vi "QUIZ#2.vi"() -> ()   [LabVIEW 2020]
uses:
  <vilib>/Utility/miscctls.llb/LVBoundsTypeDef.ctl
  <vilib>/Utility/miscctls.llb/LVPositionTypeDef.ctl
  Control 2.ctl
panel:
  out "String":string
  out "DISCO 6":bool
  out "Numeric 2":dbl
  out "x-y":ext
  in  "Array":dbl[](array[numeric])
  out "Bounds 4":T1
  out "x*y 2":u32
  in  "NUMERO DISCOS":T2
  out "Position 5":T3
  out "Position 4":T3
  out "Position 3":T3
  out "Position 2":T3
  out "Position":T3
  out "DISCO 1":bool
  out "DISCO 2":bool
  in  "Boolean 2":bool
  in  "Boolean":bool
  in  "s 2":bool
  out "Bounds 3":T1
  out "DISCO 3":bool
  out "DISCO 4":bool
  out "Bounds":T1
  in  "s":bool
  out "DISCO 5":bool
  out "DESTINO 3":bool
  out "DESTINO":bool
  out "DESTINO 2":bool
  # "NUMERO DE DISCOS ="
  # "NUMERO DE MOVIMIENTOS MINIMOS="
  # "TU NUMERO DE MOVIMIENTOS="
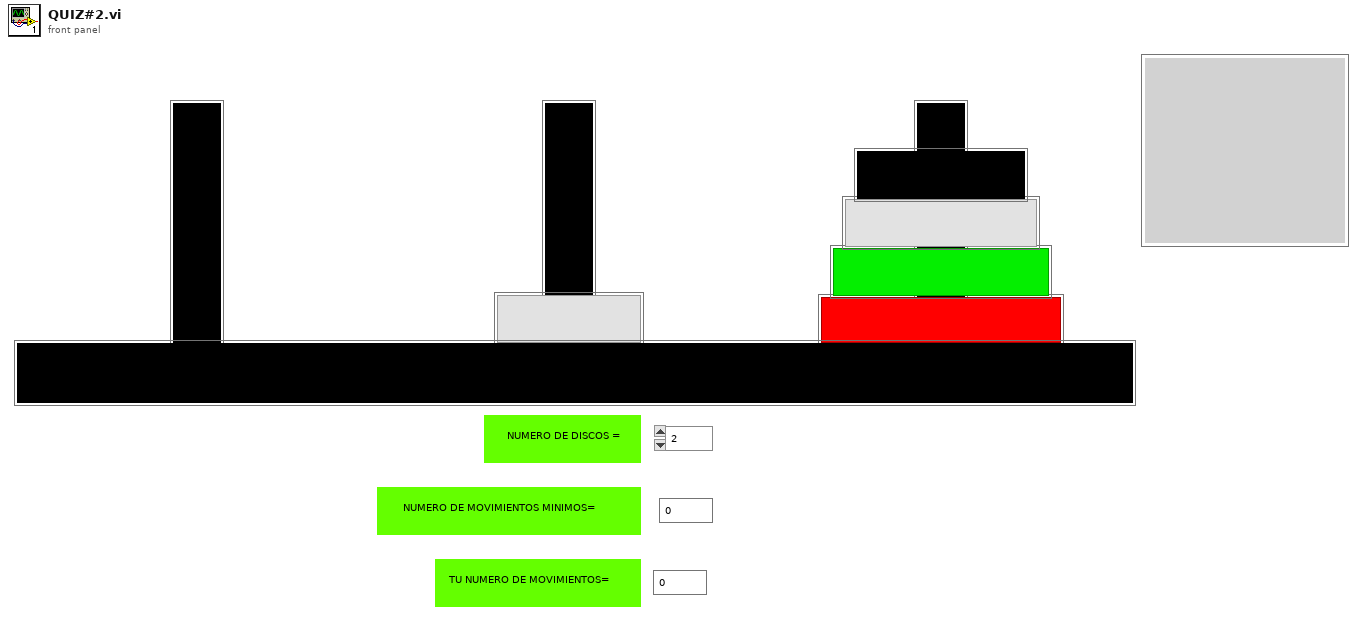
[diagram p1: front panel]
types:
  T1 = typedef "LVBoundsTypeDef.ctl" = cluster{"Width":u32, "Height":u32}
  T2 = typedef "Control 2.ctl" = enum16{"2", "3", "4", "5"}
  T3 = typedef "LVPositionTypeDef.ctl" = cluster{"Left":i32, "Top":i32}
  T4 = typedef "LVPoint32TypeDef.ctl" = cluster{"Horizontal":i32, "Vertical":i32}
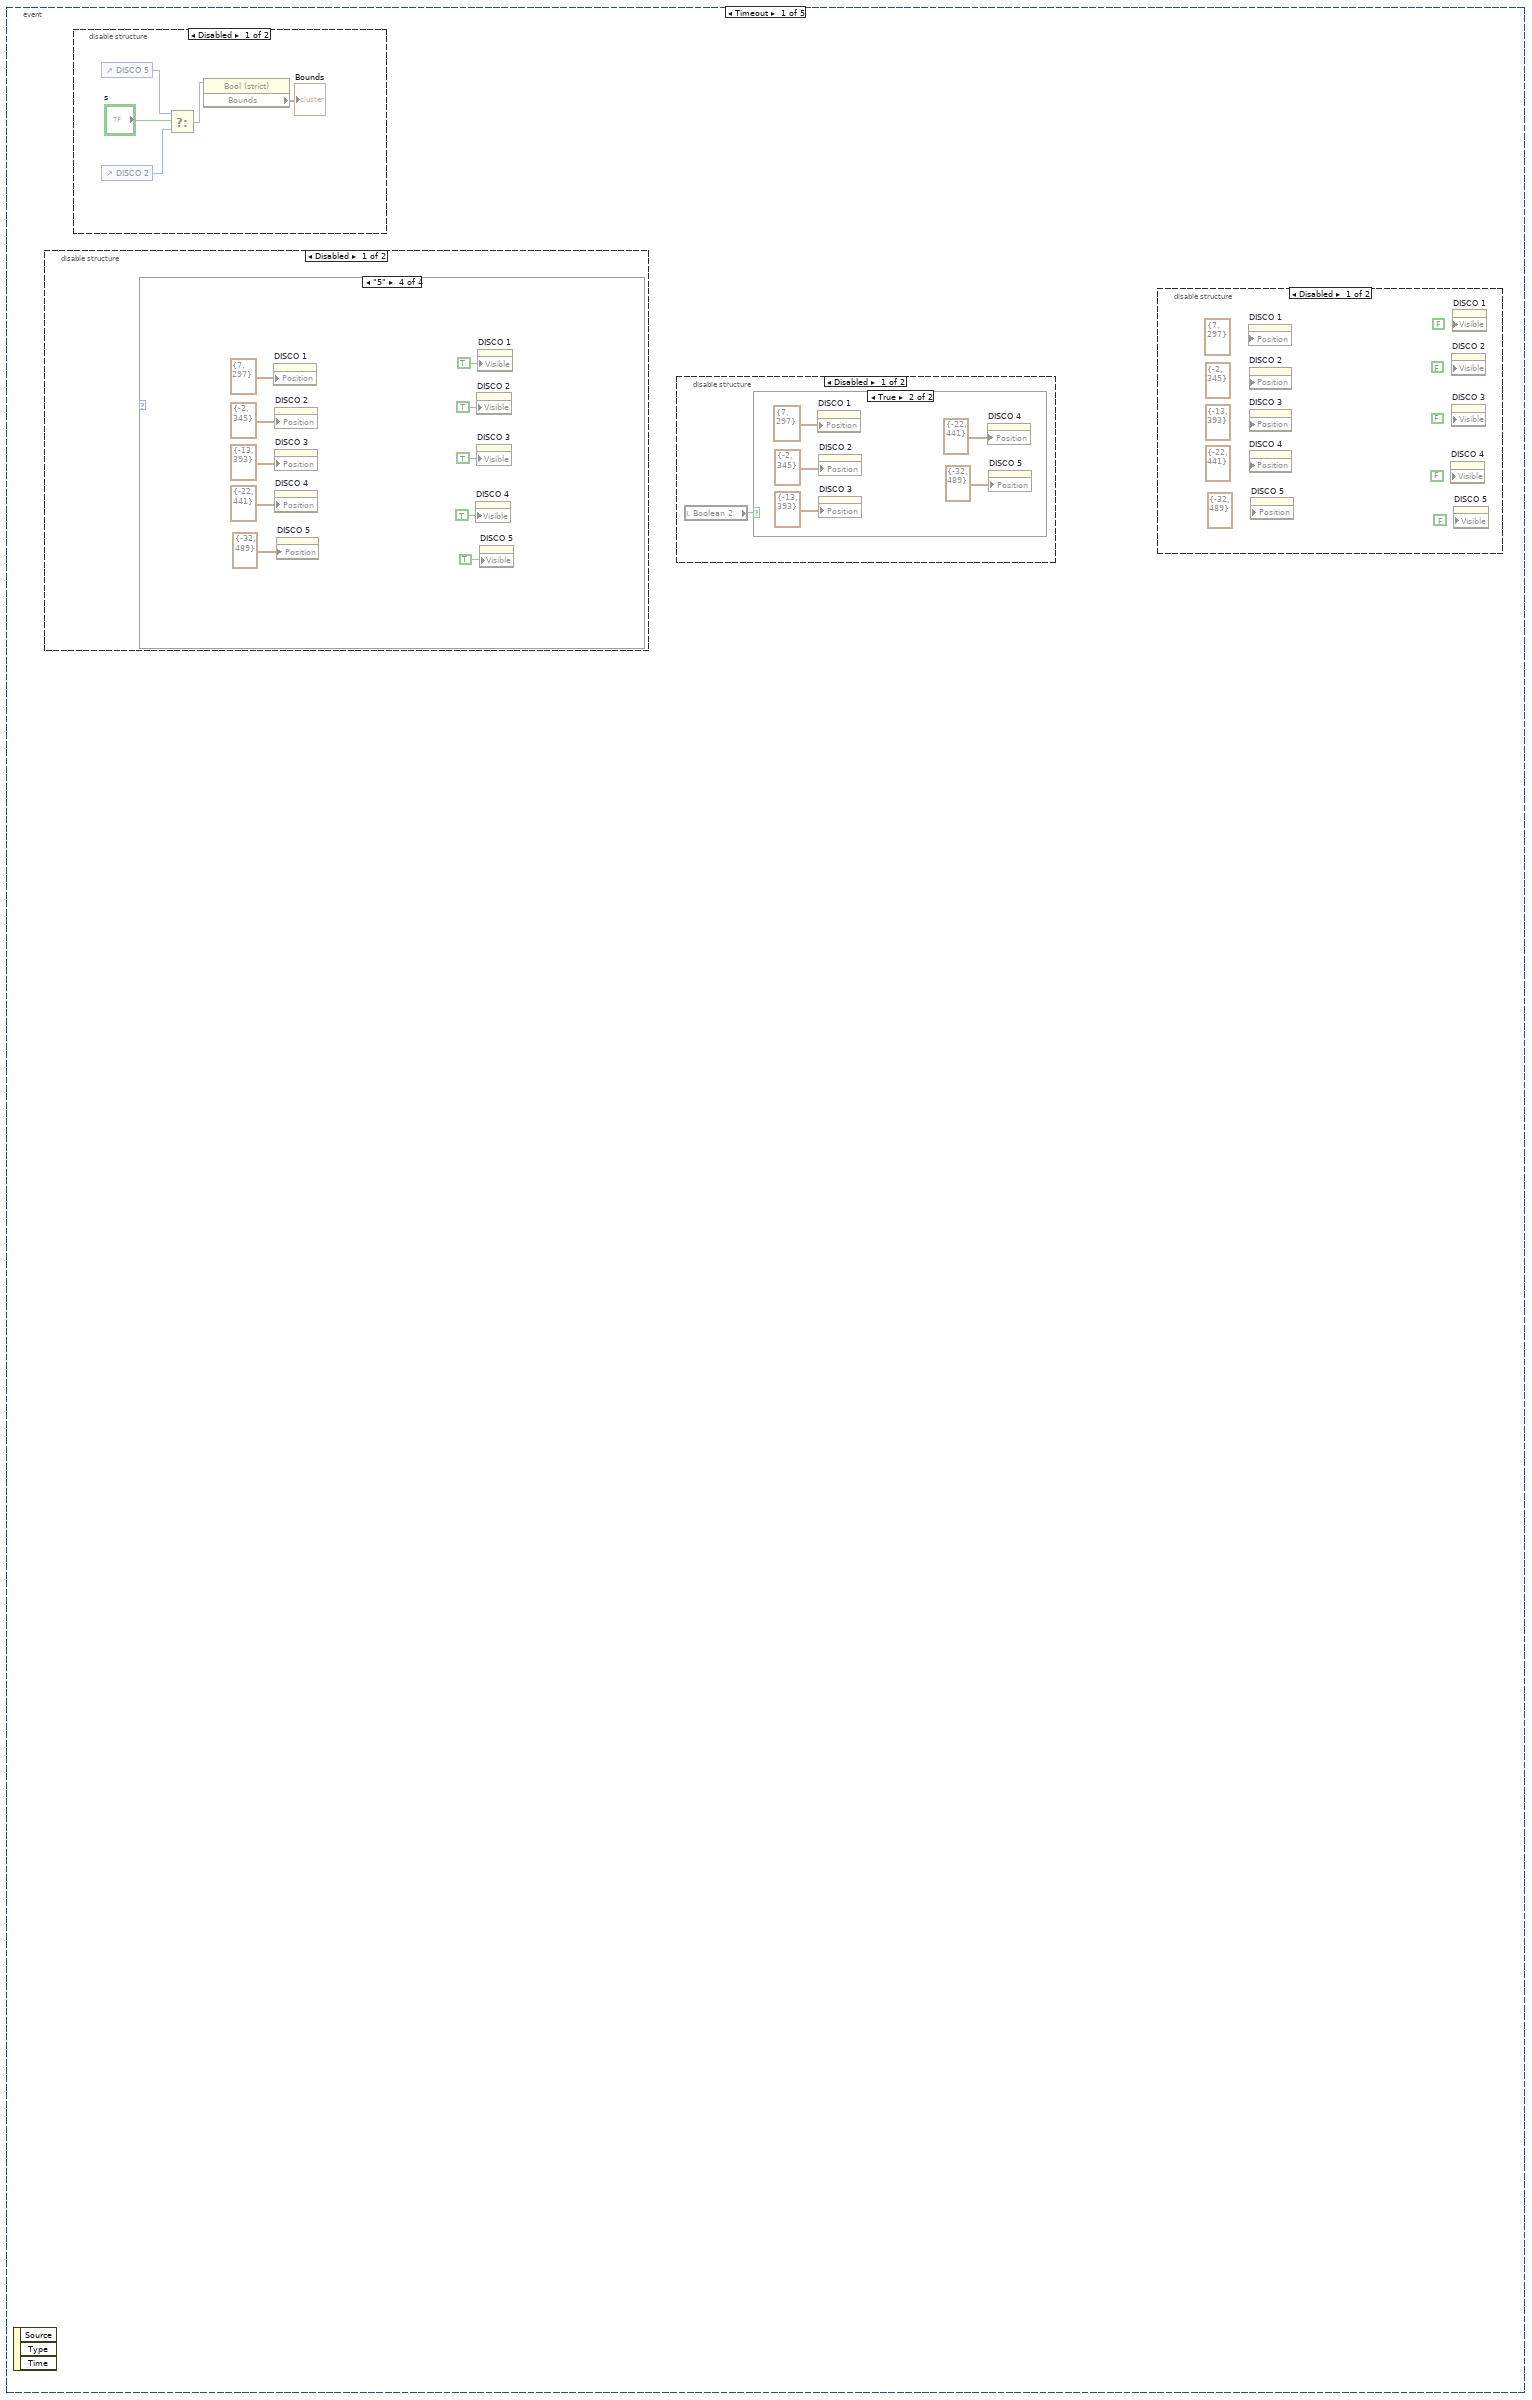
[diagram p7: hidden frame]
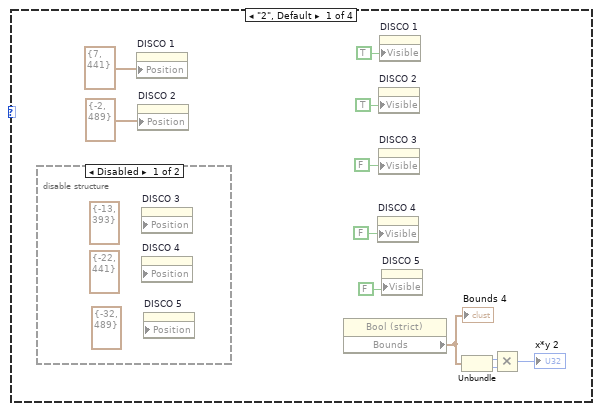
[diagram p9: hidden frame]
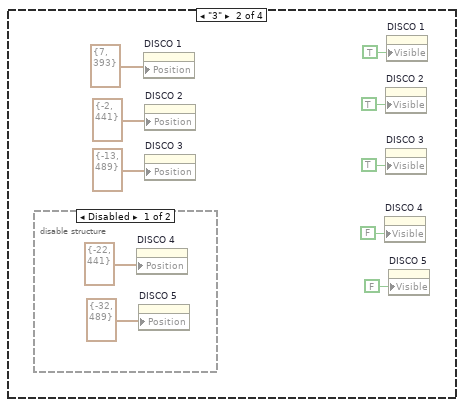
[diagram p11: hidden frame]
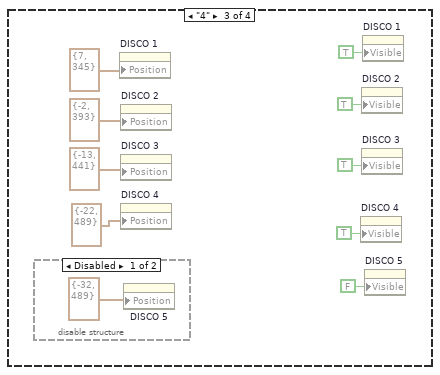
[diagram p13: hidden frame]
diagram:
  (unwired) Control_2."2"
  n1 = disable-structure shown="Disabled" {
    frame Disabled {
      n2 = property on="DISCO 1" class="Bool (strict)"() -> ("Position"=→"Position":T3)  [unwired: 2 in, 2 out]
      n3 = property on="DISCO 2" class="Bool (strict)"() -> ("Position"=→"Position 2":T3)  [unwired: 2 in, 2 out]
      n4 = property on="DISCO 3" class="Bool (strict)"() -> ("Position"=→"Position 3":T3)  [unwired: 2 in, 2 out]
      n5 = property on="DISCO 4" class="Bool (strict)"() -> ("Position"=→"Position 4":T3)  [unwired: 2 in, 2 out]
      n6 = property on="DISCO 5" class="Bool (strict)"() -> ("Position"=→"Position 5":T3)  [unwired: 2 in, 2 out]
      n7 = property on="DISCO 1" class="Bool (strict)"("Position"=T3 {"Left"=381, "Top"=297}) -> ()  [unwired: 2 in, 2 out]
      n8 = property on="DISCO 2" class="Bool (strict)"("Position"=T3 {"Left"=369, "Top"=345}) -> ()  [unwired: 2 in, 2 out]
      n9 = property on="DISCO 3" class="Bool (strict)"("Position"=T3 {"Left"=357, "Top"=393}) -> ()  [unwired: 2 in, 2 out]
      n10 = property on="DISCO 4" class="Bool (strict)"("Position"=T3 {"Left"=345, "Top"=441}) -> ()  [unwired: 2 in, 2 out]
      n11 = property on="DISCO 5" class="Bool (strict)"("Position"=T3 {"Left"=333, "Top"=489}) -> ()  [unwired: 2 in, 2 out]
    }
    frame Enabled {
    }
  }
  n12 = while {
    stop <- FALSE stop-if-true
    n13 = event shown="[1] \"DISCO 1\", \"DISCO 2\", \"DISCO 5\", \"DISCO 4\", \"DISCO 3\", \"DESTINO 3\", \"DESTINO 2\", \"DESTINO\": Mouse Up" {
      selector: _ -> [_ _ _ _ _]
      dyn-events: _ -> [_ _ _ _ _]
      timeout: 100 -> [_ _ _ _ _]
      event Timeout {
        n14 = event-data() -> ()  [unwired: 1 in, 3 out]
        n15 = disable-structure shown="Disabled" {
          frame Disabled {
            n16 = case shown="\"5\"" w14 {
              frame "2", Default {
                n17 = disable-structure shown="Disabled" {
                  frame Disabled {
                    (unwired) T3 {"Left"=-32, "Top"=489} ("Position")
                    (unwired) T3 {"Left"=-22, "Top"=441} ("Position")
                    (unwired) T3 {"Left"=-13, "Top"=393} ("Position")
                    n18 = property on="DISCO 3" class="Bool (strict)" props=["Position"]() -> ()  [unwired: 3 in, 2 out]
                    n19 = property on="DISCO 4" class="Bool (strict)" props=["Position"]() -> ()  [unwired: 3 in, 2 out]
                    n20 = property on="DISCO 5" class="Bool (strict)" props=["Position"]() -> ()  [unwired: 3 in, 2 out]
                  }
                  frame Enabled {
                  }
                }
                n21 = property on="DISCO 1" class="Bool (strict)"("Position"=T3 {"Left"=7, "Top"=441}) -> ()  [unwired: 2 in, 2 out]
                n22 = property on="DISCO 2" class="Bool (strict)"("Position"=T3 {"Left"=-2, "Top"=489}) -> ()  [unwired: 2 in, 2 out]
                n23 = property class="Bool (strict)"() -> ("Bounds"=w18:T1)  [unwired: 2 in, 2 out]
                "Bounds 4" <- w18
                n24 = property on="DISCO 4" class="Bool (strict)"("Visible"=FALSE) -> ()  [unwired: 2 in, 2 out]
                n25 = property on="DISCO 2" class="Bool (strict)"("Visible"=TRUE) -> ()  [unwired: 2 in, 2 out]
                n26 = property on="DISCO 3" class="Bool (strict)"("Visible"=FALSE) -> ()  [unwired: 2 in, 2 out]
                n27 = property on="DISCO 1" class="Bool (strict)"("Visible"=TRUE) -> ()  [unwired: 2 in, 2 out]
                n28 = property on="DISCO 5" class="Bool (strict)"("Visible"=FALSE) -> ()  [unwired: 2 in, 2 out]
                n29 = Unbundle(w18) -> ("Width"=w16:u32, "Height"=w15:u32)
                n30 = Multiply(x=w16, y=w15) -> (x*y=→"x*y 2":u32)
              }
              frame "3" {
                n31 = disable-structure shown="Disabled" {
                  frame Disabled {
                    n32 = property on="DISCO 4" class="Bool (strict)"("Position"=T3 {"Left"=-22, "Top"=441}) -> ()  [unwired: 2 in, 2 out]
                    n33 = property on="DISCO 5" class="Bool (strict)"("Position"=T3 {"Left"=-32, "Top"=489}) -> ()  [unwired: 2 in, 2 out]
                  }
                  frame Enabled {
                  }
                }
                n34 = property on="DISCO 1" class="Bool (strict)"("Position"=T3 {"Left"=7, "Top"=393}) -> ()  [unwired: 2 in, 2 out]
                n35 = property on="DISCO 2" class="Bool (strict)"("Position"=T3 {"Left"=-2, "Top"=441}) -> ()  [unwired: 2 in, 2 out]
                n36 = property on="DISCO 3" class="Bool (strict)"("Position"=T3 {"Left"=-13, "Top"=489}) -> ()  [unwired: 2 in, 2 out]
                n37 = property on="DISCO 4" class="Bool (strict)"("Visible"=FALSE) -> ()  [unwired: 2 in, 2 out]
                n38 = property on="DISCO 2" class="Bool (strict)"("Visible"=TRUE) -> ()  [unwired: 2 in, 2 out]
                n39 = property on="DISCO 3" class="Bool (strict)"("Visible"=TRUE) -> ()  [unwired: 2 in, 2 out]
                n40 = property on="DISCO 1" class="Bool (strict)"("Visible"=TRUE) -> ()  [unwired: 2 in, 2 out]
                n41 = property on="DISCO 5" class="Bool (strict)"("Visible"=FALSE) -> ()  [unwired: 2 in, 2 out]
              }
              frame "4" {
                n42 = disable-structure shown="Disabled" {
                  frame Disabled {
                    n43 = property on="DISCO 5" class="Bool (strict)"("Position"=T3 {"Left"=-32, "Top"=489}) -> ()  [unwired: 2 in, 2 out]
                  }
                  frame Enabled {
                  }
                }
                n44 = property on="DISCO 1" class="Bool (strict)"("Position"=T3 {"Left"=7, "Top"=345}) -> ()  [unwired: 2 in, 2 out]
                n45 = property on="DISCO 2" class="Bool (strict)"("Position"=T3 {"Left"=-2, "Top"=393}) -> ()  [unwired: 2 in, 2 out]
                n46 = property on="DISCO 3" class="Bool (strict)"("Position"=T3 {"Left"=-13, "Top"=441}) -> ()  [unwired: 2 in, 2 out]
                n47 = property on="DISCO 4" class="Bool (strict)"("Position"=T3 {"Left"=-22, "Top"=489}) -> ()  [unwired: 2 in, 2 out]
                n48 = property on="DISCO 4" class="Bool (strict)"("Visible"=TRUE) -> ()  [unwired: 2 in, 2 out]
                n49 = property on="DISCO 2" class="Bool (strict)"("Visible"=TRUE) -> ()  [unwired: 2 in, 2 out]
                n50 = property on="DISCO 3" class="Bool (strict)"("Visible"=TRUE) -> ()  [unwired: 2 in, 2 out]
                n51 = property on="DISCO 1" class="Bool (strict)"("Visible"=TRUE) -> ()  [unwired: 2 in, 2 out]
                n52 = property on="DISCO 5" class="Bool (strict)"("Visible"=FALSE) -> ()  [unwired: 2 in, 2 out]
              }
              frame "5" {
                n53 = property on="DISCO 1" class="Bool (strict)"("Position"=T3 {"Left"=7, "Top"=297}) -> ()  [unwired: 2 in, 2 out]
                n54 = property on="DISCO 2" class="Bool (strict)"("Position"=T3 {"Left"=-2, "Top"=345}) -> ()  [unwired: 2 in, 2 out]
                n55 = property on="DISCO 3" class="Bool (strict)"("Position"=T3 {"Left"=-13, "Top"=393}) -> ()  [unwired: 2 in, 2 out]
                n56 = property on="DISCO 4" class="Bool (strict)"("Position"=T3 {"Left"=-22, "Top"=441}) -> ()  [unwired: 2 in, 2 out]
                n57 = property on="DISCO 5" class="Bool (strict)"("Position"=T3 {"Left"=-32, "Top"=489}) -> ()  [unwired: 2 in, 2 out]
                n58 = property on="DISCO 4" class="Bool (strict)"("Visible"=TRUE) -> ()  [unwired: 2 in, 2 out]
                n59 = property on="DISCO 2" class="Bool (strict)"("Visible"=TRUE) -> ()  [unwired: 2 in, 2 out]
                n60 = property on="DISCO 3" class="Bool (strict)"("Visible"=TRUE) -> ()  [unwired: 2 in, 2 out]
                n61 = property on="DISCO 1" class="Bool (strict)"("Visible"=TRUE) -> ()  [unwired: 2 in, 2 out]
                n62 = property on="DISCO 5" class="Bool (strict)"("Visible"=TRUE) -> ()  [unwired: 2 in, 2 out]
              }
            }
          }
          frame Enabled {
          }
        }
        n63 = disable-structure shown="Disabled" {
          frame Disabled {
            n64 = control-ref of="DISCO 5"() -> (w66:refnum<vi>)
            n65 = control-ref of="DISCO 2"() -> (w65:refnum<vi>)
            n66 = Select(t=w66, s="s", f=w65) -> (s? t:f=w64:refnum<vi>)
            n67 = property on="Property Node" class="Bool (strict)"(reference=w64) -> ("Bounds"=→"Bounds":T1)  [unwired: 1 in, 2 out]
          }
          frame Enabled {
          }
        }
        n68 = disable-structure shown="Disabled" {
          frame Disabled {
            n69 = local read "Boolean 2"() -> (w56:bool)
            n70 = case shown="True" w56 {
              frame False {
              }
              frame True {
                n71 = property on="DISCO 1" class="Bool (strict)"("Position"=T3 {"Left"=7, "Top"=297}) -> ()  [unwired: 2 in, 2 out]
                n72 = property on="DISCO 2" class="Bool (strict)"("Position"=T3 {"Left"=-2, "Top"=345}) -> ()  [unwired: 2 in, 2 out]
                n73 = property on="DISCO 3" class="Bool (strict)"("Position"=T3 {"Left"=-13, "Top"=393}) -> ()  [unwired: 2 in, 2 out]
                n74 = property on="DISCO 4" class="Bool (strict)"("Position"=T3 {"Left"=-22, "Top"=441}) -> ()  [unwired: 2 in, 2 out]
                n75 = property on="DISCO 5" class="Bool (strict)"("Position"=T3 {"Left"=-32, "Top"=489}) -> ()  [unwired: 2 in, 2 out]
              }
            }
          }
          frame Enabled {
          }
        }
        n76 = disable-structure shown="Disabled" {
          frame Disabled {
            (unwired) FALSE ("Visible")
            (unwired) FALSE ("Visible")
            (unwired) FALSE ("Visible")
            (unwired) FALSE ("Visible")
            (unwired) FALSE ("Visible")
            (unwired) T3 {"Left"=-32, "Top"=489} ("Position")
            (unwired) T3 {"Left"=-22, "Top"=441} ("Position")
            (unwired) T3 {"Left"=-13, "Top"=393} ("Position")
            (unwired) T3 {"Left"=-2, "Top"=345} ("Position")
            (unwired) T3 {"Left"=7, "Top"=297} ("Position")
            n77 = property on="DISCO 1" class="Bool (strict)" props=["Position"]() -> ()  [unwired: 3 in, 2 out]
            n78 = property on="DISCO 2" class="Bool (strict)" props=["Position"]() -> ()  [unwired: 3 in, 2 out]
            n79 = property on="DISCO 3" class="Bool (strict)" props=["Position"]() -> ()  [unwired: 3 in, 2 out]
            n80 = property on="DISCO 4" class="Bool (strict)" props=["Position"]() -> ()  [unwired: 3 in, 2 out]
            n81 = property on="DISCO 5" class="Bool (strict)" props=["Position"]() -> ()  [unwired: 3 in, 2 out]
            n82 = property on="DISCO 4" class="Bool (strict)" props=["Visible"]() -> ()  [unwired: 3 in, 2 out]
            n83 = property on="DISCO 2" class="Bool (strict)" props=["Visible"]() -> ()  [unwired: 3 in, 2 out]
            n84 = property on="DISCO 3" class="Bool (strict)" props=["Visible"]() -> ()  [unwired: 3 in, 2 out]
            n85 = property on="DISCO 1" class="Bool (strict)" props=["Visible"]() -> ()  [unwired: 3 in, 2 out]
            n86 = property on="DISCO 5" class="Bool (strict)" props=["Visible"]() -> ()  [unwired: 3 in, 2 out]
          }
          frame Enabled {
          }
        }
      }
      event "DISCO 1", "DISCO 2", "DISCO 5", "DISCO 4", "DISCO 3", "DESTINO 3", "DESTINO 2", "DESTINO": Mouse Up {
        (unwired) 0 ("x")
        (unwired) 345 ("y")
        n87 = event-data() -> ()  [unwired: 1 in, 6 out]
        n88 = property on="DISCO 3" class="Bool (strict)"() -> ("Left"=w2294:i32, "Top"=w2302:i32)  [unwired: 2 in, 2 out]
        n89 = property on="DISCO 3" class="Bool (strict)"() -> ("Left"=w2311:i32, "Top"=w2303:i32)  [unwired: 2 in, 2 out]
        n90 = property on="DISCO 3" class="Bool (strict)"() -> ("Left"=w2320:i32, "Top"=w2328:i32)  [unwired: 2 in, 2 out]
        n91 = property on="DISCO 3" class="Bool (strict)"() -> ("Left"=w2337:i32, "Top"=w2329:i32)  [unwired: 2 in, 2 out]
        n92 = property on="DISCO 3" class="Bool (strict)"() -> ("Left"=w2346:i32, "Top"=w2354:i32)  [unwired: 2 in, 2 out]
        n93 = property on="DISCO 5" class="Bool (strict)"() -> ("Left"=w2415:i32, "Top"=w2407:i32)  [unwired: 2 in, 2 out]
        n94 = property on="DISCO 5" class="Bool (strict)"() -> ("Left"=w2398:i32, "Top"=w2406:i32)  [unwired: 2 in, 2 out]
        n95 = property on="DISCO 5" class="Bool (strict)"() -> ("Left"=w2389:i32, "Top"=w2381:i32)  [unwired: 2 in, 2 out]
        n96 = property on="DISCO 5" class="Bool (strict)"() -> ("Left"=w2372:i32, "Top"=w2380:i32)  [unwired: 2 in, 2 out]
        n97 = property on="DISCO 5" class="Bool (strict)"() -> ("Left"=w2363:i32, "Top"=w2355:i32)  [unwired: 2 in, 2 out]
        n98 = property on="DISCO 5" class="Bool (strict)"() -> ("Left"=w2424:i32, "Top"=w2432:i32)  [unwired: 2 in, 2 out]
        n99 = local write "Boolean"(FALSE ("Boolean 2")) -> ()
        n100 = property on="DISCO 5" class="Bool (strict)"() -> ("Left"=w2441:i32, "Top"=w2433:i32)  [unwired: 2 in, 2 out]
        n101 = property on="DISCO 5" class="Bool (strict)"() -> ("Left"=w2467:i32, "Top"=w2459:i32)  [unwired: 2 in, 2 out]
        n102 = property on="DISCO 5" class="Bool (strict)"() -> ("Left"=w2476:i32, "Top"=w2484:i32)  [unwired: 2 in, 2 out]
        n103 = property on="DISCO 3" class="Bool (strict)"() -> ("Left"=w1765:i32, "Top"=w1757:i32)  [unwired: 2 in, 2 out]
        n104 = property on="DISCO 5" class="Bool (strict)"() -> ("Left"=w2450:i32, "Top"=w2458:i32)  [unwired: 2 in, 2 out]
        n105 = property on="DISCO 1" class="Bool (strict)"() -> ("Left"=w2208:i32, "Top"=w2200:i32)  [unwired: 2 in, 2 out]
        n106 = property on="DISCO 1" class="Bool (strict)"() -> ("Left"=w2217:i32, "Top"=w2225:i32)  [unwired: 2 in, 2 out]
        n107 = property on="DISCO 3" class="Bool (strict)"() -> ("Left"=w1748:i32, "Top"=w1756:i32)  [unwired: 2 in, 2 out]
        n108 = property on="DISCO 3" class="Bool (strict)"() -> ("Left"=w1739:i32, "Top"=w1731:i32)  [unwired: 2 in, 2 out]
        n109 = property on="DISCO 3" class="Bool (strict)"() -> ("Left"=w1722:i32, "Top"=w1730:i32)  [unwired: 2 in, 2 out]
        n110 = property on="DISCO 3" class="Bool (strict)"() -> ("Left"=w1713:i32, "Top"=w1705:i32)  [unwired: 2 in, 2 out]
        n111 = property on="DISCO 1" class="Bool (strict)"() -> ("Left"=w2165:i32, "Top"=w2173:i32)  [unwired: 2 in, 2 out]
        n112 = property on="DISCO 1" class="Bool (strict)"() -> ("Left"=w2182:i32, "Top"=w2174:i32)  [unwired: 2 in, 2 out]
        n113 = property on="DISCO 1" class="Bool (strict)"() -> ("Left"=w2191:i32, "Top"=w2199:i32)  [unwired: 2 in, 2 out]
        n114 = Greater Or Equal?(x=w2372, y=700) -> (x >= y?=w2370:bool)
        n115 = Less Or Equal?(x=w2372, y=900) -> (x <= y?=w2371:bool)
        n116 = Greater Or Equal?(x=w2380, y=297) -> (x >= y?=w2374:bool)
        n117 = Less Or Equal?(x=w2380, y=345) -> (x <= y?=w2373:bool)
        n118 = Greater Or Equal?(x=w2363, y=700) -> (x >= y?=w2365:bool)
        n119 = Less Or Equal?(x=w2363, y=900) -> (x <= y?=w2364:bool)
        n120 = Greater Or Equal?(x=w2355, y=240) -> (x >= y?=w2361:bool)
        n121 = Less Or Equal?(x=w2355, y=297) -> (x <= y?=w2362:bool)
        n122 = Greater Or Equal?(x=w2337, y=700) -> (x >= y?=w2339:bool)
        n123 = Less Or Equal?(x=w2337, y=900) -> (x <= y?=w2338:bool)
        n124 = Greater Or Equal?(x=w2329, y=297) -> (x >= y?=w2335:bool)
        n125 = Less Or Equal?(x=w2329, y=345) -> (x <= y?=w2336:bool)
        n126 = Greater Or Equal?(x=w2346, y=700) -> (x >= y?=w2344:bool)
        n127 = Less Or Equal?(x=w2346, y=900) -> (x <= y?=w2345:bool)
        n128 = Greater Or Equal?(x=w2354, y=240) -> (x >= y?=w2348:bool)
        n129 = Less Or Equal?(x=w2354, y=297) -> (x <= y?=w2347:bool)
        n130 = property on="DISCO 1" class="Bool (strict)"() -> ("Left"=w2519:i32, "Top"=w2511:i32)  [unwired: 2 in, 2 out]
        n131 = Less Or Equal?(x=w2415, y=900) -> (x <= y?=w2416:bool)
        n132 = Greater Or Equal?(x=w2407, y=441) -> (x >= y?=w2413:bool)
        n133 = Less Or Equal?(x=w2407, y=489) -> (x <= y?=w2414:bool)
        n134 = Greater Or Equal?(x=w2398, y=700) -> (x >= y?=w2396:bool)
        n135 = Less Or Equal?(x=w2398, y=900) -> (x <= y?=w2397:bool)
        n136 = Greater Or Equal?(x=w2406, y=393) -> (x >= y?=w2400:bool)
        n137 = Less Or Equal?(x=w2406, y=441) -> (x <= y?=w2399:bool)
        n138 = Greater Or Equal?(x=w2389, y=700) -> (x >= y?=w2391:bool)
        n139 = Less Or Equal?(x=w2389, y=900) -> (x <= y?=w2390:bool)
        n140 = Greater Or Equal?(x=w2381, y=345) -> (x >= y?=w2387:bool)
        n141 = Less Or Equal?(x=w2381, y=393) -> (x <= y?=w2388:bool)
        n142 = Less Or Equal?(x=w2294, y=900) -> (x <= y?=w2293:bool)
        n143 = Greater Or Equal?(x=w2302, y=441) -> (x >= y?=w2296:bool)
        n144 = Less Or Equal?(x=w2302, y=489) -> (x <= y?=w2295:bool)
        n145 = Greater Or Equal?(x=w2311, y=700) -> (x >= y?=w2313:bool)
        n146 = Less Or Equal?(x=w2311, y=900) -> (x <= y?=w2312:bool)
        n147 = Greater Or Equal?(x=w2303, y=393) -> (x >= y?=w2309:bool)
        n148 = Less Or Equal?(x=w2303, y=441) -> (x <= y?=w2310:bool)
        n149 = Greater Or Equal?(x=w2320, y=700) -> (x >= y?=w2318:bool)
        n150 = Less Or Equal?(x=w2320, y=900) -> (x <= y?=w2319:bool)
        n151 = Greater Or Equal?(x=w2328, y=345) -> (x >= y?=w2322:bool)
        n152 = Less Or Equal?(x=w2328, y=393) -> (x <= y?=w2321:bool)
        n153 = Greater Or Equal?(x=w2415, y=700) -> (x >= y?=w2417:bool)
        n154 = Greater Or Equal?(x=w2294, y=700) -> (x >= y?=w2292:bool)
        n155 = property on="DISCO 1" class="Bool (strict)"() -> ("Left"=w1696:i32, "Top"=w1704:i32)  [unwired: 2 in, 2 out]
        n156 = property on="DISCO 1" class="Bool (strict)"() -> ("Left"=w1687:i32, "Top"=w1679:i32)  [unwired: 2 in, 2 out]
        n157 = property on="DISCO 1" class="Bool (strict)"() -> ("Left"=w2503:i32, "Top"=w2510:i32)  [unwired: 2 in, 2 out]
        n158 = property on="DISCO 1" class="Bool (strict)"() -> ("Left"=w2493:i32, "Top"=w2485:i32)  [unwired: 2 in, 2 out]
        n159 = And(x=w2370, y=w2371) -> (x .and. y?=w2377:bool)
        n160 = And(x=w2374, y=w2373) -> (x .and. y?=w2378:bool)
        n161 = And(x=w2365, y=w2364) -> (x .and. y?=w2358:bool)
        n162 = And(x=w2361, y=w2362) -> (x .and. y?=w2357:bool)
        n163 = And(x=w2339, y=w2338) -> (x .and. y?=w2332:bool)
        n164 = And(x=w2335, y=w2336) -> (x .and. y?=w2331:bool)
        n165 = And(x=w2344, y=w2345) -> (x .and. y?=w2351:bool)
        n166 = And(x=w2348, y=w2347) -> (x .and. y?=w2352:bool)
        n167 = Less Or Equal?(x=w1730, y=345) -> (x <= y?=w1723:bool)
        n168 = Greater Or Equal?(x=w2467, y=350) -> (x >= y?=w2469:bool)
        n169 = Less Or Equal?(x=w2467, y=500) -> (x <= y?=w2468:bool)
        n170 = Greater Or Equal?(x=w2459, y=297) -> (x >= y?=w2465:bool)
        n171 = Less Or Equal?(x=w2459, y=345) -> (x <= y?=w2466:bool)
        n172 = And(x=w2417, y=w2416) -> (x .and. y?=w2410:bool)
        n173 = And(x=w2413, y=w2414) -> (x .and. y?=w2409:bool)
        n174 = And(x=w2396, y=w2397) -> (x .and. y?=w2403:bool)
        n175 = And(x=w2400, y=w2399) -> (x .and. y?=w2404:bool)
        n176 = And(x=w2391, y=w2390) -> (x .and. y?=w2384:bool)
        n177 = And(x=w2387, y=w2388) -> (x .and. y?=w2383:bool)
        n178 = Greater Or Equal?(x=w2476, y=350) -> (x >= y?=w2474:bool)
        n179 = Less Or Equal?(x=w2476, y=500) -> (x <= y?=w2475:bool)
        n180 = Greater Or Equal?(x=w2484, y=240) -> (x >= y?=w2478:bool)
        n181 = Greater Or Equal?(x=w1722, y=350) -> (x >= y?=w1720:bool)
        n182 = Less Or Equal?(x=w1722, y=500) -> (x <= y?=w1721:bool)
        n183 = Greater Or Equal?(x=w1730, y=297) -> (x >= y?=w1724:bool)
        n184 = And(x=w2292, y=w2293) -> (x .and. y?=w2299:bool)
        n185 = And(x=w2296, y=w2295) -> (x .and. y?=w2300:bool)
        n186 = And(x=w2313, y=w2312) -> (x .and. y?=w2306:bool)
        n187 = And(x=w2309, y=w2310) -> (x .and. y?=w2305:bool)
        n188 = And(x=w2318, y=w2319) -> (x .and. y?=w2325:bool)
        n189 = And(x=w2322, y=w2321) -> (x .and. y?=w2326:bool)
        n190 = Greater Or Equal?(x=w1713, y=350) -> (x >= y?=w1715:bool)
        n191 = Less Or Equal?(x=w1713, y=500) -> (x <= y?=w1714:bool)
        n192 = Greater Or Equal?(x=w1705, y=240) -> (x >= y?=w1711:bool)
        n193 = Less Or Equal?(x=w1705, y=297) -> (x <= y?=w1712:bool)
        n194 = Less Or Equal?(x=w2484, y=297) -> (x <= y?=w2477:bool)
        n195 = Less Or Equal?(x=w2424, y=500) -> (x <= y?=w2423:bool)
        n196 = Greater Or Equal?(x=w2432, y=441) -> (x >= y?=w2426:bool)
        n197 = Less Or Equal?(x=w2432, y=489) -> (x <= y?=w2425:bool)
        n198 = Greater Or Equal?(x=w2441, y=350) -> (x >= y?=w2443:bool)
        n199 = Less Or Equal?(x=w2441, y=500) -> (x <= y?=w2442:bool)
        n200 = Greater Or Equal?(x=w2433, y=393) -> (x >= y?=w2439:bool)
        n201 = Less Or Equal?(x=w2433, y=441) -> (x <= y?=w2440:bool)
        n202 = Greater Or Equal?(x=w2450, y=350) -> (x >= y?=w2448:bool)
        n203 = Less Or Equal?(x=w2450, y=500) -> (x <= y?=w2449:bool)
        n204 = Greater Or Equal?(x=w2458, y=345) -> (x >= y?=w2452:bool)
        n205 = Less Or Equal?(x=w2458, y=393) -> (x <= y?=w2451:bool)
        n206 = Less Or Equal?(x=w1756, y=441) -> (x <= y?=w1749:bool)
        n207 = Less Or Equal?(x=w1765, y=500) -> (x <= y?=w1766:bool)
        n208 = Greater Or Equal?(x=w1757, y=441) -> (x >= y?=w1763:bool)
        n209 = Less Or Equal?(x=w1757, y=489) -> (x <= y?=w1764:bool)
        n210 = Greater Or Equal?(x=w1748, y=350) -> (x >= y?=w1746:bool)
        n211 = Less Or Equal?(x=w1748, y=500) -> (x <= y?=w1747:bool)
        n212 = Greater Or Equal?(x=w1756, y=393) -> (x >= y?=w1750:bool)
        n213 = Greater Or Equal?(x=w1739, y=350) -> (x >= y?=w1741:bool)
        n214 = Less Or Equal?(x=w1739, y=500) -> (x <= y?=w1740:bool)
        n215 = Greater Or Equal?(x=w1731, y=345) -> (x >= y?=w1737:bool)
        n216 = Less Or Equal?(x=w1731, y=393) -> (x <= y?=w1738:bool)
        n217 = Greater Or Equal?(x=w2424, y=350) -> (x >= y?=w2422:bool)
        n218 = Greater Or Equal?(x=w1765, y=350) -> (x >= y?=w1767:bool)
        n219 = Greater Or Equal?(x=w2208, y=700) -> (x >= y?=w2210:bool)
        n220 = Less Or Equal?(x=w2208, y=900) -> (x <= y?=w2209:bool)
        n221 = Greater Or Equal?(x=w2200, y=297) -> (x >= y?=w2206:bool)
        n222 = Less Or Equal?(x=w2200, y=345) -> (x <= y?=w2207:bool)
        n223 = And(x=w2377, y=w2378) -> (x .and. y?=w2379:bool)
        n224 = Greater Or Equal?(x=w2217, y=700) -> (x >= y?=w2215:bool)
        n225 = Less Or Equal?(x=w2217, y=900) -> (x <= y?=w2216:bool)
        n226 = Greater Or Equal?(x=w2225, y=240) -> (x >= y?=w2219:bool)
        n227 = Less Or Equal?(x=w2225, y=297) -> (x <= y?=w2218:bool)
        n228 = And(x=w2358, y=w2357) -> (x .and. y?=w2356:bool)
        n229 = And(x=w2332, y=w2331) -> (x .and. y?=w2330:bool)
        n230 = And(x=w2351, y=w2352) -> (x .and. y?=w2353:bool)
        n231 = And(x=w2469, y=w2468) -> (x .and. y?=w2462:bool)
        n232 = And(x=w2465, y=w2466) -> (x .and. y?=w2461:bool)
        n233 = And(x=w2474, y=w2475) -> (x .and. y?=w2481:bool)
        n234 = And(x=w2478, y=w2477) -> (x .and. y?=w2482:bool)
        n235 = Greater Or Equal?(x=w2165, y=700) -> (x >= y?=w2163:bool)
        n236 = Less Or Equal?(x=w2165, y=900) -> (x <= y?=w2164:bool)
        n237 = Greater Or Equal?(x=w2173, y=441) -> (x >= y?=w2167:bool)
        n238 = Less Or Equal?(x=w2173, y=489) -> (x <= y?=w2166:bool)
        n239 = Greater Or Equal?(x=w2182, y=700) -> (x >= y?=w2184:bool)
        n240 = Less Or Equal?(x=w2182, y=900) -> (x <= y?=w2183:bool)
        n241 = Greater Or Equal?(x=w2174, y=393) -> (x >= y?=w2180:bool)
        n242 = Less Or Equal?(x=w2174, y=441) -> (x <= y?=w2181:bool)
        n243 = Greater Or Equal?(x=w2191, y=700) -> (x >= y?=w2189:bool)
        n244 = Less Or Equal?(x=w2191, y=900) -> (x <= y?=w2190:bool)
        n245 = Greater Or Equal?(x=w2199, y=345) -> (x >= y?=w2193:bool)
        n246 = Less Or Equal?(x=w2199, y=393) -> (x <= y?=w2192:bool)
        n247 = And(x=w2410, y=w2409) -> (x .and. y?=w2408:bool)
        n248 = And(x=w2403, y=w2404) -> (x .and. y?=w2405:bool)
        n249 = And(x=w2384, y=w2383) -> (x .and. y?=w2382:bool)
        n250 = And(x=w1720, y=w1721) -> (x .and. y?=w1727:bool)
        n251 = And(x=w1724, y=w1723) -> (x .and. y?=w1728:bool)
        n252 = And(x=w1715, y=w1714) -> (x .and. y?=w1708:bool)
        n253 = And(x=w1711, y=w1712) -> (x .and. y?=w1707:bool)
        n254 = And(x=w2299, y=w2300) -> (x .and. y?=w2301:bool)
        n255 = And(x=w2306, y=w2305) -> (x .and. y?=w2304:bool)
        n256 = And(x=w2325, y=w2326) -> (x .and. y?=w2327:bool)
        n257 = And(x=w2422, y=w2423) -> (x .and. y?=w2429:bool)
        n258 = And(x=w2426, y=w2425) -> (x .and. y?=w2430:bool)
        n259 = And(x=w2443, y=w2442) -> (x .and. y?=w2436:bool)
        n260 = And(x=w2439, y=w2440) -> (x .and. y?=w2435:bool)
        n261 = And(x=w2448, y=w2449) -> (x .and. y?=w2455:bool)
        n262 = And(x=w2452, y=w2451) -> (x .and. y?=w2456:bool)
        n263 = And(x=w1767, y=w1766) -> (x .and. y?=w1760:bool)
        n264 = And(x=w1763, y=w1764) -> (x .and. y?=w1759:bool)
        n265 = And(x=w1746, y=w1747) -> (x .and. y?=w1753:bool)
        n266 = And(x=w1750, y=w1749) -> (x .and. y?=w1754:bool)
        n267 = And(x=w1741, y=w1740) -> (x .and. y?=w1734:bool)
        n268 = And(x=w1737, y=w1738) -> (x .and. y?=w1733:bool)
        n269 = Greater Or Equal?(x=w2519, y=350) -> (x >= y?=w2521:bool)
        n270 = Less Or Equal?(x=w2519, y=500) -> (x <= y?=w2520:bool)
        n271 = Greater Or Equal?(x=w2511, y=441) -> (x >= y?=w2517:bool)
        n272 = Less Or Equal?(x=w1704, y=345) -> (x <= y?=w1697:bool)
        n273 = And(x=w2210, y=w2209) -> (x .and. y?=w2203:bool)
        n274 = And(x=w2206, y=w2207) -> (x .and. y?=w2202:bool)
        n275 = And(x=w2215, y=w2216) -> (x .and. y?=w2222:bool)
        n276 = And(x=w2219, y=w2218) -> (x .and. y?=w2223:bool)
        n277 = Less Or Equal?(x=w1679, y=297) -> (x <= y?=w1686:bool)
        n278 = case shown="True" w2356 {
          frame False {
          }
          frame True {
            n279 = property on="DISCO 5" class="Bool (strict)"("Position"=T3 {"Left"=705, "Top"=297}) -> ()  [unwired: 2 in, 2 out]
          }
        }
        n280 = Greater Or Equal?(x=w1696, y=350) -> (x >= y?=w1694:bool)
        n281 = Less Or Equal?(x=w1696, y=500) -> (x <= y?=w1695:bool)
        n282 = Greater Or Equal?(x=w1704, y=297) -> (x >= y?=w1698:bool)
        n283 = And(x=w2462, y=w2461) -> (x .and. y?=w2460:bool)
        n284 = And(x=w2163, y=w2164) -> (x .and. y?=w2170:bool)
        n285 = And(x=w2167, y=w2166) -> (x .and. y?=w2171:bool)
        n286 = And(x=w2184, y=w2183) -> (x .and. y?=w2177:bool)
        n287 = And(x=w2180, y=w2181) -> (x .and. y?=w2176:bool)
        n288 = And(x=w2189, y=w2190) -> (x .and. y?=w2196:bool)
        n289 = And(x=w2193, y=w2192) -> (x .and. y?=w2197:bool)
        n290 = Greater Or Equal?(x=w1687, y=350) -> (x >= y?=w1689:bool)
        n291 = Less Or Equal?(x=w1687, y=500) -> (x <= y?=w1688:bool)
        n292 = Greater Or Equal?(x=w1679, y=240) -> (x >= y?=w1685:bool)
        n293 = And(x=w2481, y=w2482) -> (x .and. y?=w2483:bool)
        n294 = case shown="True" w2353 {
          frame False {
          }
          frame True {
            n295 = property on="DISCO 3" class="Bool (strict)"("Position"=T3 {"Left"=729, "Top"=297}) -> ()  [unwired: 2 in, 2 out]
          }
        }
        n296 = case shown="True" w2379 {
          frame False {
          }
          frame True {
            n297 = property on="DISCO 5" class="Bool (strict)"("Position"=T3 {"Left"=705, "Top"=345}) -> ()  [unwired: 2 in, 2 out]
          }
        }
        n298 = Greater Or Equal?(x=w2510, y=393) -> (x >= y?=w2505:bool)
        n299 = case shown="True" w2382 {
          frame False {
          }
          frame True {
            n300 = property on="DISCO 5" class="Bool (strict)"("Position"=T3 {"Left"=705, "Top"=393}) -> ()  [unwired: 2 in, 2 out]
          }
        }
        n301 = And(x=w1727, y=w1728) -> (x .and. y?=w1729:bool)
        n302 = case shown="True" w2405 {
          frame False {
          }
          frame True {
            n303 = property on="DISCO 5" class="Bool (strict)"("Position"=T3 {"Left"=705, "Top"=441}) -> ()  [unwired: 2 in, 2 out]
          }
        }
        n304 = Less Or Equal?(x=w2510, y=441) -> (x <= y?=w2504:bool)
        n305 = And(x=w1708, y=w1707) -> (x .and. y?=w1706:bool)
        n306 = case shown="True" w2330 {
          frame False {
          }
          frame True {
            n307 = property on="DISCO 3" class="Bool (strict)"("Position"=T3 {"Left"=729, "Top"=345}) -> ()  [unwired: 2 in, 2 out]
          }
        }
        n308 = case shown="True" w2327 {
          frame False {
          }
          frame True {
            n309 = property on="DISCO 3" class="Bool (strict)"("Position"=T3 {"Left"=729, "Top"=393}) -> ()  [unwired: 2 in, 2 out]
          }
        }
        n310 = case shown="True" w2304 {
          frame False {
          }
          frame True {
            n311 = property on="DISCO 3" class="Bool (strict)"("Position"=T3 {"Left"=729, "Top"=441}) -> ()  [unwired: 2 in, 2 out]
          }
        }
        n312 = Less Or Equal?(x=w2511, y=489) -> (x <= y?=w2518:bool)
        n313 = Greater Or Equal?(x=w2503, y=350) -> (x >= y?=w2501:bool)
        n314 = Less Or Equal?(x=w2503, y=500) -> (x <= y?=w2502:bool)
        n315 = Greater Or Equal?(x=w2493, y=350) -> (x >= y?=w2495:bool)
        n316 = Less Or Equal?(x=w2493, y=500) -> (x <= y?=w2494:bool)
        n317 = Greater Or Equal?(x=w2485, y=345) -> (x >= y?=w2491:bool)
        n318 = And(x=w2429, y=w2430) -> (x .and. y?=w2431:bool)
        n319 = And(x=w2436, y=w2435) -> (x .and. y?=w2434:bool)
        n320 = And(x=w2455, y=w2456) -> (x .and. y?=w2457:bool)
        n321 = Less Or Equal?(x=w2485, y=393) -> (x <= y?=w2492:bool)
        n322 = And(x=w1760, y=w1759) -> (x .and. y?=w1758:bool)
        n323 = And(x=w1753, y=w1754) -> (x .and. y?=w1755:bool)
        n324 = And(x=w1734, y=w1733) -> (x .and. y?=w1732:bool)
        n325 = case shown="True" w2408 {
          frame False {
          }
          frame True {
            n326 = property on="DISCO 5" class="Bool (strict)"("Position"=T3 {"Left"=705, "Top"=489}) -> ()  [unwired: 2 in, 2 out]
          }
        }
        n327 = case shown="True" w2301 {
          frame False {
          }
          frame True {
            n328 = property on="DISCO 3" class="Bool (strict)"("Position"=T3 {"Left"=729, "Top"=489}) -> ()  [unwired: 2 in, 2 out]
          }
        }
        n329 = And(x=w2521, y=w2520) -> (x .and. y?=w2514:bool)
        n330 = And(x=w2517, y=w2518) -> (x .and. y?=w2513:bool)
        n331 = And(x=w2203, y=w2202) -> (x .and. y?=w2201:bool)
        n332 = And(x=w2222, y=w2223) -> (x .and. y?=w2224:bool)
        n333 = And(x=w1694, y=w1695) -> (x .and. y?=w1701:bool)
        n334 = And(x=w1698, y=w1697) -> (x .and. y?=w1702:bool)
        n335 = And(x=w1689, y=w1688) -> (x .and. y?=w1682:bool)
        n336 = And(x=w1685, y=w1686) -> (x .and. y?=w1681:bool)
        n337 = And(x=w2170, y=w2171) -> (x .and. y?=w2172:bool)
        n338 = And(x=w2177, y=w2176) -> (x .and. y?=w2175:bool)
        n339 = And(x=w2196, y=w2197) -> (x .and. y?=w2198:bool)
        n340 = And(x=w2505, y=w2504) -> (x .and. y?=w2508:bool)
        n341 = case shown="True" w2483 {
          frame False {
          }
          frame True {
            n342 = property on="DISCO 5" class="Bool (strict)"("Position"=T3 {"Left"=333, "Top"=297}) -> ()  [unwired: 2 in, 2 out]
          }
        }
        n343 = And(x=w2501, y=w2502) -> (x .and. y?=w2507:bool)
        n344 = And(x=w2495, y=w2494) -> (x .and. y?=w2488:bool)
        n345 = And(x=w2491, y=w2492) -> (x .and. y?=w2487:bool)
        n346 = case shown="True" w2460 {
          frame False {
          }
          frame True {
            n347 = property on="DISCO 5" class="Bool (strict)"("Position"=T3 {"Left"=333, "Top"=345}) -> ()  [unwired: 2 in, 2 out]
          }
        }
        n348 = case shown="True" w1729 {
          frame False {
          }
          frame True {
            n349 = property on="DISCO 3" class="Bool (strict)"("Position"=T3 {"Left"=357, "Top"=345}) -> ()  [unwired: 2 in, 2 out]
          }
        }
        n350 = case shown="True" w2457 {
          frame False {
          }
          frame True {
            n351 = property on="DISCO 5" class="Bool (strict)"("Position"=T3 {"Left"=333, "Top"=393}) -> ()  [unwired: 2 in, 2 out]
          }
        }
        n352 = case shown="True" w2434 {
          frame False {
          }
          frame True {
            n353 = property on="DISCO 5" class="Bool (strict)"("Position"=T3 {"Left"=333, "Top"=441}) -> ()  [unwired: 2 in, 2 out]
          }
        }
        n354 = case shown="True" w1706 {
          frame False {
          }
          frame True {
            n355 = property on="DISCO 3" class="Bool (strict)"("Position"=T3 {"Left"=357, "Top"=297}) -> ()  [unwired: 2 in, 2 out]
          }
        }
        n356 = case shown="True" w1755 {
          frame False {
          }
          frame True {
            n357 = property on="DISCO 3" class="Bool (strict)"("Position"=T3 {"Left"=357, "Top"=441}) -> ()  [unwired: 2 in, 2 out]
          }
        }
        n358 = And(x=w2514, y=w2513) -> (x .and. y?=w2512:bool)
        n359 = case shown="True" w2431 {
          frame False {
          }
          frame True {
            n360 = property on="DISCO 5" class="Bool (strict)"("Position"=T3 {"Left"=333, "Top"=489}) -> ()  [unwired: 2 in, 2 out]
          }
        }
        n361 = case shown="True" w1732 {
          frame False {
          }
          frame True {
            n362 = property on="DISCO 3" class="Bool (strict)"("Position"=T3 {"Left"=357, "Top"=393}) -> ()  [unwired: 2 in, 2 out]
          }
        }
        n363 = case shown="True" w1758 {
          frame False {
          }
          frame True {
            n364 = property on="DISCO 3" class="Bool (strict)"("Position"=T3 {"Left"=357, "Top"=489}) -> ()  [unwired: 2 in, 2 out]
          }
        }
        n365 = case shown="True" w2224 {
          frame False {
          }
          frame True {
            n366 = property on="DISCO 1" class="Bool (strict)"("Position"=T3 {"Left"=753, "Top"=297}) -> ()  [unwired: 2 in, 2 out]
          }
        }
        n367 = And(x=w1701, y=w1702) -> (x .and. y?=w1703:bool)
        n368 = And(x=w1682, y=w1681) -> (x .and. y?=w1680:bool)
        n369 = case shown="True" w2201 {
          frame False {
          }
          frame True {
            n370 = property on="DISCO 1" class="Bool (strict)"("Position"=T3 {"Left"=753, "Top"=345}) -> ()  [unwired: 2 in, 2 out]
          }
        }
        n371 = case shown="True" w2198 {
          frame False {
          }
          frame True {
            n372 = property on="DISCO 1" class="Bool (strict)"("Position"=T3 {"Left"=753, "Top"=393}) -> ()  [unwired: 2 in, 2 out]
          }
        }
        n373 = case shown="True" w2175 {
          frame False {
          }
          frame True {
            n374 = property on="DISCO 1" class="Bool (strict)"("Position"=T3 {"Left"=753, "Top"=441}) -> ()  [unwired: 2 in, 2 out]
          }
        }
        n375 = And(x=w2507, y=w2508) -> (x .and. y?=w2509:bool)
        n376 = And(x=w2488, y=w2487) -> (x .and. y?=w2486:bool)
        n377 = case shown="True" w2172 {
          frame False {
          }
          frame True {
            n378 = property on="DISCO 1" class="Bool (strict)"("Position"=T3 {"Left"=753, "Top"=489}) -> ()  [unwired: 2 in, 2 out]
          }
        }
        n379 = case shown="True" w2512 {
          frame False {
          }
          frame True {
            n380 = property on="DISCO 1" class="Bool (strict)"("Position"=T3 {"Left"=381, "Top"=489}) -> ()  [unwired: 2 in, 2 out]
          }
        }
        n381 = case shown="True" w2486 {
          frame False {
          }
          frame True {
            n382 = property on="DISCO 1" class="Bool (strict)"("Position"=T3 {"Left"=381, "Top"=393}) -> ()  [unwired: 2 in, 2 out]
          }
        }
        n383 = case shown="True" w2509 {
          frame False {
          }
          frame True {
            n384 = property on="DISCO 1" class="Bool (strict)"("Position"=T3 {"Left"=381, "Top"=441}) -> ()  [unwired: 2 in, 2 out]
          }
        }
        n385 = case shown="True" w1680 {
          frame False {
          }
          frame True {
            n386 = property on="DISCO 1" class="Bool (strict)"("Position"=T3 {"Left"=381, "Top"=297}) -> ()  [unwired: 2 in, 2 out]
          }
        }
        n387 = case shown="True" w1703 {
          frame False {
          }
          frame True {
            n388 = property on="DISCO 1" class="Bool (strict)"("Position"=T3 {"Left"=381, "Top"=345}) -> ()  [unwired: 2 in, 2 out]
          }
        }
        n389 = disable-structure shown="Disabled" {
          frame Disabled {
            n390 = property on="DISCO 4" class="Bool (strict)"() -> ("Left"=w2598:i32, "Top"=w2590:i32)  [unwired: 2 in, 2 out]
            n391 = Less Or Equal?(x=w2590, y=489) -> (x <= y?=w2597:bool)
            n392 = Less Or Equal?(x=w2598, y=900) -> (x <= y?=w2599:bool)
            n393 = Greater Or Equal?(x=w2590, y=441) -> (x >= y?=w2596:bool)
            n394 = Greater Or Equal?(x=w2598, y=700) -> (x >= y?=w2600:bool)
            n395 = And(x=w2600, y=w2599) -> (x .and. y?=w2593:bool)
            n396 = And(x=w2596, y=w2597) -> (x .and. y?=w2592:bool)
            n397 = And(x=w2593, y=w2592) -> (x .and. y?=w2591:bool)
            n398 = case shown="True" w2591 {
              frame False {
              }
              frame True {
                n399 = property on="DISCO 4" class="Bool (strict)"("Position"=T3 {"Left"=717, "Top"=489}) -> ()  [unwired: 2 in, 2 out]
              }
            }
          }
          frame Enabled {
          }
        }
        n400 = property on="DISCO 2" class="Bool (strict)"() -> ("Left"=w2243:i32, "Top"=w2251:i32)  [unwired: 2 in, 2 out]
        n401 = property on="DISCO 2" class="Bool (strict)"() -> ("Left"=w2234:i32, "Top"=w2226:i32)  [unwired: 2 in, 2 out]
        n402 = property on="DISCO 2" class="Bool (strict)"() -> ("Left"=w2285:i32, "Top"=w2278:i32)  [unwired: 2 in, 2 out]
        n403 = property on="DISCO 2" class="Bool (strict)"() -> ("Left"=w2269:i32, "Top"=w2277:i32)  [unwired: 2 in, 2 out]
        n404 = property on="DISCO 2" class="Bool (strict)"() -> ("Left"=w2260:i32, "Top"=w2252:i32)  [unwired: 2 in, 2 out]
        n405 = property on="DISCO 4" class="Bool (strict)"() -> ("Left"=w71:i32, "Top"=w79:i32)  [unwired: 2 in, 2 out]
        n406 = property on="DISCO 4" class="Bool (strict)"() -> ("Left"=w114:i32, "Top"=w106:i32)  [unwired: 2 in, 2 out]
        n407 = property on="DISCO 4" class="Bool (strict)"() -> ("Left"=w97:i32, "Top"=w105:i32)  [unwired: 2 in, 2 out]
        n408 = property on="DISCO 4" class="Bool (strict)"() -> ("Left"=w88:i32, "Top"=w80:i32)  [unwired: 2 in, 2 out]
        n409 = property on="DISCO 2" class="Bool (strict)"() -> ("Left"=w1813:i32, "Top"=w1821:i32)  [unwired: 2 in, 2 out]
        n410 = property on="DISCO 2" class="Bool (strict)"() -> ("Left"=w1791:i32, "Top"=w1783:i32)  [unwired: 2 in, 2 out]
        n411 = property on="DISCO 4" class="Bool (strict)"() -> ("Left"=w2529:i32, "Top"=w2537:i32)  [unwired: 2 in, 2 out]
        n412 = property on="DISCO 2" class="Bool (strict)"() -> ("Left"=w1774:i32, "Top"=w1782:i32)  [unwired: 2 in, 2 out]
        n413 = property on="DISCO 2" class="Bool (strict)"() -> ("Left"=w1830:i32, "Top"=w1822:i32)  [unwired: 2 in, 2 out]
        n414 = property on="DISCO 2" class="Bool (strict)"() -> ("Left"=w1800:i32, "Top"=w1808:i32)  [unwired: 2 in, 2 out]
        n415 = property on="DISCO 4" class="Bool (strict)"() -> ("Left"=w2546:i32, "Top"=w2538:i32)  [unwired: 2 in, 2 out]
        n416 = property on="DISCO 4" class="Bool (strict)"() -> ("Left"=w2555:i32, "Top"=w2563:i32)  [unwired: 2 in, 2 out]
        n417 = property on="DISCO 4" class="Bool (strict)"() -> ("Left"=w2572:i32, "Top"=w2564:i32)  [unwired: 2 in, 2 out]
        n418 = property on="DISCO 4" class="Bool (strict)"() -> ("Left"=w2581:i32, "Top"=w2589:i32)  [unwired: 2 in, 2 out]
        n419 = Greater Or Equal?(x=w97, y=700) -> (x >= y?=w95:bool)
        n420 = Less Or Equal?(x=w97, y=900) -> (x <= y?=w96:bool)
        n421 = Greater Or Equal?(x=w105, y=297) -> (x >= y?=w99:bool)
        n422 = Less Or Equal?(x=w105, y=345) -> (x <= y?=w98:bool)
        n423 = Greater Or Equal?(x=w88, y=700) -> (x >= y?=w90:bool)
        n424 = Less Or Equal?(x=w88, y=900) -> (x <= y?=w89:bool)
        n425 = Greater Or Equal?(x=w80, y=240) -> (x >= y?=w86:bool)
        n426 = Less Or Equal?(x=w80, y=297) -> (x <= y?=w87:bool)
        n427 = Greater Or Equal?(x=w71, y=700) -> (x >= y?=w69:bool)
        n428 = Less Or Equal?(x=w71, y=900) -> (x <= y?=w70:bool)
        n429 = Greater Or Equal?(x=w79, y=393) -> (x >= y?=w73:bool)
        n430 = Less Or Equal?(x=w79, y=441) -> (x <= y?=w72:bool)
        n431 = Greater Or Equal?(x=w114, y=700) -> (x >= y?=w116:bool)
        n432 = Less Or Equal?(x=w114, y=900) -> (x <= y?=w115:bool)
        n433 = Greater Or Equal?(x=w106, y=345) -> (x >= y?=w112:bool)
        n434 = Less Or Equal?(x=w106, y=393) -> (x <= y?=w113:bool)
        n435 = Less Or Equal?(x=w2226, y=297) -> (x <= y?=w2233:bool)
        n436 = Greater Or Equal?(x=w2243, y=700) -> (x >= y?=w2241:bool)
        n437 = Less Or Equal?(x=w2243, y=900) -> (x <= y?=w2242:bool)
        n438 = Greater Or Equal?(x=w2251, y=297) -> (x >= y?=w2245:bool)
        n439 = Less Or Equal?(x=w2251, y=345) -> (x <= y?=w2244:bool)
        n440 = Greater Or Equal?(x=w2234, y=700) -> (x >= y?=w2236:bool)
        n441 = Less Or Equal?(x=w2234, y=900) -> (x <= y?=w2235:bool)
        n442 = Greater Or Equal?(x=w2226, y=240) -> (x >= y?=w2232:bool)
        n443 = Greater Or Equal?(x=w2285, y=700) -> (x >= y?=w2287:bool)
        n444 = Less Or Equal?(x=w2285, y=900) -> (x <= y?=w2286:bool)
        n445 = Greater Or Equal?(x=w2278, y=441) -> (x >= y?=w2283:bool)
        n446 = Less Or Equal?(x=w2278, y=489) -> (x <= y?=w2284:bool)
        n447 = Greater Or Equal?(x=w2269, y=700) -> (x >= y?=w2267:bool)
        n448 = Less Or Equal?(x=w2269, y=900) -> (x <= y?=w2268:bool)
        n449 = Greater Or Equal?(x=w2277, y=393) -> (x >= y?=w2271:bool)
        n450 = Less Or Equal?(x=w2277, y=441) -> (x <= y?=w2270:bool)
        n451 = Greater Or Equal?(x=w2260, y=700) -> (x >= y?=w2262:bool)
        n452 = Less Or Equal?(x=w2260, y=900) -> (x <= y?=w2261:bool)
        n453 = Greater Or Equal?(x=w2252, y=345) -> (x >= y?=w2258:bool)
        n454 = Less Or Equal?(x=w2252, y=393) -> (x <= y?=w2259:bool)
        n455 = And(x=w95, y=w96) -> (x .and. y?=w102:bool)
        n456 = And(x=w99, y=w98) -> (x .and. y?=w103:bool)
        n457 = And(x=w90, y=w89) -> (x .and. y?=w83:bool)
        n458 = And(x=w86, y=w87) -> (x .and. y?=w82:bool)
        n459 = Greater Or Equal?(x=w1813, y=350) -> (x >= y?=w1811:bool)
        n460 = Less Or Equal?(x=w1813, y=500) -> (x <= y?=w1812:bool)
        n461 = Greater Or Equal?(x=w1821, y=441) -> (x >= y?=w1815:bool)
        n462 = Greater Or Equal?(x=w2572, y=350) -> (x >= y?=w2574:bool)
        n463 = Less Or Equal?(x=w2572, y=500) -> (x <= y?=w2573:bool)
        n464 = Greater Or Equal?(x=w2564, y=297) -> (x >= y?=w2570:bool)
        n465 = Less Or Equal?(x=w2564, y=345) -> (x <= y?=w2571:bool)
        n466 = And(x=w69, y=w70) -> (x .and. y?=w76:bool)
        n467 = And(x=w73, y=w72) -> (x .and. y?=w77:bool)
        n468 = And(x=w116, y=w115) -> (x .and. y?=w109:bool)
        n469 = And(x=w112, y=w113) -> (x .and. y?=w108:bool)
        n470 = Greater Or Equal?(x=w2581, y=350) -> (x >= y?=w2579:bool)
        n471 = Less Or Equal?(x=w2581, y=500) -> (x <= y?=w2580:bool)
        n472 = Greater Or Equal?(x=w2589, y=240) -> (x >= y?=w2583:bool)
        n473 = Less Or Equal?(x=w2589, y=297) -> (x <= y?=w2582:bool)
        n474 = And(x=w2241, y=w2242) -> (x .and. y?=w2248:bool)
        n475 = And(x=w2245, y=w2244) -> (x .and. y?=w2249:bool)
        n476 = And(x=w2236, y=w2235) -> (x .and. y?=w2229:bool)
        n477 = And(x=w2232, y=w2233) -> (x .and. y?=w2228:bool)
        n478 = Less Or Equal?(x=w2529, y=500) -> (x <= y?=w2528:bool)
        n479 = Greater Or Equal?(x=w2537, y=441) -> (x >= y?=w2531:bool)
        n480 = Less Or Equal?(x=w2537, y=489) -> (x <= y?=w2530:bool)
        n481 = Greater Or Equal?(x=w2546, y=350) -> (x >= y?=w2548:bool)
        n482 = Less Or Equal?(x=w2546, y=500) -> (x <= y?=w2547:bool)
        n483 = Greater Or Equal?(x=w2538, y=393) -> (x >= y?=w2544:bool)
        n484 = Less Or Equal?(x=w2538, y=441) -> (x <= y?=w2545:bool)
        n485 = Greater Or Equal?(x=w2555, y=350) -> (x >= y?=w2553:bool)
        n486 = Less Or Equal?(x=w2555, y=500) -> (x <= y?=w2554:bool)
        n487 = Greater Or Equal?(x=w2563, y=345) -> (x >= y?=w2557:bool)
        n488 = Less Or Equal?(x=w2563, y=393) -> (x <= y?=w2556:bool)
        n489 = Less Or Equal?(x=w1783, y=345) -> (x <= y?=w1790:bool)
        n490 = Greater Or Equal?(x=w2529, y=350) -> (x >= y?=w2527:bool)
        n491 = Greater Or Equal?(x=w1791, y=350) -> (x >= y?=w1793:bool)
        n492 = Less Or Equal?(x=w1791, y=500) -> (x <= y?=w1792:bool)
        n493 = Greater Or Equal?(x=w1783, y=297) -> (x >= y?=w1789:bool)
        n494 = And(x=w2287, y=w2286) -> (x .and. y?=w2280:bool)
        n495 = And(x=w2283, y=w2284) -> (x .and. y?=w2279:bool)
        n496 = And(x=w2267, y=w2268) -> (x .and. y?=w2274:bool)
        n497 = And(x=w2271, y=w2270) -> (x .and. y?=w2275:bool)
        n498 = And(x=w2262, y=w2261) -> (x .and. y?=w2255:bool)
        n499 = And(x=w2258, y=w2259) -> (x .and. y?=w2254:bool)
        n500 = Greater Or Equal?(x=w1774, y=350) -> (x >= y?=w1772:bool)
        n501 = Less Or Equal?(x=w1774, y=500) -> (x <= y?=w1773:bool)
        n502 = Greater Or Equal?(x=w1782, y=240) -> (x >= y?=w1776:bool)
        n503 = Less Or Equal?(x=w1782, y=297) -> (x <= y?=w1775:bool)
        n504 = Less Or Equal?(x=w1822, y=441) -> (x <= y?=w1829:bool)
        n505 = Less Or Equal?(x=w1808, y=393) -> (x <= y?=w1801:bool)
        n506 = Less Or Equal?(x=w1821, y=489) -> (x <= y?=w1814:bool)
        n507 = Greater Or Equal?(x=w1830, y=350) -> (x >= y?=w1832:bool)
        n508 = Less Or Equal?(x=w1830, y=500) -> (x <= y?=w1831:bool)
        n509 = Greater Or Equal?(x=w1822, y=393) -> (x >= y?=w1828:bool)
        n510 = Greater Or Equal?(x=w1800, y=350) -> (x >= y?=w1798:bool)
        n511 = Less Or Equal?(x=w1800, y=500) -> (x <= y?=w1799:bool)
        n512 = Greater Or Equal?(x=w1808, y=345) -> (x >= y?=w1802:bool)
        n513 = And(x=w102, y=w103) -> (x .and. y?=w104:bool)
        n514 = And(x=w1811, y=w1812) -> (x .and. y?=w1818:bool)
        n515 = And(x=w1815, y=w1814) -> (x .and. y?=w1819:bool)
        n516 = And(x=w83, y=w82) -> (x .and. y?=w81:bool)
        n517 = And(x=w2574, y=w2573) -> (x .and. y?=w2567:bool)
        n518 = And(x=w2570, y=w2571) -> (x .and. y?=w2566:bool)
        n519 = And(x=w2579, y=w2580) -> (x .and. y?=w2586:bool)
        n520 = And(x=w2583, y=w2582) -> (x .and. y?=w2587:bool)
        n521 = And(x=w76, y=w77) -> (x .and. y?=w78:bool)
        n522 = And(x=w109, y=w108) -> (x .and. y?=w107:bool)
        n523 = And(x=w2248, y=w2249) -> (x .and. y?=w2250:bool)
        n524 = And(x=w2527, y=w2528) -> (x .and. y?=w2534:bool)
        n525 = And(x=w2531, y=w2530) -> (x .and. y?=w2535:bool)
        n526 = And(x=w2548, y=w2547) -> (x .and. y?=w2541:bool)
        n527 = And(x=w2544, y=w2545) -> (x .and. y?=w2540:bool)
        n528 = And(x=w2553, y=w2554) -> (x .and. y?=w2560:bool)
        n529 = And(x=w2557, y=w2556) -> (x .and. y?=w2561:bool)
        n530 = And(x=w2229, y=w2228) -> (x .and. y?=w2227:bool)
        n531 = And(x=w1793, y=w1792) -> (x .and. y?=w1786:bool)
        n532 = And(x=w1789, y=w1790) -> (x .and. y?=w1785:bool)
        n533 = And(x=w1772, y=w1773) -> (x .and. y?=w1779:bool)
        n534 = And(x=w1776, y=w1775) -> (x .and. y?=w1780:bool)
        n535 = And(x=w2280, y=w2279) -> (x .and. y?=w2160:bool)
        n536 = And(x=w2274, y=w2275) -> (x .and. y?=w2276:bool)
        n537 = And(x=w2255, y=w2254) -> (x .and. y?=w2253:bool)
        n538 = And(x=w1832, y=w1831) -> (x .and. y?=w1825:bool)
        n539 = And(x=w1828, y=w1829) -> (x .and. y?=w1824:bool)
        n540 = And(x=w1798, y=w1799) -> (x .and. y?=w1805:bool)
        n541 = And(x=w1802, y=w1801) -> (x .and. y?=w1806:bool)
        n542 = And(x=w1818, y=w1819) -> (x .and. y?=w1820:bool)
        n543 = case shown="True" w81 {
          frame False {
          }
          frame True {
            n544 = property on="DISCO 4" class="Bool (strict)"("Position"=T3 {"Left"=717, "Top"=297}) -> ()  [unwired: 2 in, 2 out]
          }
        }
        n545 = And(x=w2567, y=w2566) -> (x .and. y?=w2565:bool)
        n546 = And(x=w2586, y=w2587) -> (x .and. y?=w2588:bool)
        n547 = case shown="True" w78 {
          frame False {
          }
          frame True {
            n548 = property on="DISCO 4" class="Bool (strict)"("Position"=T3 {"Left"=717, "Top"=441}) -> ()  [unwired: 2 in, 2 out]
          }
        }
        n549 = case shown="True" w104 {
          frame False {
          }
          frame True {
            n550 = property on="DISCO 4" class="Bool (strict)"("Position"=T3 {"Left"=717, "Top"=345}) -> ()  [unwired: 2 in, 2 out]
          }
        }
        n551 = And(x=w2534, y=w2535) -> (x .and. y?=w2536:bool)
        n552 = And(x=w2541, y=w2540) -> (x .and. y?=w2539:bool)
        n553 = And(x=w2560, y=w2561) -> (x .and. y?=w2562:bool)
        n554 = case shown="True" w2227 {
          frame False {
          }
          frame True {
            n555 = property on="DISCO 2" class="Bool (strict)"("Position"=T3 {"Left"=741, "Top"=297}) -> ()  [unwired: 2 in, 2 out]
          }
        }
        n556 = case shown="True" w107 {
          frame False {
          }
          frame True {
            n557 = property on="DISCO 4" class="Bool (strict)"("Position"=T3 {"Left"=717, "Top"=393}) -> ()  [unwired: 2 in, 2 out]
          }
        }
        n558 = And(x=w1786, y=w1785) -> (x .and. y?=w1784:bool)
        n559 = And(x=w1779, y=w1780) -> (x .and. y?=w1781:bool)
        n560 = case shown="True" w2250 {
          frame False {
          }
          frame True {
            n561 = property on="DISCO 2" class="Bool (strict)"("Position"=T3 {"Left"=741, "Top"=345}) -> ()  [unwired: 2 in, 2 out]
          }
        }
        n562 = case shown="True" w2253 {
          frame False {
          }
          frame True {
            n563 = property on="DISCO 2" class="Bool (strict)"("Position"=T3 {"Left"=741, "Top"=393}) -> ()  [unwired: 2 in, 2 out]
          }
        }
        n564 = case shown="True" w2276 {
          frame False {
          }
          frame True {
            n565 = property on="DISCO 2" class="Bool (strict)"("Position"=T3 {"Left"=741, "Top"=441}) -> ()  [unwired: 2 in, 2 out]
          }
        }
        n566 = And(x=w1825, y=w1824) -> (x .and. y?=w1823:bool)
        n567 = And(x=w1805, y=w1806) -> (x .and. y?=w1807:bool)
        n568 = case shown="True" w2588 {
          frame False {
          }
          frame True {
            n569 = property on="DISCO 4" class="Bool (strict)"("Position"=T3 {"Left"=345, "Top"=297}) -> ()  [unwired: 2 in, 2 out]
          }
        }
        n570 = case shown="True" w2565 {
          frame False {
          }
          frame True {
            n571 = property on="DISCO 4" class="Bool (strict)"("Position"=T3 {"Left"=345, "Top"=345}) -> ()  [unwired: 2 in, 2 out]
          }
        }
        n572 = case shown="True" w2562 {
          frame False {
          }
          frame True {
            n573 = property on="DISCO 4" class="Bool (strict)"("Position"=T3 {"Left"=345, "Top"=393}) -> ()  [unwired: 2 in, 2 out]
          }
        }
        n574 = case shown="True" w2539 {
          frame False {
          }
          frame True {
            n575 = property on="DISCO 4" class="Bool (strict)"("Position"=T3 {"Left"=345, "Top"=441}) -> ()  [unwired: 2 in, 2 out]
          }
        }
        n576 = case shown="True" w2160 {
          frame False {
          }
          frame True {
            n577 = property on="DISCO 2" class="Bool (strict)"("Position"=T3 {"Left"=741, "Top"=489}) -> ()  [unwired: 2 in, 2 out]
          }
        }
        n578 = case shown="True" w2536 {
          frame False {
          }
          frame True {
            n579 = property on="DISCO 4" class="Bool (strict)"("Position"=T3 {"Left"=345, "Top"=489}) -> ()  [unwired: 2 in, 2 out]
          }
        }
        n580 = case shown="True" w1784 {
          frame False {
          }
          frame True {
            n581 = property on="DISCO 2" class="Bool (strict)"("Position"=T3 {"Left"=369, "Top"=345}) -> ()  [unwired: 2 in, 2 out]
          }
        }
        n582 = case shown="True" w1807 {
          frame False {
          }
          frame True {
            n583 = property on="DISCO 2" class="Bool (strict)"("Position"=T3 {"Left"=369, "Top"=393}) -> ()  [unwired: 2 in, 2 out]
          }
        }
        n584 = case shown="True" w1823 {
          frame False {
          }
          frame True {
            n585 = property on="DISCO 2" class="Bool (strict)"("Position"=T3 {"Left"=369, "Top"=441}) -> ()  [unwired: 2 in, 2 out]
          }
        }
        n586 = case shown="True" w1820 {
          frame False {
          }
          frame True {
            n587 = property on="DISCO 2" class="Bool (strict)"("Position"=T3 {"Left"=369, "Top"=489}) -> ()  [unwired: 2 in, 2 out]
          }
        }
        n588 = case shown="True" w1781 {
          frame False {
          }
          frame True {
            n589 = property on="DISCO 2" class="Bool (strict)"("Position"=T3 {"Left"=369, "Top"=297}) -> ()  [unwired: 2 in, 2 out]
          }
        }
        n590 = property on="DISCO 3" class="Bool (strict)"() -> ("Left"=w1969:i32, "Top"=w1977:i32)  [unwired: 2 in, 2 out]
        n591 = property on="DISCO 3" class="Bool (strict)"() -> ("Left"=w1986:i32, "Top"=w1978:i32)  [unwired: 2 in, 2 out]
        n592 = property on="DISCO 3" class="Bool (strict)"() -> ("Left"=w1995:i32, "Top"=w2003:i32)  [unwired: 2 in, 2 out]
        n593 = property on="DISCO 3" class="Bool (strict)"() -> ("Left"=w2012:i32, "Top"=w2004:i32)  [unwired: 2 in, 2 out]
        n594 = property on="DISCO 3" class="Bool (strict)"() -> ("Left"=w2021:i32, "Top"=w2029:i32)  [unwired: 2 in, 2 out]
        n595 = property on="DISCO 5" class="Bool (strict)"() -> ("Left"=w2155:i32, "Top"=w2147:i32)  [unwired: 2 in, 2 out]
        n596 = property on="DISCO 5" class="Bool (strict)"() -> ("Left"=w2138:i32, "Top"=w2146:i32)  [unwired: 2 in, 2 out]
        n597 = property on="DISCO 5" class="Bool (strict)"() -> ("Left"=w2129:i32, "Top"=w2121:i32)  [unwired: 2 in, 2 out]
        n598 = property on="DISCO 5" class="Bool (strict)"() -> ("Left"=w2112:i32, "Top"=w2120:i32)  [unwired: 2 in, 2 out]
        n599 = property on="DISCO 5" class="Bool (strict)"() -> ("Left"=w2103:i32, "Top"=w2095:i32)  [unwired: 2 in, 2 out]
        n600 = property on="DISCO 1" class="Bool (strict)"() -> ("Left"=w1839:i32, "Top"=w1847:i32)  [unwired: 2 in, 2 out]
        n601 = property on="DISCO 1" class="Bool (strict)"() -> ("Left"=w1882:i32, "Top"=w1874:i32)  [unwired: 2 in, 2 out]
        n602 = property on="DISCO 1" class="Bool (strict)"() -> ("Left"=w1891:i32, "Top"=w1899:i32)  [unwired: 2 in, 2 out]
        n603 = property on="DISCO 1" class="Bool (strict)"() -> ("Left"=w1856:i32, "Top"=w1848:i32)  [unwired: 2 in, 2 out]
        n604 = property on="DISCO 1" class="Bool (strict)"() -> ("Left"=w1865:i32, "Top"=w1873:i32)  [unwired: 2 in, 2 out]
        n605 = Greater Or Equal?(x=w2112, y=0) -> (x >= y?=w2110:bool)
        n606 = Less Or Equal?(x=w2112, y=160) -> (x <= y?=w2111:bool)
        n607 = Greater Or Equal?(x=w2120, y=297) -> (x >= y?=w2114:bool)
        n608 = Less Or Equal?(x=w2120, y=345) -> (x <= y?=w2113:bool)
        n609 = Greater Or Equal?(x=w2103, y=0) -> (x >= y?=w2105:bool)
        n610 = Less Or Equal?(x=w2103, y=1608) -> (x <= y?=w2104:bool)
        n611 = Greater Or Equal?(x=w2095, y=240) -> (x >= y?=w2101:bool)
        n612 = Less Or Equal?(x=w2095, y=297) -> (x <= y?=w2102:bool)
        n613 = Greater Or Equal?(x=w2012, y=0) -> (x >= y?=w2014:bool)
        n614 = Less Or Equal?(x=w2012, y=160) -> (x <= y?=w2013:bool)
        n615 = Greater Or Equal?(x=w2004, y=297) -> (x >= y?=w2010:bool)
        n616 = Less Or Equal?(x=w2004, y=345) -> (x <= y?=w2011:bool)
        n617 = Greater Or Equal?(x=w2021, y=0) -> (x >= y?=w2019:bool)
        n618 = Less Or Equal?(x=w2021, y=160) -> (x <= y?=w2020:bool)
        n619 = Greater Or Equal?(x=w2029, y=240) -> (x >= y?=w2023:bool)
        n620 = Less Or Equal?(x=w2029, y=297) -> (x <= y?=w2022:bool)
        n621 = Less Or Equal?(x=w2155, y=160) -> (x <= y?=w2156:bool)
        n622 = Greater Or Equal?(x=w2147, y=441) -> (x >= y?=w2153:bool)
        n623 = Less Or Equal?(x=w2147, y=489) -> (x <= y?=w2154:bool)
        n624 = Greater Or Equal?(x=w2138, y=0) -> (x >= y?=w2136:bool)
        n625 = Less Or Equal?(x=w2138, y=160) -> (x <= y?=w2137:bool)
        n626 = Greater Or Equal?(x=w2146, y=393) -> (x >= y?=w2140:bool)
        n627 = Less Or Equal?(x=w2146, y=441) -> (x <= y?=w2139:bool)
        n628 = Greater Or Equal?(x=w2129, y=0) -> (x >= y?=w2131:bool)
        n629 = Less Or Equal?(x=w2129, y=160) -> (x <= y?=w2130:bool)
        n630 = Greater Or Equal?(x=w2121, y=345) -> (x >= y?=w2127:bool)
        n631 = Less Or Equal?(x=w2121, y=393) -> (x <= y?=w2128:bool)
        n632 = Less Or Equal?(x=w1969, y=160) -> (x <= y?=w1968:bool)
        n633 = Greater Or Equal?(x=w1977, y=441) -> (x >= y?=w1971:bool)
        n634 = Less Or Equal?(x=w1977, y=489) -> (x <= y?=w1970:bool)
        n635 = Greater Or Equal?(x=w1986, y=0) -> (x >= y?=w1988:bool)
        n636 = Less Or Equal?(x=w1986, y=160) -> (x <= y?=w1987:bool)
        n637 = Greater Or Equal?(x=w1978, y=393) -> (x >= y?=w1984:bool)
        n638 = Less Or Equal?(x=w1978, y=441) -> (x <= y?=w1985:bool)
        n639 = Greater Or Equal?(x=w1995, y=0) -> (x >= y?=w1993:bool)
        n640 = Less Or Equal?(x=w1995, y=160) -> (x <= y?=w1994:bool)
        n641 = Greater Or Equal?(x=w2003, y=345) -> (x >= y?=w1997:bool)
        n642 = Less Or Equal?(x=w2003, y=393) -> (x <= y?=w1996:bool)
        n643 = Greater Or Equal?(x=w2155, y=0) -> (x >= y?=w2157:bool)
        n644 = Greater Or Equal?(x=w1969, y=0) -> (x >= y?=w1967:bool)
        n645 = And(x=w2110, y=w2111) -> (x .and. y?=w2117:bool)
        n646 = And(x=w2114, y=w2113) -> (x .and. y?=w2118:bool)
        n647 = And(x=w2105, y=w2104) -> (x .and. y?=w2098:bool)
        n648 = And(x=w2101, y=w2102) -> (x .and. y?=w2097:bool)
        n649 = And(x=w2014, y=w2013) -> (x .and. y?=w2007:bool)
        n650 = And(x=w2010, y=w2011) -> (x .and. y?=w2006:bool)
        n651 = And(x=w2019, y=w2020) -> (x .and. y?=w2026:bool)
        n652 = And(x=w2023, y=w2022) -> (x .and. y?=w2027:bool)
        n653 = And(x=w2157, y=w2156) -> (x .and. y?=w2150:bool)
        n654 = And(x=w2153, y=w2154) -> (x .and. y?=w2149:bool)
        n655 = And(x=w2136, y=w2137) -> (x .and. y?=w2143:bool)
        n656 = And(x=w2140, y=w2139) -> (x .and. y?=w2144:bool)
        n657 = And(x=w2131, y=w2130) -> (x .and. y?=w2124:bool)
        n658 = And(x=w2127, y=w2128) -> (x .and. y?=w2123:bool)
        n659 = And(x=w1967, y=w1968) -> (x .and. y?=w1974:bool)
        n660 = And(x=w1971, y=w1970) -> (x .and. y?=w1975:bool)
        n661 = And(x=w1988, y=w1987) -> (x .and. y?=w1981:bool)
        n662 = And(x=w1984, y=w1985) -> (x .and. y?=w1980:bool)
        n663 = And(x=w1993, y=w1994) -> (x .and. y?=w2000:bool)
        n664 = And(x=w1997, y=w1996) -> (x .and. y?=w2001:bool)
        n665 = Greater Or Equal?(x=w1839, y=0) -> (x >= y?=w1837:bool)
        n666 = Less Or Equal?(x=w1839, y=160) -> (x <= y?=w1838:bool)
        n667 = Greater Or Equal?(x=w1847, y=441) -> (x >= y?=w1841:bool)
        n668 = Greater Or Equal?(x=w1882, y=0) -> (x >= y?=w1884:bool)
        n669 = Less Or Equal?(x=w1882, y=160) -> (x <= y?=w1883:bool)
        n670 = Greater Or Equal?(x=w1874, y=297) -> (x >= y?=w1880:bool)
        n671 = Less Or Equal?(x=w1874, y=345) -> (x <= y?=w1881:bool)
        n672 = And(x=w2117, y=w2118) -> (x .and. y?=w2119:bool)
        n673 = Greater Or Equal?(x=w1891, y=0) -> (x >= y?=w1889:bool)
        n674 = Less Or Equal?(x=w1891, y=160) -> (x <= y?=w1890:bool)
        n675 = Greater Or Equal?(x=w1899, y=240) -> (x >= y?=w1893:bool)
        n676 = Less Or Equal?(x=w1899, y=297) -> (x <= y?=w1892:bool)
        n677 = And(x=w2098, y=w2097) -> (x .and. y?=w2096:bool)
        n678 = And(x=w2007, y=w2006) -> (x .and. y?=w2005:bool)
        n679 = And(x=w2026, y=w2027) -> (x .and. y?=w2028:bool)
        n680 = Less Or Equal?(x=w1847, y=489) -> (x <= y?=w1840:bool)
        n681 = Greater Or Equal?(x=w1856, y=0) -> (x >= y?=w1858:bool)
        n682 = Less Or Equal?(x=w1856, y=160) -> (x <= y?=w1857:bool)
        n683 = Greater Or Equal?(x=w1848, y=393) -> (x >= y?=w1854:bool)
        n684 = Less Or Equal?(x=w1848, y=441) -> (x <= y?=w1855:bool)
        n685 = Greater Or Equal?(x=w1865, y=0) -> (x >= y?=w1863:bool)
        n686 = Less Or Equal?(x=w1865, y=160) -> (x <= y?=w1864:bool)
        n687 = Greater Or Equal?(x=w1873, y=345) -> (x >= y?=w1867:bool)
        n688 = Less Or Equal?(x=w1873, y=393) -> (x <= y?=w1866:bool)
        n689 = And(x=w2150, y=w2149) -> (x .and. y?=w2148:bool)
        n690 = And(x=w2143, y=w2144) -> (x .and. y?=w2145:bool)
        n691 = And(x=w2124, y=w2123) -> (x .and. y?=w2122:bool)
        n692 = And(x=w1974, y=w1975) -> (x .and. y?=w1976:bool)
        n693 = And(x=w1981, y=w1980) -> (x .and. y?=w1979:bool)
        n694 = And(x=w2000, y=w2001) -> (x .and. y?=w2002:bool)
        n695 = And(x=w1837, y=w1838) -> (x .and. y?=w1844:bool)
        n696 = And(x=w1841, y=w1840) -> (x .and. y?=w1845:bool)
        n697 = And(x=w1884, y=w1883) -> (x .and. y?=w1877:bool)
        n698 = And(x=w1880, y=w1881) -> (x .and. y?=w1876:bool)
        n699 = And(x=w1889, y=w1890) -> (x .and. y?=w1896:bool)
        n700 = And(x=w1893, y=w1892) -> (x .and. y?=w1897:bool)
        n701 = case shown="True" w2096 {
          frame False {
          }
          frame True {
            n702 = property on="DISCO 5" class="Bool (strict)"("Position"=T3 {"Left"=-32, "Top"=297}) -> ()  [unwired: 2 in, 2 out]
          }
        }
        n703 = And(x=w1858, y=w1857) -> (x .and. y?=w1851:bool)
        n704 = And(x=w1854, y=w1855) -> (x .and. y?=w1850:bool)
        n705 = And(x=w1863, y=w1864) -> (x .and. y?=w1870:bool)
        n706 = And(x=w1867, y=w1866) -> (x .and. y?=w1871:bool)
        n707 = case shown="True" w2028 {
          frame False {
          }
          frame True {
            n708 = property on="DISCO 3" class="Bool (strict)"("Position"=T3 {"Left"=-13, "Top"=297}) -> ()  [unwired: 2 in, 2 out]
          }
        }
        n709 = case shown="True" w2119 {
          frame False {
          }
          frame True {
            n710 = property on="DISCO 5" class="Bool (strict)"("Position"=T3 {"Left"=-32, "Top"=345}) -> ()  [unwired: 2 in, 2 out]
          }
        }
        n711 = case shown="True" w2122 {
          frame False {
          }
          frame True {
            n712 = property on="DISCO 5" class="Bool (strict)"("Position"=T3 {"Left"=-32, "Top"=393}) -> ()  [unwired: 2 in, 2 out]
          }
        }
        n713 = case shown="True" w2145 {
          frame False {
          }
          frame True {
            n714 = property on="DISCO 5" class="Bool (strict)"("Position"=T3 {"Left"=-32, "Top"=441}) -> ()  [unwired: 2 in, 2 out]
          }
        }
        n715 = case shown="True" w2005 {
          frame False {
          }
          frame True {
            n716 = property on="DISCO 3" class="Bool (strict)"("Position"=T3 {"Left"=-13, "Top"=345}) -> ()  [unwired: 2 in, 2 out]
          }
        }
        n717 = case shown="True" w2002 {
          frame False {
          }
          frame True {
            n718 = property on="DISCO 3" class="Bool (strict)"("Position"=T3 {"Left"=-13, "Top"=393}) -> ()  [unwired: 2 in, 2 out]
          }
        }
        n719 = case shown="True" w1979 {
          frame False {
          }
          frame True {
            n720 = property on="DISCO 3" class="Bool (strict)"("Position"=T3 {"Left"=-13, "Top"=441}) -> ()  [unwired: 2 in, 2 out]
          }
        }
        n721 = And(x=w1844, y=w1845) -> (x .and. y?=w1846:bool)
        n722 = case shown="True" w2148 {
          frame False {
          }
          frame True {
            n723 = property on="DISCO 5" class="Bool (strict)"("Position"=T3 {"Left"=-32, "Top"=489}) -> ()  [unwired: 2 in, 2 out]
          }
        }
        n724 = case shown="True" w1976 {
          frame False {
          }
          frame True {
            n725 = property on="DISCO 3" class="Bool (strict)"("Position"=T3 {"Left"=-13, "Top"=489}) -> ()  [unwired: 2 in, 2 out]
          }
        }
        n726 = And(x=w1877, y=w1876) -> (x .and. y?=w1875:bool)
        n727 = And(x=w1896, y=w1897) -> (x .and. y?=w1898:bool)
        n728 = And(x=w1851, y=w1850) -> (x .and. y?=w1849:bool)
        n729 = And(x=w1870, y=w1871) -> (x .and. y?=w1872:bool)
        n730 = case shown="True" w1846 {
          frame False {
          }
          frame True {
            n731 = property on="DISCO 1" class="Bool (strict)"("Position"=T3 {"Left"=7, "Top"=489}) -> ()  [unwired: 2 in, 2 out]
          }
        }
        n732 = case shown="True" w1898 {
          frame False {
          }
          frame True {
            n733 = property on="DISCO 1" class="Bool (strict)"("Position"=T3 {"Left"=7, "Top"=297}) -> ()  [unwired: 2 in, 2 out]
          }
        }
        n734 = case shown="True" w1875 {
          frame False {
          }
          frame True {
            n735 = property on="DISCO 1" class="Bool (strict)"("Position"=T3 {"Left"=7, "Top"=345}) -> ()  [unwired: 2 in, 2 out]
          }
        }
        n736 = case shown="True" w1872 {
          frame False {
          }
          frame True {
            n737 = property on="DISCO 1" class="Bool (strict)"("Position"=T3 {"Left"=7, "Top"=393}) -> ()  [unwired: 2 in, 2 out]
          }
        }
        n738 = case shown="True" w1849 {
          frame False {
          }
          frame True {
            n739 = property on="DISCO 1" class="Bool (strict)"("Position"=T3 {"Left"=7, "Top"=441}) -> ()  [unwired: 2 in, 2 out]
          }
        }
        n740 = property on="DISCO 2" class="Bool (strict)"() -> ("Left"=w1960:i32, "Top"=w1952:i32)  [unwired: 2 in, 2 out]
        n741 = property on="DISCO 2" class="Bool (strict)"() -> ("Left"=w1917:i32, "Top"=w1925:i32)  [unwired: 2 in, 2 out]
        n742 = property on="DISCO 4" class="Bool (strict)"() -> ("Left"=w2090:i32, "Top"=w2082:i32)  [unwired: 2 in, 2 out]
        n743 = property on="DISCO 2" class="Bool (strict)"() -> ("Left"=w1908:i32, "Top"=w1900:i32)  [unwired: 2 in, 2 out]
        n744 = property on="DISCO 2" class="Bool (strict)"() -> ("Left"=w1943:i32, "Top"=w1951:i32)  [unwired: 2 in, 2 out]
        n745 = property on="DISCO 2" class="Bool (strict)"() -> ("Left"=w1934:i32, "Top"=w1926:i32)  [unwired: 2 in, 2 out]
        n746 = property on="DISCO 4" class="Bool (strict)"() -> ("Left"=w2073:i32, "Top"=w2081:i32)  [unwired: 2 in, 2 out]
        n747 = property on="DISCO 4" class="Bool (strict)"() -> ("Left"=w2064:i32, "Top"=w2056:i32)  [unwired: 2 in, 2 out]
        n748 = property on="DISCO 4" class="Bool (strict)"() -> ("Left"=w2047:i32, "Top"=w2055:i32)  [unwired: 2 in, 2 out]
        n749 = property on="DISCO 4" class="Bool (strict)"() -> ("Left"=w2038:i32, "Top"=w2030:i32)  [unwired: 2 in, 2 out]
        n750 = Greater Or Equal?(x=w1960, y=0) -> (x >= y?=w1962:bool)
        n751 = Less Or Equal?(x=w1960, y=160) -> (x <= y?=w1961:bool)
        n752 = Greater Or Equal?(x=w1952, y=441) -> (x >= y?=w1958:bool)
        n753 = Greater Or Equal?(x=w2047, y=0) -> (x >= y?=w2045:bool)
        n754 = Less Or Equal?(x=w2047, y=160) -> (x <= y?=w2046:bool)
        n755 = Greater Or Equal?(x=w2055, y=297) -> (x >= y?=w2049:bool)
        n756 = Less Or Equal?(x=w2055, y=345) -> (x <= y?=w2048:bool)
        n757 = Greater Or Equal?(x=w2038, y=0) -> (x >= y?=w2040:bool)
        n758 = Less Or Equal?(x=w2038, y=160) -> (x <= y?=w2039:bool)
        n759 = Greater Or Equal?(x=w2030, y=240) -> (x >= y?=w2036:bool)
        n760 = Less Or Equal?(x=w2030, y=297) -> (x <= y?=w2037:bool)
        n761 = Less Or Equal?(x=w2090, y=160) -> (x <= y?=w2091:bool)
        n762 = Greater Or Equal?(x=w2082, y=441) -> (x >= y?=w2088:bool)
        n763 = Less Or Equal?(x=w2082, y=489) -> (x <= y?=w2089:bool)
        n764 = Greater Or Equal?(x=w2073, y=0) -> (x >= y?=w2071:bool)
        n765 = Less Or Equal?(x=w2073, y=160) -> (x <= y?=w2072:bool)
        n766 = Greater Or Equal?(x=w2081, y=393) -> (x >= y?=w2075:bool)
        n767 = Less Or Equal?(x=w2081, y=441) -> (x <= y?=w2074:bool)
        n768 = Greater Or Equal?(x=w2064, y=0) -> (x >= y?=w2066:bool)
        n769 = Less Or Equal?(x=w2064, y=160) -> (x <= y?=w2065:bool)
        n770 = Greater Or Equal?(x=w2056, y=345) -> (x >= y?=w2062:bool)
        n771 = Less Or Equal?(x=w2056, y=393) -> (x <= y?=w2063:bool)
        n772 = Greater Or Equal?(x=w2090, y=0) -> (x >= y?=w2092:bool)
        n773 = Greater Or Equal?(x=w1917, y=0) -> (x >= y?=w1915:bool)
        n774 = Less Or Equal?(x=w1917, y=160) -> (x <= y?=w1916:bool)
        n775 = Greater Or Equal?(x=w1925, y=297) -> (x >= y?=w1919:bool)
        n776 = Less Or Equal?(x=w1925, y=345) -> (x <= y?=w1918:bool)
        n777 = Greater Or Equal?(x=w1908, y=0) -> (x >= y?=w1910:bool)
        n778 = Less Or Equal?(x=w1908, y=160) -> (x <= y?=w1909:bool)
        n779 = Greater Or Equal?(x=w1900, y=240) -> (x >= y?=w1906:bool)
        n780 = Less Or Equal?(x=w1900, y=297) -> (x <= y?=w1907:bool)
        n781 = Less Or Equal?(x=w1952, y=489) -> (x <= y?=w1959:bool)
        n782 = Greater Or Equal?(x=w1943, y=0) -> (x >= y?=w1941:bool)
        n783 = Less Or Equal?(x=w1943, y=160) -> (x <= y?=w1942:bool)
        n784 = Greater Or Equal?(x=w1951, y=393) -> (x >= y?=w1945:bool)
        n785 = Less Or Equal?(x=w1951, y=441) -> (x <= y?=w1944:bool)
        n786 = Greater Or Equal?(x=w1934, y=0) -> (x >= y?=w1936:bool)
        n787 = Less Or Equal?(x=w1934, y=160) -> (x <= y?=w1935:bool)
        n788 = Greater Or Equal?(x=w1926, y=345) -> (x >= y?=w1932:bool)
        n789 = Less Or Equal?(x=w1926, y=393) -> (x <= y?=w1933:bool)
        n790 = And(x=w1962, y=w1961) -> (x .and. y?=w1955:bool)
        n791 = And(x=w1958, y=w1959) -> (x .and. y?=w1954:bool)
        n792 = And(x=w2045, y=w2046) -> (x .and. y?=w2052:bool)
        n793 = And(x=w2049, y=w2048) -> (x .and. y?=w2053:bool)
        n794 = And(x=w2040, y=w2039) -> (x .and. y?=w2033:bool)
        n795 = And(x=w2036, y=w2037) -> (x .and. y?=w2032:bool)
        n796 = And(x=w2092, y=w2091) -> (x .and. y?=w2085:bool)
        n797 = And(x=w2088, y=w2089) -> (x .and. y?=w2084:bool)
        n798 = And(x=w2071, y=w2072) -> (x .and. y?=w2078:bool)
        n799 = And(x=w2075, y=w2074) -> (x .and. y?=w2079:bool)
        n800 = And(x=w2066, y=w2065) -> (x .and. y?=w2059:bool)
        n801 = And(x=w2062, y=w2063) -> (x .and. y?=w2058:bool)
        n802 = And(x=w1915, y=w1916) -> (x .and. y?=w1922:bool)
        n803 = And(x=w1919, y=w1918) -> (x .and. y?=w1923:bool)
        n804 = And(x=w1910, y=w1909) -> (x .and. y?=w1903:bool)
        n805 = And(x=w1906, y=w1907) -> (x .and. y?=w1902:bool)
        n806 = And(x=w1941, y=w1942) -> (x .and. y?=w1948:bool)
        n807 = And(x=w1945, y=w1944) -> (x .and. y?=w1949:bool)
        n808 = And(x=w1936, y=w1935) -> (x .and. y?=w1929:bool)
        n809 = And(x=w1932, y=w1933) -> (x .and. y?=w1928:bool)
        n810 = And(x=w1955, y=w1954) -> (x .and. y?=w1953:bool)
        n811 = And(x=w2052, y=w2053) -> (x .and. y?=w2054:bool)
        n812 = And(x=w2033, y=w2032) -> (x .and. y?=w2031:bool)
        n813 = And(x=w2085, y=w2084) -> (x .and. y?=w2083:bool)
        n814 = And(x=w2078, y=w2079) -> (x .and. y?=w2080:bool)
        n815 = And(x=w2059, y=w2058) -> (x .and. y?=w2057:bool)
        n816 = And(x=w1922, y=w1923) -> (x .and. y?=w1924:bool)
        n817 = And(x=w1903, y=w1902) -> (x .and. y?=w1901:bool)
        n818 = And(x=w1948, y=w1949) -> (x .and. y?=w1950:bool)
        n819 = And(x=w1929, y=w1928) -> (x .and. y?=w1927:bool)
        n820 = case shown="True" w1953 {
          frame False {
          }
          frame True {
            n821 = property on="DISCO 2" class="Bool (strict)"("Position"=T3 {"Left"=-2, "Top"=489}) -> ()  [unwired: 2 in, 2 out]
          }
        }
        n822 = case shown="True" w2031 {
          frame False {
          }
          frame True {
            n823 = property on="DISCO 4" class="Bool (strict)"("Position"=T3 {"Left"=-22, "Top"=297}) -> ()  [unwired: 2 in, 2 out]
          }
        }
        n824 = case shown="True" w2054 {
          frame False {
          }
          frame True {
            n825 = property on="DISCO 4" class="Bool (strict)"("Position"=T3 {"Left"=-22, "Top"=345}) -> ()  [unwired: 2 in, 2 out]
          }
        }
        n826 = case shown="True" w2057 {
          frame False {
          }
          frame True {
            n827 = property on="DISCO 4" class="Bool (strict)"("Position"=T3 {"Left"=-22, "Top"=393}) -> ()  [unwired: 2 in, 2 out]
          }
        }
        n828 = case shown="True" w2080 {
          frame False {
          }
          frame True {
            n829 = property on="DISCO 4" class="Bool (strict)"("Position"=T3 {"Left"=-22, "Top"=441}) -> ()  [unwired: 2 in, 2 out]
          }
        }
        n830 = case shown="True" w1901 {
          frame False {
          }
          frame True {
            n831 = property on="DISCO 2" class="Bool (strict)"("Position"=T3 {"Left"=-2, "Top"=297}) -> ()  [unwired: 2 in, 2 out]
          }
        }
        n832 = case shown="True" w2083 {
          frame False {
          }
          frame True {
            n833 = property on="DISCO 4" class="Bool (strict)"("Position"=T3 {"Left"=-22, "Top"=489}) -> ()  [unwired: 2 in, 2 out]
          }
        }
        n834 = case shown="True" w1924 {
          frame False {
          }
          frame True {
            n835 = property on="DISCO 2" class="Bool (strict)"("Position"=T3 {"Left"=-2, "Top"=345}) -> ()  [unwired: 2 in, 2 out]
          }
        }
        n836 = case shown="True" w1927 {
          frame False {
          }
          frame True {
            n837 = property on="DISCO 2" class="Bool (strict)"("Position"=T3 {"Left"=-2, "Top"=393}) -> ()  [unwired: 2 in, 2 out]
          }
        }
        n838 = case shown="True" w1950 {
          frame False {
          }
          frame True {
            n839 = property on="DISCO 2" class="Bool (strict)"("Position"=T3 {"Left"=-2, "Top"=441}) -> ()  [unwired: 2 in, 2 out]
          }
        }
        n840 = property on="DISCO 2" class="Bool (strict)"() -> ("Left"=w912:i32, "Top"=w906:i32)  [unwired: 2 in, 2 out]
        n841 = property on="DISCO 3" class="Bool (strict)"() -> ("Left"=w934:i32, "Top"=w940:i32)  [unwired: 2 in, 2 out]
        n842 = property on="DISCO 1" class="Bool (strict)"() -> ("Left"=w923:i32, "Top"=w929:i32)  [unwired: 2 in, 2 out]
        n843 = property on="DISCO 4" class="Bool (strict)"() -> ("Left"=w952:i32, "Top"=w946:i32)  [unwired: 2 in, 2 out]
        n844 = property on="DISCO 5" class="Bool (strict)"() -> ("Left"=w963:i32, "Top"=w969:i32)  [unwired: 2 in, 2 out]
        n845 = property on="DISCO 2" class="Bool (strict)"() -> ("Left"=w896:i32, "Top"=w902:i32)  [unwired: 2 in, 2 out]
        n846 = property on="DISCO 3" class="Bool (strict)"() -> ("Left"=w873:i32, "Top"=w867:i32)  [unwired: 2 in, 2 out]
        n847 = property on="DISCO 1" class="Bool (strict)"() -> ("Left"=w885:i32, "Top"=w879:i32)  [unwired: 2 in, 2 out]
        n848 = property on="DISCO 4" class="Bool (strict)"() -> ("Left"=w855:i32, "Top"=w861:i32)  [unwired: 2 in, 2 out]
        n849 = property on="DISCO 5" class="Bool (strict)"() -> ("Left"=w844:i32, "Top"=w838:i32)  [unwired: 2 in, 2 out]
        n850 = Greater Or Equal?(x=w912, y=0) -> (x >= y?=w914:bool)
        n851 = Less Or Equal?(x=w912, y=160) -> (x <= y?=w913:bool)
        n852 = Greater Or Equal?(x=w906, y=393) -> (x >= y?=w910:bool)
        n853 = Less Or Equal?(x=w906, y=441) -> (x <= y?=w911:bool)
        n854 = Less Or Equal?(x=w934, y=160) -> (x <= y?=w933:bool)
        n855 = Greater Or Equal?(x=w940, y=393) -> (x >= y?=w936:bool)
        n856 = Less Or Equal?(x=w940, y=441) -> (x <= y?=w935:bool)
        n857 = Greater Or Equal?(x=w923, y=0) -> (x >= y?=w921:bool)
        n858 = Less Or Equal?(x=w923, y=160) -> (x <= y?=w922:bool)
        n859 = Greater Or Equal?(x=w929, y=441) -> (x >= y?=w925:bool)
        n860 = Less Or Equal?(x=w929, y=489) -> (x <= y?=w924:bool)
        n861 = Greater Or Equal?(x=w952, y=0) -> (x >= y?=w954:bool)
        n862 = Less Or Equal?(x=w952, y=160) -> (x <= y?=w953:bool)
        n863 = Greater Or Equal?(x=w946, y=393) -> (x >= y?=w950:bool)
        n864 = Less Or Equal?(x=w946, y=441) -> (x <= y?=w951:bool)
        n865 = Greater Or Equal?(x=w963, y=0) -> (x >= y?=w961:bool)
        n866 = Less Or Equal?(x=w963, y=160) -> (x <= y?=w962:bool)
        n867 = Greater Or Equal?(x=w969, y=393) -> (x >= y?=w965:bool)
        n868 = Less Or Equal?(x=w969, y=441) -> (x <= y?=w964:bool)
        n869 = Greater Or Equal?(x=w934, y=0) -> (x >= y?=w932:bool)
        n870 = Greater Or Equal?(x=w896, y=350) -> (x >= y?=w894:bool)
        n871 = Less Or Equal?(x=w896, y=500) -> (x <= y?=w895:bool)
        n872 = Greater Or Equal?(x=w902, y=393) -> (x >= y?=w898:bool)
        n873 = Less Or Equal?(x=w902, y=441) -> (x <= y?=w897:bool)
        n874 = Greater Or Equal?(x=w873, y=350) -> (x >= y?=w875:bool)
        n875 = Less Or Equal?(x=w873, y=500) -> (x <= y?=w874:bool)
        n876 = Greater Or Equal?(x=w867, y=393) -> (x >= y?=w871:bool)
        n877 = Less Or Equal?(x=w867, y=441) -> (x <= y?=w872:bool)
        n878 = Greater Or Equal?(x=w885, y=350) -> (x >= y?=w887:bool)
        n879 = Less Or Equal?(x=w885, y=500) -> (x <= y?=w886:bool)
        n880 = Greater Or Equal?(x=w879, y=441) -> (x >= y?=w883:bool)
        n881 = Less Or Equal?(x=w879, y=489) -> (x <= y?=w884:bool)
        n882 = Greater Or Equal?(x=w855, y=350) -> (x >= y?=w853:bool)
        n883 = Less Or Equal?(x=w855, y=500) -> (x <= y?=w854:bool)
        n884 = Greater Or Equal?(x=w861, y=393) -> (x >= y?=w857:bool)
        n885 = Less Or Equal?(x=w861, y=441) -> (x <= y?=w856:bool)
        n886 = Greater Or Equal?(x=w844, y=350) -> (x >= y?=w846:bool)
        n887 = Less Or Equal?(x=w844, y=500) -> (x <= y?=w845:bool)
        n888 = Greater Or Equal?(x=w838, y=393) -> (x >= y?=w842:bool)
        n889 = Less Or Equal?(x=w838, y=441) -> (x <= y?=w843:bool)
        n890 = And(x=w914, y=w913) -> (x .and. y?=w908:bool)
        n891 = And(x=w910, y=w911) -> (x .and. y?=w907:bool)
        n892 = And(x=w932, y=w933) -> (x .and. y?=w938:bool)
        n893 = And(x=w936, y=w935) -> (x .and. y?=w939:bool)
        n894 = And(x=w921, y=w922) -> (x .and. y?=w927:bool)
        n895 = And(x=w925, y=w924) -> (x .and. y?=w928:bool)
        n896 = And(x=w954, y=w953) -> (x .and. y?=w948:bool)
        n897 = And(x=w950, y=w951) -> (x .and. y?=w947:bool)
        n898 = And(x=w961, y=w962) -> (x .and. y?=w967:bool)
        n899 = And(x=w965, y=w964) -> (x .and. y?=w968:bool)
        n900 = And(x=w894, y=w895) -> (x .and. y?=w900:bool)
        n901 = And(x=w898, y=w897) -> (x .and. y?=w901:bool)
        n902 = And(x=w875, y=w874) -> (x .and. y?=w869:bool)
        n903 = And(x=w871, y=w872) -> (x .and. y?=w868:bool)
        n904 = And(x=w887, y=w886) -> (x .and. y?=w881:bool)
        n905 = And(x=w883, y=w884) -> (x .and. y?=w880:bool)
        n906 = And(x=w853, y=w854) -> (x .and. y?=w859:bool)
        n907 = And(x=w857, y=w856) -> (x .and. y?=w860:bool)
        n908 = And(x=w846, y=w845) -> (x .and. y?=w840:bool)
        n909 = And(x=w842, y=w843) -> (x .and. y?=w839:bool)
        n910 = And(x=w908, y=w907) -> (x .and. y?=w941:bool)
        n911 = And(x=w938, y=w939) -> (x .and. y?=w942:bool)
        n912 = And(x=w927, y=w928) -> (x .and. y?=w970:bool)
        n913 = And(x=w948, y=w947) -> (x .and. y?=w971:bool)
        n914 = And(x=w967, y=w968) -> (x .and. y?=w972:bool)
        n915 = And(x=w900, y=w901) -> (x .and. y?=w866:bool)
        n916 = And(x=w869, y=w868) -> (x .and. y?=w865:bool)
        n917 = And(x=w881, y=w880) -> (x .and. y?=w837:bool)
        n918 = And(x=w859, y=w860) -> (x .and. y?=w836:bool)
        n919 = And(x=w840, y=w839) -> (x .and. y?=w835:bool)
        n920 = And(x=w970, y=w941) -> (x .and. y?=w943:bool)
        n921 = And(x=w970, y=w942) -> (x .and. y?=w944:bool)
        n922 = And(x=w970, y=w971) -> (x .and. y?=w973:bool)
        n923 = And(x=w970, y=w972) -> (x .and. y?=w974:bool)
        n924 = And(x=w837, y=w866) -> (x .and. y?=w864:bool)
        n925 = And(x=w837, y=w865) -> (x .and. y?=w863:bool)
        n926 = And(x=w837, y=w836) -> (x .and. y?=w834:bool)
        n927 = And(x=w837, y=w835) -> (x .and. y?=w833:bool)
        n928 = Compound Arithmetic op=OR(w943, w944, w973, w974) -> (w945:bool)
        n929 = Compound Arithmetic op=OR(w864, w863, w834, w833) -> (w862:bool)
        n930 = case shown="False" w945 {
          frame False {
          }
          frame True {
            n931 = local write "String"("MOVIMIENTO INCORRECTO" ("String")) -> ()
          }
        }
        n932 = case shown="False" w862 {
          frame False {
          }
          frame True {
            n933 = local write "String"("MOVIMIENTO INCORRECTO" ("String")) -> ()
          }
        }
        n934 = property on="DISCO 2" class="Bool (strict)"() -> ("Left"=w1013:i32, "Top"=w1007:i32)  [unwired: 2 in, 2 out]
        n935 = property on="DISCO 4" class="Bool (strict)"() -> ("Left"=w1001:i32, "Top"=w995:i32)  [unwired: 2 in, 2 out]
        n936 = property on="DISCO 2" class="Bool (strict)"() -> ("Left"=w794:i32, "Top"=w800:i32)  [unwired: 2 in, 2 out]
        n937 = property on="DISCO 4" class="Bool (strict)"() -> ("Left"=w806:i32, "Top"=w812:i32)  [unwired: 2 in, 2 out]
        n938 = property on="DISCO 5" class="Bool (strict)"() -> ("Left"=w983:i32, "Top"=w989:i32)  [unwired: 2 in, 2 out]
        n939 = property on="DISCO 3" class="Bool (strict)"() -> ("Left"=w1024:i32, "Top"=w1030:i32)  [unwired: 2 in, 2 out]
        n940 = property on="DISCO 5" class="Bool (strict)"() -> ("Left"=w824:i32, "Top"=w818:i32)  [unwired: 2 in, 2 out]
        n941 = property on="DISCO 3" class="Bool (strict)"() -> ("Left"=w783:i32, "Top"=w777:i32)  [unwired: 2 in, 2 out]
        n942 = Greater Or Equal?(x=w1013, y=0) -> (x >= y?=w1015:bool)
        n943 = Less Or Equal?(x=w1013, y=160) -> (x <= y?=w1014:bool)
        n944 = Greater Or Equal?(x=w1007, y=441) -> (x >= y?=w1011:bool)
        n945 = Greater Or Equal?(x=w1001, y=0) -> (x >= y?=w1003:bool)
        n946 = Less Or Equal?(x=w1001, y=160) -> (x <= y?=w1002:bool)
        n947 = Greater Or Equal?(x=w995, y=393) -> (x >= y?=w999:bool)
        n948 = Greater Or Equal?(x=w794, y=350) -> (x >= y?=w792:bool)
        n949 = Less Or Equal?(x=w794, y=500) -> (x <= y?=w793:bool)
        n950 = Greater Or Equal?(x=w800, y=441) -> (x >= y?=w796:bool)
        n951 = Greater Or Equal?(x=w806, y=350) -> (x >= y?=w804:bool)
        n952 = Less Or Equal?(x=w806, y=500) -> (x <= y?=w805:bool)
        n953 = Greater Or Equal?(x=w812, y=393) -> (x >= y?=w808:bool)
        n954 = Greater Or Equal?(x=w983, y=0) -> (x >= y?=w981:bool)
        n955 = Less Or Equal?(x=w983, y=160) -> (x <= y?=w982:bool)
        n956 = Greater Or Equal?(x=w989, y=393) -> (x >= y?=w985:bool)
        n957 = Greater Or Equal?(x=w1024, y=0) -> (x >= y?=w1022:bool)
        n958 = Less Or Equal?(x=w1024, y=160) -> (x <= y?=w1023:bool)
        n959 = Greater Or Equal?(x=w1030, y=393) -> (x >= y?=w1026:bool)
        n960 = Greater Or Equal?(x=w824, y=350) -> (x >= y?=w826:bool)
        n961 = Less Or Equal?(x=w824, y=500) -> (x <= y?=w825:bool)
        n962 = Greater Or Equal?(x=w818, y=393) -> (x >= y?=w822:bool)
        n963 = Greater Or Equal?(x=w783, y=350) -> (x >= y?=w785:bool)
        n964 = Less Or Equal?(x=w783, y=500) -> (x <= y?=w784:bool)
        n965 = Greater Or Equal?(x=w777, y=393) -> (x >= y?=w781:bool)
        n966 = Less Or Equal?(x=w1007, y=489) -> (x <= y?=w1012:bool)
        n967 = Less Or Equal?(x=w995, y=441) -> (x <= y?=w1000:bool)
        n968 = Less Or Equal?(x=w800, y=489) -> (x <= y?=w795:bool)
        n969 = Less Or Equal?(x=w812, y=441) -> (x <= y?=w807:bool)
        n970 = Less Or Equal?(x=w989, y=441) -> (x <= y?=w984:bool)
        n971 = And(x=w1015, y=w1014) -> (x .and. y?=w1009:bool)
        n972 = And(x=w1011, y=w1012) -> (x .and. y?=w1008:bool)
        n973 = Less Or Equal?(x=w1030, y=441) -> (x <= y?=w1025:bool)
        n974 = Less Or Equal?(x=w818, y=441) -> (x <= y?=w823:bool)
        n975 = And(x=w1003, y=w1002) -> (x .and. y?=w997:bool)
        n976 = And(x=w999, y=w1000) -> (x .and. y?=w996:bool)
        n977 = And(x=w792, y=w793) -> (x .and. y?=w798:bool)
        n978 = And(x=w796, y=w795) -> (x .and. y?=w799:bool)
        n979 = Less Or Equal?(x=w777, y=441) -> (x <= y?=w782:bool)
        n980 = And(x=w804, y=w805) -> (x .and. y?=w810:bool)
        n981 = And(x=w808, y=w807) -> (x .and. y?=w811:bool)
        n982 = And(x=w981, y=w982) -> (x .and. y?=w987:bool)
        n983 = And(x=w985, y=w984) -> (x .and. y?=w988:bool)
        n984 = And(x=w1022, y=w1023) -> (x .and. y?=w1028:bool)
        n985 = And(x=w1026, y=w1025) -> (x .and. y?=w1029:bool)
        n986 = And(x=w826, y=w825) -> (x .and. y?=w820:bool)
        n987 = And(x=w822, y=w823) -> (x .and. y?=w819:bool)
        n988 = And(x=w785, y=w784) -> (x .and. y?=w779:bool)
        n989 = And(x=w781, y=w782) -> (x .and. y?=w778:bool)
        n990 = And(x=w1009, y=w1008) -> (x .and. y?=w977:bool)
        n991 = And(x=w997, y=w996) -> (x .and. y?=w993:bool)
        n992 = And(x=w798, y=w799) -> (x .and. y?=w830:bool)
        n993 = And(x=w810, y=w811) -> (x .and. y?=w814:bool)
        n994 = And(x=w987, y=w988) -> (x .and. y?=w976:bool)
        n995 = And(x=w1028, y=w1029) -> (x .and. y?=w994:bool)
        n996 = And(x=w820, y=w819) -> (x .and. y?=w831:bool)
        n997 = And(x=w779, y=w778) -> (x .and. y?=w813:bool)
        n998 = And(x=w977, y=w976) -> (x .and. y?=w975:bool)
        n999 = And(x=w830, y=w831) -> (x .and. y?=w832:bool)
        n1000 = And(x=w977, y=w993) -> (x .and. y?=w991:bool)
        n1001 = And(x=w977, y=w994) -> (x .and. y?=w992:bool)
        n1002 = And(x=w830, y=w814) -> (x .and. y?=w816:bool)
        n1003 = And(x=w830, y=w813) -> (x .and. y?=w815:bool)
        n1004 = Compound Arithmetic op=OR(w992, w991, w975) -> (w990:bool)
        n1005 = Compound Arithmetic op=OR(w815, w816, w832) -> (w817:bool)
        n1006 = case shown="False" w990 {
          frame False {
          }
          frame True {
            n1007 = local write "String"("MOVIMIENTO INCORRECTO" ("String")) -> ()
          }
        }
        n1008 = case shown="False" w817 {
          frame False {
          }
          frame True {
            n1009 = local write "String"("MOVIMIENTO INCORRECTO" ("String")) -> ()
          }
        }
        n1010 = property on="DISCO 4" class="Bool (strict)"() -> ("Left"=w1037:i32, "Top"=w1031:i32)  [unwired: 2 in, 2 out]
        n1011 = property on="DISCO 3" class="Bool (strict)"() -> ("Left"=w1048:i32, "Top"=w1054:i32)  [unwired: 2 in, 2 out]
        n1012 = property on="DISCO 5" class="Bool (strict)"() -> ("Left"=w1060:i32, "Top"=w1066:i32)  [unwired: 2 in, 2 out]
        n1013 = property on="DISCO 4" class="Bool (strict)"() -> ("Left"=w770:i32, "Top"=w776:i32)  [unwired: 2 in, 2 out]
        n1014 = property on="DISCO 3" class="Bool (strict)"() -> ("Left"=w759:i32, "Top"=w753:i32)  [unwired: 2 in, 2 out]
        n1015 = property on="DISCO 5" class="Bool (strict)"() -> ("Left"=w747:i32, "Top"=w741:i32)  [unwired: 2 in, 2 out]
        n1016 = Greater Or Equal?(x=w1037, y=0) -> (x >= y?=w1039:bool)
        n1017 = Less Or Equal?(x=w1037, y=160) -> (x <= y?=w1038:bool)
        n1018 = Greater Or Equal?(x=w1031, y=393) -> (x >= y?=w1035:bool)
        n1019 = Less Or Equal?(x=w1031, y=441) -> (x <= y?=w1036:bool)
        n1020 = Greater Or Equal?(x=w1048, y=0) -> (x >= y?=w1046:bool)
        n1021 = Less Or Equal?(x=w1048, y=160) -> (x <= y?=w1047:bool)
        n1022 = Greater Or Equal?(x=w1054, y=441) -> (x >= y?=w1050:bool)
        n1023 = Less Or Equal?(x=w1054, y=489) -> (x <= y?=w1049:bool)
        n1024 = Greater Or Equal?(x=w1060, y=0) -> (x >= y?=w1058:bool)
        n1025 = Less Or Equal?(x=w1060, y=160) -> (x <= y?=w1059:bool)
        n1026 = Greater Or Equal?(x=w1066, y=393) -> (x >= y?=w1062:bool)
        n1027 = Less Or Equal?(x=w1066, y=441) -> (x <= y?=w1061:bool)
        n1028 = Greater Or Equal?(x=w770, y=350) -> (x >= y?=w768:bool)
        n1029 = Less Or Equal?(x=w770, y=500) -> (x <= y?=w769:bool)
        n1030 = Greater Or Equal?(x=w776, y=393) -> (x >= y?=w772:bool)
        n1031 = Less Or Equal?(x=w776, y=441) -> (x <= y?=w771:bool)
        n1032 = Greater Or Equal?(x=w759, y=350) -> (x >= y?=w761:bool)
        n1033 = Less Or Equal?(x=w759, y=500) -> (x <= y?=w760:bool)
        n1034 = Greater Or Equal?(x=w753, y=441) -> (x >= y?=w757:bool)
        n1035 = Less Or Equal?(x=w753, y=489) -> (x <= y?=w758:bool)
        n1036 = Greater Or Equal?(x=w747, y=350) -> (x >= y?=w749:bool)
        n1037 = Less Or Equal?(x=w747, y=500) -> (x <= y?=w748:bool)
        n1038 = Greater Or Equal?(x=w741, y=393) -> (x >= y?=w745:bool)
        n1039 = Less Or Equal?(x=w741, y=441) -> (x <= y?=w746:bool)
        n1040 = And(x=w1039, y=w1038) -> (x .and. y?=w1033:bool)
        n1041 = And(x=w1035, y=w1036) -> (x .and. y?=w1032:bool)
        n1042 = And(x=w1046, y=w1047) -> (x .and. y?=w1052:bool)
        n1043 = And(x=w1050, y=w1049) -> (x .and. y?=w1053:bool)
        n1044 = And(x=w1058, y=w1059) -> (x .and. y?=w1064:bool)
        n1045 = And(x=w1062, y=w1061) -> (x .and. y?=w1065:bool)
        n1046 = And(x=w768, y=w769) -> (x .and. y?=w774:bool)
        n1047 = And(x=w772, y=w771) -> (x .and. y?=w775:bool)
        n1048 = And(x=w761, y=w760) -> (x .and. y?=w755:bool)
        n1049 = And(x=w757, y=w758) -> (x .and. y?=w754:bool)
        n1050 = And(x=w749, y=w748) -> (x .and. y?=w743:bool)
        n1051 = And(x=w745, y=w746) -> (x .and. y?=w742:bool)
        n1052 = And(x=w1033, y=w1032) -> (x .and. y?=w1067:bool)
        n1053 = And(x=w1052, y=w1053) -> (x .and. y?=w1072:bool)
        n1054 = And(x=w1064, y=w1065) -> (x .and. y?=w1068:bool)
        n1055 = And(x=w774, y=w775) -> (x .and. y?=w740:bool)
        n1056 = And(x=w755, y=w754) -> (x .and. y?=w735:bool)
        n1057 = And(x=w743, y=w742) -> (x .and. y?=w739:bool)
        n1058 = And(x=w1072, y=w1067) -> (x .and. y?=w1069:bool)
        n1059 = And(x=w1072, y=w1068) -> (x .and. y?=w1070:bool)
        n1060 = And(x=w735, y=w740) -> (x .and. y?=w738:bool)
        n1061 = And(x=w735, y=w739) -> (x .and. y?=w737:bool)
        n1062 = Compound Arithmetic op=OR(w1069, w1070) -> (w1071:bool)
        n1063 = Compound Arithmetic op=OR(w738, w737) -> (w736:bool)
        n1064 = case shown="False" w1071 {
          frame False {
          }
          frame True {
            n1065 = local write "String"("MOVIMIENTO INCORRECTO" ("String")) -> ()
          }
        }
        n1066 = case shown="False" w736 {
          frame False {
          }
          frame True {
            n1067 = local write "String"("MOVIMIENTO INCORRECTO" ("String")) -> ()
          }
        }
        n1068 = property on="DISCO 4" class="Bool (strict)"() -> ("Left"=w1079:i32, "Top"=w1073:i32)  [unwired: 2 in, 2 out]
        n1069 = property on="DISCO 5" class="Bool (strict)"() -> ("Left"=w1090:i32, "Top"=w1096:i32)  [unwired: 2 in, 2 out]
        n1070 = property on="DISCO 4" class="Bool (strict)"() -> ("Left"=w728:i32, "Top"=w734:i32)  [unwired: 2 in, 2 out]
        n1071 = property on="DISCO 5" class="Bool (strict)"() -> ("Left"=w717:i32, "Top"=w711:i32)  [unwired: 2 in, 2 out]
        n1072 = Greater Or Equal?(x=w1079, y=0) -> (x >= y?=w1081:bool)
        n1073 = Less Or Equal?(x=w1079, y=160) -> (x <= y?=w1080:bool)
        n1074 = Greater Or Equal?(x=w1073, y=430) -> (x >= y?=w1077:bool)
        n1075 = Less Or Equal?(x=w1073, y=500) -> (x <= y?=w1078:bool)
        n1076 = Greater Or Equal?(x=w1090, y=0) -> (x >= y?=w1088:bool)
        n1077 = Less Or Equal?(x=w1090, y=160) -> (x <= y?=w1089:bool)
        n1078 = Greater Or Equal?(x=w1096, y=380) -> (x >= y?=w1092:bool)
        n1079 = Less Or Equal?(x=w1096, y=441) -> (x <= y?=w1091:bool)
        n1080 = Greater Or Equal?(x=w728, y=350) -> (x >= y?=w726:bool)
        n1081 = Less Or Equal?(x=w728, y=500) -> (x <= y?=w727:bool)
        n1082 = Greater Or Equal?(x=w734, y=430) -> (x >= y?=w730:bool)
        n1083 = Less Or Equal?(x=w734, y=500) -> (x <= y?=w729:bool)
        n1084 = Greater Or Equal?(x=w717, y=330) -> (x >= y?=w719:bool)
        n1085 = Less Or Equal?(x=w717, y=500) -> (x <= y?=w718:bool)
        n1086 = Greater Or Equal?(x=w711, y=380) -> (x >= y?=w715:bool)
        n1087 = Less Or Equal?(x=w711, y=441) -> (x <= y?=w716:bool)
        n1088 = And(x=w1081, y=w1080) -> (x .and. y?=w1075:bool)
        n1089 = And(x=w1077, y=w1078) -> (x .and. y?=w1074:bool)
        n1090 = And(x=w1088, y=w1089) -> (x .and. y?=w1094:bool)
        n1091 = And(x=w1092, y=w1091) -> (x .and. y?=w1095:bool)
        n1092 = And(x=w726, y=w727) -> (x .and. y?=w732:bool)
        n1093 = And(x=w730, y=w729) -> (x .and. y?=w733:bool)
        n1094 = And(x=w719, y=w718) -> (x .and. y?=w713:bool)
        n1095 = And(x=w715, y=w716) -> (x .and. y?=w712:bool)
        n1096 = And(x=w1075, y=w1074) -> (x .and. y?=w1097:bool)
        n1097 = And(x=w1094, y=w1095) -> (x .and. y?=w1099:bool)
        n1098 = And(x=w732, y=w733) -> (x .and. y?=w710:bool)
        n1099 = And(x=w713, y=w712) -> (x .and. y?=w708:bool)
        n1100 = And(x=w1097, y=w1099) -> (x .and. y?=w1098:bool)
        n1101 = And(x=w710, y=w708) -> (x .and. y?=w709:bool)
        n1102 = case shown="False" w1098 {
          frame False {
          }
          frame True {
            n1103 = local write "String"("MOVIMIENTO INCORRECTO" ("String")) -> ()
          }
        }
        n1104 = case shown="False" w709 {
          frame False {
          }
          frame True {
            n1105 = local write "String"("MOVIMIENTO INCORRECTO" ("String")) -> ()
          }
        }
        n1106 = property on="DISCO 2" class="Bool (strict)"() -> ("Left"=w1283:i32, "Top"=w1289:i32)  [unwired: 2 in, 2 out]
        n1107 = property on="DISCO 2" class="Bool (strict)"() -> ("Left"=w522:i32, "Top"=w516:i32)  [unwired: 2 in, 2 out]
        n1108 = property on="DISCO 3" class="Bool (strict)"() -> ("Left"=w1261:i32, "Top"=w1255:i32)  [unwired: 2 in, 2 out]
        n1109 = property on="DISCO 1" class="Bool (strict)"() -> ("Left"=w1272:i32, "Top"=w1267:i32)  [unwired: 2 in, 2 out]
        n1110 = property on="DISCO 4" class="Bool (strict)"() -> ("Left"=w1244:i32, "Top"=w1250:i32)  [unwired: 2 in, 2 out]
        n1111 = property on="DISCO 5" class="Bool (strict)"() -> ("Left"=w1235:i32, "Top"=w1229:i32)  [unwired: 2 in, 2 out]
        n1112 = property on="DISCO 3" class="Bool (strict)"() -> ("Left"=w544:i32, "Top"=w550:i32)  [unwired: 2 in, 2 out]
        n1113 = property on="DISCO 1" class="Bool (strict)"() -> ("Left"=w533:i32, "Top"=w538:i32)  [unwired: 2 in, 2 out]
        n1114 = property on="DISCO 4" class="Bool (strict)"() -> ("Left"=w561:i32, "Top"=w555:i32)  [unwired: 2 in, 2 out]
        n1115 = property on="DISCO 5" class="Bool (strict)"() -> ("Left"=w572:i32, "Top"=w578:i32)  [unwired: 2 in, 2 out]
        n1116 = Greater Or Equal?(x=w1283, y=0) -> (x >= y?=w1281:bool)
        n1117 = Less Or Equal?(x=w1283, y=160) -> (x <= y?=w1282:bool)
        n1118 = Greater Or Equal?(x=w1289, y=345) -> (x >= y?=w1285:bool)
        n1119 = Less Or Equal?(x=w1289, y=393) -> (x <= y?=w1284:bool)
        n1120 = Greater Or Equal?(x=w1261, y=0) -> (x >= y?=w1263:bool)
        n1121 = Less Or Equal?(x=w1261, y=160) -> (x <= y?=w1262:bool)
        n1122 = Greater Or Equal?(x=w1255, y=345) -> (x >= y?=w1259:bool)
        n1123 = Less Or Equal?(x=w1255, y=393) -> (x <= y?=w1260:bool)
        n1124 = Greater Or Equal?(x=w1272, y=0) -> (x >= y?=w1274:bool)
        n1125 = Less Or Equal?(x=w1272, y=160) -> (x <= y?=w1273:bool)
        n1126 = Greater Or Equal?(x=w1267, y=410) -> (x >= y?=w1270:bool)
        n1127 = Less Or Equal?(x=w1267, y=441) -> (x <= y?=w1271:bool)
        n1128 = Greater Or Equal?(x=w1244, y=0) -> (x >= y?=w1242:bool)
        n1129 = Less Or Equal?(x=w1244, y=160) -> (x <= y?=w1243:bool)
        n1130 = Greater Or Equal?(x=w1250, y=345) -> (x >= y?=w1246:bool)
        n1131 = Less Or Equal?(x=w1250, y=393) -> (x <= y?=w1245:bool)
        n1132 = Greater Or Equal?(x=w1235, y=0) -> (x >= y?=w1236:bool)
        n1133 = Less Or Equal?(x=w1235, y=160) -> (x <= y?=w119:bool)
        n1134 = Greater Or Equal?(x=w1229, y=345) -> (x >= y?=w1233:bool)
        n1135 = Less Or Equal?(x=w1229, y=393) -> (x <= y?=w1234:bool)
        n1136 = Greater Or Equal?(x=w522, y=350) -> (x >= y?=w524:bool)
        n1137 = Less Or Equal?(x=w522, y=500) -> (x <= y?=w523:bool)
        n1138 = Greater Or Equal?(x=w516, y=345) -> (x >= y?=w520:bool)
        n1139 = Less Or Equal?(x=w516, y=393) -> (x <= y?=w521:bool)
        n1140 = Greater Or Equal?(x=w544, y=350) -> (x >= y?=w542:bool)
        n1141 = Less Or Equal?(x=w544, y=500) -> (x <= y?=w543:bool)
        n1142 = Greater Or Equal?(x=w550, y=345) -> (x >= y?=w546:bool)
        n1143 = Less Or Equal?(x=w550, y=393) -> (x <= y?=w545:bool)
        n1144 = Greater Or Equal?(x=w533, y=350) -> (x >= y?=w531:bool)
        n1145 = Less Or Equal?(x=w533, y=500) -> (x <= y?=w532:bool)
        n1146 = Greater Or Equal?(x=w538, y=410) -> (x >= y?=w535:bool)
        n1147 = Less Or Equal?(x=w538, y=441) -> (x <= y?=w534:bool)
        n1148 = Greater Or Equal?(x=w561, y=350) -> (x >= y?=w563:bool)
        n1149 = Less Or Equal?(x=w561, y=500) -> (x <= y?=w562:bool)
        n1150 = Greater Or Equal?(x=w555, y=345) -> (x >= y?=w559:bool)
        n1151 = Less Or Equal?(x=w555, y=393) -> (x <= y?=w560:bool)
        n1152 = Greater Or Equal?(x=w572, y=350) -> (x >= y?=w570:bool)
        n1153 = Less Or Equal?(x=w572, y=500) -> (x <= y?=w571:bool)
        n1154 = Greater Or Equal?(x=w578, y=345) -> (x >= y?=w574:bool)
        n1155 = Less Or Equal?(x=w578, y=393) -> (x <= y?=w573:bool)
        n1156 = And(x=w1281, y=w1282) -> (x .and. y?=w1287:bool)
        n1157 = And(x=w1285, y=w1284) -> (x .and. y?=w1288:bool)
        n1158 = And(x=w1263, y=w1262) -> (x .and. y?=w1257:bool)
        n1159 = And(x=w1259, y=w1260) -> (x .and. y?=w1256:bool)
        n1160 = And(x=w1274, y=w1273) -> (x .and. y?=w1290:bool)
        n1161 = And(x=w1270, y=w1271) -> (x .and. y?=w1268:bool)
        n1162 = And(x=w1242, y=w1243) -> (x .and. y?=w1248:bool)
        n1163 = And(x=w1246, y=w1245) -> (x .and. y?=w1249:bool)
        n1164 = And(x=w1236, y=w119) -> (x .and. y?=w1231:bool)
        n1165 = And(x=w1233, y=w1234) -> (x .and. y?=w1230:bool)
        n1166 = And(x=w524, y=w523) -> (x .and. y?=w518:bool)
        n1167 = And(x=w520, y=w521) -> (x .and. y?=w517:bool)
        n1168 = And(x=w542, y=w543) -> (x .and. y?=w548:bool)
        n1169 = And(x=w546, y=w545) -> (x .and. y?=w549:bool)
        n1170 = And(x=w531, y=w532) -> (x .and. y?=w515:bool)
        n1171 = And(x=w535, y=w534) -> (x .and. y?=w537:bool)
        n1172 = And(x=w563, y=w562) -> (x .and. y?=w557:bool)
        n1173 = And(x=w559, y=w560) -> (x .and. y?=w556:bool)
        n1174 = And(x=w570, y=w571) -> (x .and. y?=w576:bool)
        n1175 = And(x=w574, y=w573) -> (x .and. y?=w577:bool)
        n1176 = And(x=w1287, y=w1288) -> (x .and. y?=w1254:bool)
        n1177 = And(x=w1257, y=w1256) -> (x .and. y?=w1253:bool)
        n1178 = And(x=w1290, y=w1268) -> (x .and. y?=w1292:bool)
        n1179 = And(x=w1248, y=w1249) -> (x .and. y?=w1228:bool)
        n1180 = And(x=w1231, y=w1230) -> (x .and. y?=w1227:bool)
        n1181 = And(x=w518, y=w517) -> (x .and. y?=w551:bool)
        n1182 = And(x=w548, y=w549) -> (x .and. y?=w552:bool)
        n1183 = And(x=w515, y=w537) -> (x .and. y?=w513:bool)
        n1184 = And(x=w557, y=w556) -> (x .and. y?=w579:bool)
        n1185 = And(x=w576, y=w577) -> (x .and. y?=w580:bool)
        n1186 = And(x=w1292, y=w1254) -> (x .and. y?=w1252:bool)
        n1187 = And(x=w1292, y=w1253) -> (x .and. y?=w1251:bool)
        n1188 = And(x=w1292, y=w1228) -> (x .and. y?=w1226:bool)
        n1189 = And(x=w1292, y=w1227) -> (x .and. y?=w1225:bool)
        n1190 = And(x=w513, y=w551) -> (x .and. y?=w553:bool)
        n1191 = And(x=w513, y=w552) -> (x .and. y?=w554:bool)
        n1192 = And(x=w513, y=w579) -> (x .and. y?=w581:bool)
        n1193 = And(x=w513, y=w580) -> (x .and. y?=w582:bool)
        n1194 = Compound Arithmetic op=OR(w1252, w1251, w1226, w1225) -> (w1291:bool)
        n1195 = Compound Arithmetic op=OR(w553, w554, w581, w582) -> (w514:bool)
        n1196 = case shown="False" w1291 {
          frame False {
          }
          frame True {
            n1197 = local write "String"("MOVIMIENTO INCORRECTO" ("String")) -> ()
          }
        }
        n1198 = case shown="False" w514 {
          frame False {
          }
          frame True {
            n1199 = local write "String"("MOVIMIENTO INCORRECTO" ("String")) -> ()
          }
        }
        n1200 = property on="DISCO 2" class="Bool (strict)"() -> ("Left"=w1186:i32, "Top"=w1192:i32)  [unwired: 2 in, 2 out]
        n1201 = property on="DISCO 4" class="Bool (strict)"() -> ("Left"=w1198:i32, "Top"=w1204:i32)  [unwired: 2 in, 2 out]
        n1202 = property on="DISCO 2" class="Bool (strict)"() -> ("Left"=w621:i32, "Top"=w615:i32)  [unwired: 2 in, 2 out]
        n1203 = property on="DISCO 4" class="Bool (strict)"() -> ("Left"=w609:i32, "Top"=w603:i32)  [unwired: 2 in, 2 out]
        n1204 = property on="DISCO 5" class="Bool (strict)"() -> ("Left"=w1216:i32, "Top"=w1210:i32)  [unwired: 2 in, 2 out]
        n1205 = property on="DISCO 3" class="Bool (strict)"() -> ("Left"=w1175:i32, "Top"=w1169:i32)  [unwired: 2 in, 2 out]
        n1206 = property on="DISCO 5" class="Bool (strict)"() -> ("Left"=w591:i32, "Top"=w597:i32)  [unwired: 2 in, 2 out]
        n1207 = property on="DISCO 3" class="Bool (strict)"() -> ("Left"=w632:i32, "Top"=w638:i32)  [unwired: 2 in, 2 out]
        n1208 = Greater Or Equal?(x=w1186, y=0) -> (x >= y?=w1184:bool)
        n1209 = Less Or Equal?(x=w1186, y=160) -> (x <= y?=w1185:bool)
        n1210 = Greater Or Equal?(x=w1192, y=393) -> (x >= y?=w1188:bool)
        n1211 = Greater Or Equal?(x=w1198, y=0) -> (x >= y?=w1196:bool)
        n1212 = Less Or Equal?(x=w1198, y=160) -> (x <= y?=w1197:bool)
        n1213 = Greater Or Equal?(x=w1204, y=345) -> (x >= y?=w1200:bool)
        n1214 = Greater Or Equal?(x=w621, y=350) -> (x >= y?=w623:bool)
        n1215 = Less Or Equal?(x=w621, y=500) -> (x <= y?=w622:bool)
        n1216 = Greater Or Equal?(x=w615, y=393) -> (x >= y?=w619:bool)
        n1217 = Greater Or Equal?(x=w609, y=350) -> (x >= y?=w611:bool)
        n1218 = Less Or Equal?(x=w609, y=500) -> (x <= y?=w610:bool)
        n1219 = Greater Or Equal?(x=w603, y=345) -> (x >= y?=w607:bool)
        n1220 = Greater Or Equal?(x=w1216, y=0) -> (x >= y?=w1218:bool)
        n1221 = Less Or Equal?(x=w1216, y=160) -> (x <= y?=w1217:bool)
        n1222 = Greater Or Equal?(x=w1210, y=345) -> (x >= y?=w1214:bool)
        n1223 = Greater Or Equal?(x=w1175, y=0) -> (x >= y?=w1177:bool)
        n1224 = Less Or Equal?(x=w1175, y=160) -> (x <= y?=w1176:bool)
        n1225 = Greater Or Equal?(x=w1169, y=345) -> (x >= y?=w1173:bool)
        n1226 = Greater Or Equal?(x=w591, y=350) -> (x >= y?=w589:bool)
        n1227 = Less Or Equal?(x=w591, y=500) -> (x <= y?=w590:bool)
        n1228 = Greater Or Equal?(x=w597, y=345) -> (x >= y?=w593:bool)
        n1229 = Greater Or Equal?(x=w632, y=350) -> (x >= y?=w630:bool)
        n1230 = Less Or Equal?(x=w632, y=500) -> (x <= y?=w631:bool)
        n1231 = Greater Or Equal?(x=w638, y=345) -> (x >= y?=w634:bool)
        n1232 = Less Or Equal?(x=w1192, y=441) -> (x <= y?=w1187:bool)
        n1233 = Less Or Equal?(x=w1204, y=393) -> (x <= y?=w1199:bool)
        n1234 = Less Or Equal?(x=w615, y=441) -> (x <= y?=w620:bool)
        n1235 = Less Or Equal?(x=w603, y=393) -> (x <= y?=w608:bool)
        n1236 = Less Or Equal?(x=w1210, y=393) -> (x <= y?=w1215:bool)
        n1237 = And(x=w1184, y=w1185) -> (x .and. y?=w1190:bool)
        n1238 = And(x=w1188, y=w1187) -> (x .and. y?=w1191:bool)
        n1239 = Less Or Equal?(x=w1169, y=393) -> (x <= y?=w1174:bool)
        n1240 = Less Or Equal?(x=w597, y=393) -> (x <= y?=w592:bool)
        n1241 = And(x=w1196, y=w1197) -> (x .and. y?=w1202:bool)
        n1242 = And(x=w1200, y=w1199) -> (x .and. y?=w1203:bool)
        n1243 = And(x=w623, y=w622) -> (x .and. y?=w617:bool)
        n1244 = And(x=w619, y=w620) -> (x .and. y?=w616:bool)
        n1245 = Less Or Equal?(x=w638, y=393) -> (x <= y?=w633:bool)
        n1246 = And(x=w611, y=w610) -> (x .and. y?=w605:bool)
        n1247 = And(x=w607, y=w608) -> (x .and. y?=w604:bool)
        n1248 = And(x=w1218, y=w1217) -> (x .and. y?=w1212:bool)
        n1249 = And(x=w1214, y=w1215) -> (x .and. y?=w1211:bool)
        n1250 = And(x=w1177, y=w1176) -> (x .and. y?=w1171:bool)
        n1251 = And(x=w1173, y=w1174) -> (x .and. y?=w1170:bool)
        n1252 = And(x=w589, y=w590) -> (x .and. y?=w595:bool)
        n1253 = And(x=w593, y=w592) -> (x .and. y?=w596:bool)
        n1254 = And(x=w630, y=w631) -> (x .and. y?=w636:bool)
        n1255 = And(x=w634, y=w633) -> (x .and. y?=w637:bool)
        n1256 = And(x=w1190, y=w1191) -> (x .and. y?=w1222:bool)
        n1257 = And(x=w1202, y=w1203) -> (x .and. y?=w1206:bool)
        n1258 = And(x=w617, y=w616) -> (x .and. y?=w585:bool)
        n1259 = And(x=w605, y=w604) -> (x .and. y?=w601:bool)
        n1260 = And(x=w1212, y=w1211) -> (x .and. y?=w1223:bool)
        n1261 = And(x=w1171, y=w1170) -> (x .and. y?=w1205:bool)
        n1262 = And(x=w595, y=w596) -> (x .and. y?=w584:bool)
        n1263 = And(x=w636, y=w637) -> (x .and. y?=w602:bool)
        n1264 = And(x=w1222, y=w1223) -> (x .and. y?=w1224:bool)
        n1265 = And(x=w585, y=w584) -> (x .and. y?=w583:bool)
        n1266 = And(x=w1222, y=w1206) -> (x .and. y?=w1208:bool)
        n1267 = And(x=w1222, y=w1205) -> (x .and. y?=w1207:bool)
        n1268 = And(x=w585, y=w601) -> (x .and. y?=w599:bool)
        n1269 = And(x=w585, y=w602) -> (x .and. y?=w600:bool)
        n1270 = Compound Arithmetic op=OR(w1207, w1208, w1224) -> (w1209:bool)
        n1271 = Compound Arithmetic op=OR(w600, w599, w583) -> (w598:bool)
        n1272 = case shown="False" w1209 {
          frame False {
          }
          frame True {
            n1273 = local write "String"("MOVIMIENTO INCORRECTO" ("String")) -> ()
          }
        }
        n1274 = case shown="False" w598 {
          frame False {
          }
          frame True {
            n1275 = local write "String"("MOVIMIENTO INCORRECTO" ("String")) -> ()
          }
        }
        n1276 = property on="DISCO 4" class="Bool (strict)"() -> ("Left"=w1162:i32, "Top"=w1168:i32)  [unwired: 2 in, 2 out]
        n1277 = property on="DISCO 3" class="Bool (strict)"() -> ("Left"=w1151:i32, "Top"=w1145:i32)  [unwired: 2 in, 2 out]
        n1278 = property on="DISCO 5" class="Bool (strict)"() -> ("Left"=w1139:i32, "Top"=w1133:i32)  [unwired: 2 in, 2 out]
        n1279 = property on="DISCO 4" class="Bool (strict)"() -> ("Left"=w645:i32, "Top"=w639:i32)  [unwired: 2 in, 2 out]
        n1280 = property on="DISCO 3" class="Bool (strict)"() -> ("Left"=w656:i32, "Top"=w662:i32)  [unwired: 2 in, 2 out]
        n1281 = property on="DISCO 5" class="Bool (strict)"() -> ("Left"=w668:i32, "Top"=w674:i32)  [unwired: 2 in, 2 out]
        n1282 = Greater Or Equal?(x=w1162, y=0) -> (x >= y?=w1160:bool)
        n1283 = Less Or Equal?(x=w1162, y=160) -> (x <= y?=w1161:bool)
        n1284 = Greater Or Equal?(x=w1168, y=345) -> (x >= y?=w1164:bool)
        n1285 = Less Or Equal?(x=w1168, y=393) -> (x <= y?=w1163:bool)
        n1286 = Greater Or Equal?(x=w1151, y=0) -> (x >= y?=w1153:bool)
        n1287 = Less Or Equal?(x=w1151, y=160) -> (x <= y?=w1152:bool)
        n1288 = Greater Or Equal?(x=w1145, y=393) -> (x >= y?=w1149:bool)
        n1289 = Less Or Equal?(x=w1145, y=441) -> (x <= y?=w1150:bool)
        n1290 = Greater Or Equal?(x=w1139, y=0) -> (x >= y?=w1141:bool)
        n1291 = Less Or Equal?(x=w1139, y=160) -> (x <= y?=w1140:bool)
        n1292 = Greater Or Equal?(x=w1133, y=345) -> (x >= y?=w1137:bool)
        n1293 = Less Or Equal?(x=w1133, y=393) -> (x <= y?=w1138:bool)
        n1294 = Greater Or Equal?(x=w645, y=350) -> (x >= y?=w647:bool)
        n1295 = Less Or Equal?(x=w645, y=500) -> (x <= y?=w646:bool)
        n1296 = Greater Or Equal?(x=w639, y=345) -> (x >= y?=w643:bool)
        n1297 = Less Or Equal?(x=w639, y=393) -> (x <= y?=w644:bool)
        n1298 = Greater Or Equal?(x=w656, y=350) -> (x >= y?=w654:bool)
        n1299 = Less Or Equal?(x=w656, y=500) -> (x <= y?=w655:bool)
        n1300 = Greater Or Equal?(x=w662, y=393) -> (x >= y?=w658:bool)
        n1301 = Less Or Equal?(x=w662, y=441) -> (x <= y?=w657:bool)
        n1302 = Greater Or Equal?(x=w668, y=350) -> (x >= y?=w666:bool)
        n1303 = Less Or Equal?(x=w668, y=500) -> (x <= y?=w667:bool)
        n1304 = Greater Or Equal?(x=w674, y=345) -> (x >= y?=w670:bool)
        n1305 = Less Or Equal?(x=w674, y=393) -> (x <= y?=w669:bool)
        n1306 = And(x=w1160, y=w1161) -> (x .and. y?=w1166:bool)
        n1307 = And(x=w1164, y=w1163) -> (x .and. y?=w1167:bool)
        n1308 = And(x=w1153, y=w1152) -> (x .and. y?=w1147:bool)
        n1309 = And(x=w1149, y=w1150) -> (x .and. y?=w1146:bool)
        n1310 = And(x=w1141, y=w1140) -> (x .and. y?=w1135:bool)
        n1311 = And(x=w1137, y=w1138) -> (x .and. y?=w1134:bool)
        n1312 = And(x=w647, y=w646) -> (x .and. y?=w641:bool)
        n1313 = And(x=w643, y=w644) -> (x .and. y?=w640:bool)
        n1314 = And(x=w654, y=w655) -> (x .and. y?=w660:bool)
        n1315 = And(x=w658, y=w657) -> (x .and. y?=w661:bool)
        n1316 = And(x=w666, y=w667) -> (x .and. y?=w672:bool)
        n1317 = And(x=w670, y=w669) -> (x .and. y?=w673:bool)
        n1318 = And(x=w1166, y=w1167) -> (x .and. y?=w1132:bool)
        n1319 = And(x=w1147, y=w1146) -> (x .and. y?=w1127:bool)
        n1320 = And(x=w1135, y=w1134) -> (x .and. y?=w1131:bool)
        n1321 = And(x=w641, y=w640) -> (x .and. y?=w675:bool)
        n1322 = And(x=w660, y=w661) -> (x .and. y?=w680:bool)
        n1323 = And(x=w672, y=w673) -> (x .and. y?=w676:bool)
        n1324 = And(x=w1127, y=w1132) -> (x .and. y?=w1130:bool)
        n1325 = And(x=w1127, y=w1131) -> (x .and. y?=w1129:bool)
        n1326 = And(x=w680, y=w675) -> (x .and. y?=w677:bool)
        n1327 = And(x=w680, y=w676) -> (x .and. y?=w678:bool)
        n1328 = Compound Arithmetic op=OR(w1130, w1129) -> (w1128:bool)
        n1329 = Compound Arithmetic op=OR(w677, w678) -> (w679:bool)
        n1330 = case shown="False" w1128 {
          frame False {
          }
          frame True {
            n1331 = local write "String"("MOVIMIENTO INCORRECTO" ("String")) -> ()
          }
        }
        n1332 = case shown="False" w679 {
          frame False {
          }
          frame True {
            n1333 = local write "String"("MOVIMIENTO INCORRECTO" ("String")) -> ()
          }
        }
        n1334 = property on="DISCO 4" class="Bool (strict)"() -> ("Left"=w1120:i32, "Top"=w1126:i32)  [unwired: 2 in, 2 out]
        n1335 = property on="DISCO 5" class="Bool (strict)"() -> ("Left"=w1109:i32, "Top"=w1103:i32)  [unwired: 2 in, 2 out]
        n1336 = property on="DISCO 4" class="Bool (strict)"() -> ("Left"=w687:i32, "Top"=w681:i32)  [unwired: 2 in, 2 out]
        n1337 = property on="DISCO 5" class="Bool (strict)"() -> ("Left"=w698:i32, "Top"=w704:i32)  [unwired: 2 in, 2 out]
        n1338 = Greater Or Equal?(x=w1120, y=0) -> (x >= y?=w1118:bool)
        n1339 = Less Or Equal?(x=w1120, y=160) -> (x <= y?=w1119:bool)
        n1340 = Greater Or Equal?(x=w1126, y=380) -> (x >= y?=w1122:bool)
        n1341 = Less Or Equal?(x=w1126, y=441) -> (x <= y?=w1121:bool)
        n1342 = Greater Or Equal?(x=w1109, y=0) -> (x >= y?=w1111:bool)
        n1343 = Less Or Equal?(x=w1109, y=160) -> (x <= y?=w1110:bool)
        n1344 = Greater Or Equal?(x=w1103, y=330) -> (x >= y?=w1107:bool)
        n1345 = Less Or Equal?(x=w1103, y=393) -> (x <= y?=w1108:bool)
        n1346 = Greater Or Equal?(x=w687, y=330) -> (x >= y?=w689:bool)
        n1347 = Less Or Equal?(x=w687, y=500) -> (x <= y?=w688:bool)
        n1348 = Greater Or Equal?(x=w681, y=380) -> (x >= y?=w685:bool)
        n1349 = Less Or Equal?(x=w681, y=441) -> (x <= y?=w686:bool)
        n1350 = Greater Or Equal?(x=w698, y=330) -> (x >= y?=w696:bool)
        n1351 = Less Or Equal?(x=w698, y=500) -> (x <= y?=w697:bool)
        n1352 = Greater Or Equal?(x=w704, y=330) -> (x >= y?=w700:bool)
        n1353 = Less Or Equal?(x=w704, y=393) -> (x <= y?=w699:bool)
        n1354 = And(x=w1118, y=w1119) -> (x .and. y?=w1124:bool)
        n1355 = And(x=w1122, y=w1121) -> (x .and. y?=w1125:bool)
        n1356 = And(x=w1111, y=w1110) -> (x .and. y?=w1105:bool)
        n1357 = And(x=w1107, y=w1108) -> (x .and. y?=w1104:bool)
        n1358 = And(x=w689, y=w688) -> (x .and. y?=w683:bool)
        n1359 = And(x=w685, y=w686) -> (x .and. y?=w682:bool)
        n1360 = And(x=w696, y=w697) -> (x .and. y?=w702:bool)
        n1361 = And(x=w700, y=w699) -> (x .and. y?=w703:bool)
        n1362 = And(x=w1124, y=w1125) -> (x .and. y?=w1102:bool)
        n1363 = And(x=w1105, y=w1104) -> (x .and. y?=w1100:bool)
        n1364 = And(x=w683, y=w682) -> (x .and. y?=w705:bool)
        n1365 = And(x=w702, y=w703) -> (x .and. y?=w707:bool)
        n1366 = And(x=w1102, y=w1100) -> (x .and. y?=w1101:bool)
        n1367 = And(x=w705, y=w707) -> (x .and. y?=w706:bool)
        n1368 = case shown="False" w1101 {
          frame False {
          }
          frame True {
            n1369 = local write "String"("MOVIMIENTO INCORRECTO" ("String")) -> ()
          }
        }
        n1370 = case shown="False" w706 {
          frame False {
          }
          frame True {
            n1371 = local write "String"("MOVIMIENTO INCORRECTO" ("String")) -> ()
          }
        }
        n1372 = property on="DISCO 2" class="Bool (strict)"() -> ("Left"=w1302:i32, "Top"=w1296:i32)  [unwired: 2 in, 2 out]
        n1373 = property on="DISCO 2" class="Bool (strict)"() -> ("Left"=w503:i32, "Top"=w509:i32)  [unwired: 2 in, 2 out]
        n1374 = property on="DISCO 3" class="Bool (strict)"() -> ("Left"=w1324:i32, "Top"=w1330:i32)  [unwired: 2 in, 2 out]
        n1375 = property on="DISCO 1" class="Bool (strict)"() -> ("Left"=w1313:i32, "Top"=w1318:i32)  [unwired: 2 in, 2 out]
        n1376 = property on="DISCO 4" class="Bool (strict)"() -> ("Left"=w1341:i32, "Top"=w1335:i32)  [unwired: 2 in, 2 out]
        n1377 = property on="DISCO 5" class="Bool (strict)"() -> ("Left"=w1352:i32, "Top"=w1358:i32)  [unwired: 2 in, 2 out]
        n1378 = property on="DISCO 3" class="Bool (strict)"() -> ("Left"=w481:i32, "Top"=w475:i32)  [unwired: 2 in, 2 out]
        n1379 = property on="DISCO 1" class="Bool (strict)"() -> ("Left"=w492:i32, "Top"=w487:i32)  [unwired: 2 in, 2 out]
        n1380 = property on="DISCO 4" class="Bool (strict)"() -> ("Left"=w464:i32, "Top"=w470:i32)  [unwired: 2 in, 2 out]
        n1381 = property on="DISCO 5" class="Bool (strict)"() -> ("Left"=w453:i32, "Top"=w447:i32)  [unwired: 2 in, 2 out]
        n1382 = Greater Or Equal?(x=w1302, y=0) -> (x >= y?=w1304:bool)
        n1383 = Less Or Equal?(x=w1302, y=160) -> (x <= y?=w1303:bool)
        n1384 = Greater Or Equal?(x=w1296, y=297) -> (x >= y?=w1300:bool)
        n1385 = Less Or Equal?(x=w1296, y=345) -> (x <= y?=w1301:bool)
        n1386 = Greater Or Equal?(x=w1324, y=0) -> (x >= y?=w1322:bool)
        n1387 = Less Or Equal?(x=w1324, y=160) -> (x <= y?=w1323:bool)
        n1388 = Greater Or Equal?(x=w1330, y=297) -> (x >= y?=w1326:bool)
        n1389 = Less Or Equal?(x=w1330, y=345) -> (x <= y?=w1325:bool)
        n1390 = Greater Or Equal?(x=w1313, y=0) -> (x >= y?=w1311:bool)
        n1391 = Less Or Equal?(x=w1313, y=160) -> (x <= y?=w1312:bool)
        n1392 = Greater Or Equal?(x=w1318, y=345) -> (x >= y?=w1315:bool)
        n1393 = Less Or Equal?(x=w1318, y=410) -> (x <= y?=w1314:bool)
        n1394 = Greater Or Equal?(x=w1341, y=0) -> (x >= y?=w1343:bool)
        n1395 = Less Or Equal?(x=w1341, y=160) -> (x <= y?=w1342:bool)
        n1396 = Greater Or Equal?(x=w1335, y=297) -> (x >= y?=w1339:bool)
        n1397 = Less Or Equal?(x=w1335, y=345) -> (x <= y?=w1340:bool)
        n1398 = Greater Or Equal?(x=w1352, y=0) -> (x >= y?=w1350:bool)
        n1399 = Less Or Equal?(x=w1352, y=160) -> (x <= y?=w1351:bool)
        n1400 = Greater Or Equal?(x=w1358, y=297) -> (x >= y?=w1354:bool)
        n1401 = Less Or Equal?(x=w1358, y=345) -> (x <= y?=w1353:bool)
        n1402 = Greater Or Equal?(x=w503, y=350) -> (x >= y?=w501:bool)
        n1403 = Less Or Equal?(x=w503, y=500) -> (x <= y?=w502:bool)
        n1404 = Greater Or Equal?(x=w509, y=297) -> (x >= y?=w505:bool)
        n1405 = Less Or Equal?(x=w509, y=345) -> (x <= y?=w504:bool)
        n1406 = Greater Or Equal?(x=w481, y=350) -> (x >= y?=w483:bool)
        n1407 = Less Or Equal?(x=w481, y=500) -> (x <= y?=w482:bool)
        n1408 = Greater Or Equal?(x=w475, y=297) -> (x >= y?=w479:bool)
        n1409 = Less Or Equal?(x=w475, y=345) -> (x <= y?=w480:bool)
        n1410 = Greater Or Equal?(x=w492, y=350) -> (x >= y?=w494:bool)
        n1411 = Less Or Equal?(x=w492, y=500) -> (x <= y?=w493:bool)
        n1412 = Greater Or Equal?(x=w487, y=345) -> (x >= y?=w490:bool)
        n1413 = Less Or Equal?(x=w487, y=410) -> (x <= y?=w491:bool)
        n1414 = Greater Or Equal?(x=w464, y=350) -> (x >= y?=w462:bool)
        n1415 = Less Or Equal?(x=w464, y=500) -> (x <= y?=w463:bool)
        n1416 = Greater Or Equal?(x=w470, y=297) -> (x >= y?=w466:bool)
        n1417 = Less Or Equal?(x=w470, y=345) -> (x <= y?=w465:bool)
        n1418 = Greater Or Equal?(x=w453, y=350) -> (x >= y?=w455:bool)
        n1419 = Less Or Equal?(x=w453, y=500) -> (x <= y?=w454:bool)
        n1420 = Greater Or Equal?(x=w447, y=297) -> (x >= y?=w451:bool)
        n1421 = Less Or Equal?(x=w447, y=345) -> (x <= y?=w452:bool)
        n1422 = And(x=w1304, y=w1303) -> (x .and. y?=w1298:bool)
        n1423 = And(x=w1300, y=w1301) -> (x .and. y?=w1297:bool)
        n1424 = And(x=w1322, y=w1323) -> (x .and. y?=w1328:bool)
        n1425 = And(x=w1326, y=w1325) -> (x .and. y?=w1329:bool)
        n1426 = And(x=w1311, y=w1312) -> (x .and. y?=w1295:bool)
        n1427 = And(x=w1315, y=w1314) -> (x .and. y?=w1317:bool)
        n1428 = And(x=w1343, y=w1342) -> (x .and. y?=w1337:bool)
        n1429 = And(x=w1339, y=w1340) -> (x .and. y?=w1336:bool)
        n1430 = And(x=w1350, y=w1351) -> (x .and. y?=w1356:bool)
        n1431 = And(x=w1354, y=w1353) -> (x .and. y?=w1357:bool)
        n1432 = And(x=w501, y=w502) -> (x .and. y?=w507:bool)
        n1433 = And(x=w505, y=w504) -> (x .and. y?=w508:bool)
        n1434 = And(x=w483, y=w482) -> (x .and. y?=w477:bool)
        n1435 = And(x=w479, y=w480) -> (x .and. y?=w476:bool)
        n1436 = And(x=w494, y=w493) -> (x .and. y?=w510:bool)
        n1437 = And(x=w490, y=w491) -> (x .and. y?=w488:bool)
        n1438 = And(x=w462, y=w463) -> (x .and. y?=w468:bool)
        n1439 = And(x=w466, y=w465) -> (x .and. y?=w469:bool)
        n1440 = And(x=w455, y=w454) -> (x .and. y?=w449:bool)
        n1441 = And(x=w451, y=w452) -> (x .and. y?=w448:bool)
        n1442 = And(x=w1298, y=w1297) -> (x .and. y?=w1331:bool)
        n1443 = And(x=w1328, y=w1329) -> (x .and. y?=w1332:bool)
        n1444 = And(x=w1295, y=w1317) -> (x .and. y?=w1293:bool)
        n1445 = And(x=w1337, y=w1336) -> (x .and. y?=w1359:bool)
        n1446 = And(x=w1356, y=w1357) -> (x .and. y?=w1360:bool)
        n1447 = And(x=w507, y=w508) -> (x .and. y?=w474:bool)
        n1448 = And(x=w477, y=w476) -> (x .and. y?=w473:bool)
        n1449 = And(x=w510, y=w488) -> (x .and. y?=w512:bool)
        n1450 = And(x=w468, y=w469) -> (x .and. y?=w446:bool)
        n1451 = And(x=w449, y=w448) -> (x .and. y?=w445:bool)
        n1452 = And(x=w1293, y=w1331) -> (x .and. y?=w1333:bool)
        n1453 = And(x=w1293, y=w1332) -> (x .and. y?=w1334:bool)
        n1454 = And(x=w1293, y=w1359) -> (x .and. y?=w1361:bool)
        n1455 = And(x=w1293, y=w1360) -> (x .and. y?=w1362:bool)
        n1456 = And(x=w512, y=w474) -> (x .and. y?=w472:bool)
        n1457 = And(x=w512, y=w473) -> (x .and. y?=w471:bool)
        n1458 = And(x=w512, y=w446) -> (x .and. y?=w444:bool)
        n1459 = And(x=w512, y=w445) -> (x .and. y?=w443:bool)
        n1460 = Compound Arithmetic op=OR(w1333, w1334, w1361, w1362) -> (w1294:bool)
        n1461 = Compound Arithmetic op=OR(w472, w471, w444, w443) -> (w511:bool)
        n1462 = case shown="False" w1294 {
          frame False {
          }
          frame True {
            n1463 = local write "String"("MOVIMIENTO INCORRECTO" ("String")) -> ()
          }
        }
        n1464 = case shown="False" w511 {
          frame False {
          }
          frame True {
            n1465 = local write "String"("MOVIMIENTO INCORRECTO" ("String")) -> ()
          }
        }
        n1466 = property on="DISCO 2" class="Bool (strict)"() -> ("Left"=w1401:i32, "Top"=w1395:i32)  [unwired: 2 in, 2 out]
        n1467 = property on="DISCO 4" class="Bool (strict)"() -> ("Left"=w1389:i32, "Top"=w1383:i32)  [unwired: 2 in, 2 out]
        n1468 = property on="DISCO 2" class="Bool (strict)"() -> ("Left"=w404:i32, "Top"=w410:i32)  [unwired: 2 in, 2 out]
        n1469 = property on="DISCO 4" class="Bool (strict)"() -> ("Left"=w416:i32, "Top"=w422:i32)  [unwired: 2 in, 2 out]
        n1470 = property on="DISCO 5" class="Bool (strict)"() -> ("Left"=w1371:i32, "Top"=w1377:i32)  [unwired: 2 in, 2 out]
        n1471 = property on="DISCO 3" class="Bool (strict)"() -> ("Left"=w1412:i32, "Top"=w1418:i32)  [unwired: 2 in, 2 out]
        n1472 = property on="DISCO 5" class="Bool (strict)"() -> ("Left"=w434:i32, "Top"=w428:i32)  [unwired: 2 in, 2 out]
        n1473 = property on="DISCO 3" class="Bool (strict)"() -> ("Left"=w393:i32, "Top"=w387:i32)  [unwired: 2 in, 2 out]
        n1474 = Greater Or Equal?(x=w1401, y=0) -> (x >= y?=w1403:bool)
        n1475 = Less Or Equal?(x=w1401, y=160) -> (x <= y?=w1402:bool)
        n1476 = Greater Or Equal?(x=w1395, y=345) -> (x >= y?=w1399:bool)
        n1477 = Greater Or Equal?(x=w1389, y=0) -> (x >= y?=w1391:bool)
        n1478 = Less Or Equal?(x=w1389, y=160) -> (x <= y?=w1390:bool)
        n1479 = Greater Or Equal?(x=w1383, y=297) -> (x >= y?=w1387:bool)
        n1480 = Greater Or Equal?(x=w404, y=350) -> (x >= y?=w402:bool)
        n1481 = Less Or Equal?(x=w404, y=500) -> (x <= y?=w403:bool)
        n1482 = Greater Or Equal?(x=w410, y=345) -> (x >= y?=w406:bool)
        n1483 = Greater Or Equal?(x=w416, y=350) -> (x >= y?=w414:bool)
        n1484 = Less Or Equal?(x=w416, y=500) -> (x <= y?=w415:bool)
        n1485 = Greater Or Equal?(x=w422, y=297) -> (x >= y?=w418:bool)
        n1486 = Greater Or Equal?(x=w1371, y=0) -> (x >= y?=w1369:bool)
        n1487 = Less Or Equal?(x=w1371, y=160) -> (x <= y?=w1370:bool)
        n1488 = Greater Or Equal?(x=w1377, y=297) -> (x >= y?=w1373:bool)
        n1489 = Greater Or Equal?(x=w1412, y=0) -> (x >= y?=w1410:bool)
        n1490 = Less Or Equal?(x=w1412, y=160) -> (x <= y?=w1411:bool)
        n1491 = Greater Or Equal?(x=w1418, y=297) -> (x >= y?=w1414:bool)
        n1492 = Greater Or Equal?(x=w434, y=350) -> (x >= y?=w436:bool)
        n1493 = Less Or Equal?(x=w434, y=500) -> (x <= y?=w435:bool)
        n1494 = Greater Or Equal?(x=w428, y=297) -> (x >= y?=w432:bool)
        n1495 = Greater Or Equal?(x=w393, y=350) -> (x >= y?=w395:bool)
        n1496 = Less Or Equal?(x=w393, y=500) -> (x <= y?=w394:bool)
        n1497 = Greater Or Equal?(x=w387, y=297) -> (x >= y?=w391:bool)
        n1498 = Less Or Equal?(x=w1395, y=410) -> (x <= y?=w1400:bool)
        n1499 = Less Or Equal?(x=w1383, y=345) -> (x <= y?=w1388:bool)
        n1500 = Less Or Equal?(x=w410, y=410) -> (x <= y?=w405:bool)
        n1501 = Less Or Equal?(x=w422, y=345) -> (x <= y?=w417:bool)
        n1502 = Less Or Equal?(x=w1377, y=345) -> (x <= y?=w1372:bool)
        n1503 = And(x=w1403, y=w1402) -> (x .and. y?=w1397:bool)
        n1504 = And(x=w1399, y=w1400) -> (x .and. y?=w1396:bool)
        n1505 = Less Or Equal?(x=w1418, y=345) -> (x <= y?=w1413:bool)
        n1506 = Less Or Equal?(x=w428, y=345) -> (x <= y?=w433:bool)
        n1507 = And(x=w1391, y=w1390) -> (x .and. y?=w1385:bool)
        n1508 = And(x=w1387, y=w1388) -> (x .and. y?=w1384:bool)
        n1509 = And(x=w402, y=w403) -> (x .and. y?=w408:bool)
        n1510 = And(x=w406, y=w405) -> (x .and. y?=w409:bool)
        n1511 = Less Or Equal?(x=w387, y=345) -> (x <= y?=w392:bool)
        n1512 = And(x=w414, y=w415) -> (x .and. y?=w420:bool)
        n1513 = And(x=w418, y=w417) -> (x .and. y?=w421:bool)
        n1514 = And(x=w1369, y=w1370) -> (x .and. y?=w1375:bool)
        n1515 = And(x=w1373, y=w1372) -> (x .and. y?=w1376:bool)
        n1516 = And(x=w1410, y=w1411) -> (x .and. y?=w1416:bool)
        n1517 = And(x=w1414, y=w1413) -> (x .and. y?=w1417:bool)
        n1518 = And(x=w436, y=w435) -> (x .and. y?=w430:bool)
        n1519 = And(x=w432, y=w433) -> (x .and. y?=w429:bool)
        n1520 = And(x=w395, y=w394) -> (x .and. y?=w389:bool)
        n1521 = And(x=w391, y=w392) -> (x .and. y?=w388:bool)
        n1522 = And(x=w1397, y=w1396) -> (x .and. y?=w1365:bool)
        n1523 = And(x=w1385, y=w1384) -> (x .and. y?=w1381:bool)
        n1524 = And(x=w408, y=w409) -> (x .and. y?=w440:bool)
        n1525 = And(x=w420, y=w421) -> (x .and. y?=w424:bool)
        n1526 = And(x=w1375, y=w1376) -> (x .and. y?=w1364:bool)
        n1527 = And(x=w1416, y=w1417) -> (x .and. y?=w1382:bool)
        n1528 = And(x=w430, y=w429) -> (x .and. y?=w441:bool)
        n1529 = And(x=w389, y=w388) -> (x .and. y?=w423:bool)
        n1530 = And(x=w1365, y=w1364) -> (x .and. y?=w1363:bool)
        n1531 = And(x=w440, y=w441) -> (x .and. y?=w442:bool)
        n1532 = And(x=w1365, y=w1381) -> (x .and. y?=w1379:bool)
        n1533 = And(x=w1365, y=w1382) -> (x .and. y?=w1380:bool)
        n1534 = And(x=w440, y=w424) -> (x .and. y?=w426:bool)
        n1535 = And(x=w440, y=w423) -> (x .and. y?=w425:bool)
        n1536 = Compound Arithmetic op=OR(w1380, w1379, w1363) -> (w1378:bool)
        n1537 = Compound Arithmetic op=OR(w425, w426, w442) -> (w427:bool)
        n1538 = case shown="False" w1378 {
          frame False {
          }
          frame True {
            n1539 = local write "String"("MOVIMIENTO INCORRECTO" ("String")) -> ()
          }
        }
        n1540 = case shown="False" w427 {
          frame False {
          }
          frame True {
            n1541 = local write "String"("MOVIMIENTO INCORRECTO" ("String")) -> ()
          }
        }
        n1542 = property on="DISCO 4" class="Bool (strict)"() -> ("Left"=w1425:i32, "Top"=w1419:i32)  [unwired: 2 in, 2 out]
        n1543 = property on="DISCO 3" class="Bool (strict)"() -> ("Left"=w1436:i32, "Top"=w1442:i32)  [unwired: 2 in, 2 out]
        n1544 = property on="DISCO 5" class="Bool (strict)"() -> ("Left"=w1448:i32, "Top"=w1454:i32)  [unwired: 2 in, 2 out]
        n1545 = property on="DISCO 4" class="Bool (strict)"() -> ("Left"=w380:i32, "Top"=w386:i32)  [unwired: 2 in, 2 out]
        n1546 = property on="DISCO 3" class="Bool (strict)"() -> ("Left"=w369:i32, "Top"=w363:i32)  [unwired: 2 in, 2 out]
        n1547 = property on="DISCO 5" class="Bool (strict)"() -> ("Left"=w357:i32, "Top"=w351:i32)  [unwired: 2 in, 2 out]
        n1548 = Greater Or Equal?(x=w1425, y=0) -> (x >= y?=w1427:bool)
        n1549 = Less Or Equal?(x=w1425, y=160) -> (x <= y?=w1426:bool)
        n1550 = Greater Or Equal?(x=w1419, y=297) -> (x >= y?=w1423:bool)
        n1551 = Less Or Equal?(x=w1419, y=345) -> (x <= y?=w1424:bool)
        n1552 = Greater Or Equal?(x=w1436, y=0) -> (x >= y?=w1434:bool)
        n1553 = Less Or Equal?(x=w1436, y=160) -> (x <= y?=w1435:bool)
        n1554 = Greater Or Equal?(x=w1442, y=345) -> (x >= y?=w1438:bool)
        n1555 = Less Or Equal?(x=w1442, y=410) -> (x <= y?=w1437:bool)
        n1556 = Greater Or Equal?(x=w1448, y=0) -> (x >= y?=w1446:bool)
        n1557 = Less Or Equal?(x=w1448, y=160) -> (x <= y?=w1447:bool)
        n1558 = Greater Or Equal?(x=w1454, y=297) -> (x >= y?=w1450:bool)
        n1559 = Less Or Equal?(x=w1454, y=345) -> (x <= y?=w1449:bool)
        n1560 = Greater Or Equal?(x=w380, y=350) -> (x >= y?=w378:bool)
        n1561 = Less Or Equal?(x=w380, y=500) -> (x <= y?=w379:bool)
        n1562 = Greater Or Equal?(x=w386, y=297) -> (x >= y?=w382:bool)
        n1563 = Less Or Equal?(x=w386, y=345) -> (x <= y?=w381:bool)
        n1564 = Greater Or Equal?(x=w369, y=350) -> (x >= y?=w371:bool)
        n1565 = Less Or Equal?(x=w369, y=500) -> (x <= y?=w370:bool)
        n1566 = Greater Or Equal?(x=w363, y=345) -> (x >= y?=w367:bool)
        n1567 = Less Or Equal?(x=w363, y=410) -> (x <= y?=w368:bool)
        n1568 = Greater Or Equal?(x=w357, y=350) -> (x >= y?=w359:bool)
        n1569 = Less Or Equal?(x=w357, y=500) -> (x <= y?=w358:bool)
        n1570 = Greater Or Equal?(x=w351, y=297) -> (x >= y?=w355:bool)
        n1571 = Less Or Equal?(x=w351, y=345) -> (x <= y?=w356:bool)
        n1572 = And(x=w1427, y=w1426) -> (x .and. y?=w1421:bool)
        n1573 = And(x=w1423, y=w1424) -> (x .and. y?=w1420:bool)
        n1574 = And(x=w1434, y=w1435) -> (x .and. y?=w1440:bool)
        n1575 = And(x=w1438, y=w1437) -> (x .and. y?=w1441:bool)
        n1576 = And(x=w1446, y=w1447) -> (x .and. y?=w1452:bool)
        n1577 = And(x=w1450, y=w1449) -> (x .and. y?=w1453:bool)
        n1578 = And(x=w378, y=w379) -> (x .and. y?=w384:bool)
        n1579 = And(x=w382, y=w381) -> (x .and. y?=w385:bool)
        n1580 = And(x=w371, y=w370) -> (x .and. y?=w365:bool)
        n1581 = And(x=w367, y=w368) -> (x .and. y?=w364:bool)
        n1582 = And(x=w359, y=w358) -> (x .and. y?=w353:bool)
        n1583 = And(x=w355, y=w356) -> (x .and. y?=w352:bool)
        n1584 = And(x=w1421, y=w1420) -> (x .and. y?=w1455:bool)
        n1585 = And(x=w1440, y=w1441) -> (x .and. y?=w1460:bool)
        n1586 = And(x=w1452, y=w1453) -> (x .and. y?=w1456:bool)
        n1587 = And(x=w384, y=w385) -> (x .and. y?=w350:bool)
        n1588 = And(x=w365, y=w364) -> (x .and. y?=w345:bool)
        n1589 = And(x=w353, y=w352) -> (x .and. y?=w349:bool)
        n1590 = And(x=w1460, y=w1455) -> (x .and. y?=w1457:bool)
        n1591 = And(x=w1460, y=w1456) -> (x .and. y?=w1458:bool)
        n1592 = And(x=w345, y=w350) -> (x .and. y?=w348:bool)
        n1593 = And(x=w345, y=w349) -> (x .and. y?=w347:bool)
        n1594 = Compound Arithmetic op=OR(w1457, w1458) -> (w1459:bool)
        n1595 = Compound Arithmetic op=OR(w348, w347) -> (w346:bool)
        n1596 = case shown="False" w1459 {
          frame False {
          }
          frame True {
            n1597 = local write "String"("MOVIMIENTO INCORRECTO" ("String")) -> ()
          }
        }
        n1598 = case shown="False" w346 {
          frame False {
          }
          frame True {
            n1599 = local write "String"("MOVIMIENTO INCORRECTO" ("String")) -> ()
          }
        }
        n1600 = property on="DISCO 4" class="Bool (strict)"() -> ("Left"=w1467:i32, "Top"=w1461:i32)  [unwired: 2 in, 2 out]
        n1601 = property on="DISCO 5" class="Bool (strict)"() -> ("Left"=w1478:i32, "Top"=w1484:i32)  [unwired: 2 in, 2 out]
        n1602 = property on="DISCO 4" class="Bool (strict)"() -> ("Left"=w338:i32, "Top"=w344:i32)  [unwired: 2 in, 2 out]
        n1603 = property on="DISCO 5" class="Bool (strict)"() -> ("Left"=w327:i32, "Top"=w321:i32)  [unwired: 2 in, 2 out]
        n1604 = Greater Or Equal?(x=w1467, y=0) -> (x >= y?=w1469:bool)
        n1605 = Less Or Equal?(x=w1467, y=160) -> (x <= y?=w1468:bool)
        n1606 = Greater Or Equal?(x=w1461, y=345) -> (x >= y?=w1465:bool)
        n1607 = Less Or Equal?(x=w1461, y=410) -> (x <= y?=w1466:bool)
        n1608 = Greater Or Equal?(x=w1478, y=0) -> (x >= y?=w1476:bool)
        n1609 = Less Or Equal?(x=w1478, y=160) -> (x <= y?=w1477:bool)
        n1610 = Greater Or Equal?(x=w1484, y=297) -> (x >= y?=w1480:bool)
        n1611 = Less Or Equal?(x=w1484, y=345) -> (x <= y?=w1479:bool)
        n1612 = Greater Or Equal?(x=w338, y=330) -> (x >= y?=w336:bool)
        n1613 = Less Or Equal?(x=w338, y=500) -> (x <= y?=w337:bool)
        n1614 = Greater Or Equal?(x=w344, y=345) -> (x >= y?=w340:bool)
        n1615 = Less Or Equal?(x=w344, y=410) -> (x <= y?=w339:bool)
        n1616 = Greater Or Equal?(x=w327, y=330) -> (x >= y?=w329:bool)
        n1617 = Less Or Equal?(x=w327, y=500) -> (x <= y?=w328:bool)
        n1618 = Greater Or Equal?(x=w321, y=297) -> (x >= y?=w325:bool)
        n1619 = Less Or Equal?(x=w321, y=345) -> (x <= y?=w326:bool)
        n1620 = And(x=w1469, y=w1468) -> (x .and. y?=w1463:bool)
        n1621 = And(x=w1465, y=w1466) -> (x .and. y?=w1462:bool)
        n1622 = And(x=w1476, y=w1477) -> (x .and. y?=w1482:bool)
        n1623 = And(x=w1480, y=w1479) -> (x .and. y?=w1483:bool)
        n1624 = And(x=w336, y=w337) -> (x .and. y?=w342:bool)
        n1625 = And(x=w340, y=w339) -> (x .and. y?=w343:bool)
        n1626 = And(x=w329, y=w328) -> (x .and. y?=w323:bool)
        n1627 = And(x=w325, y=w326) -> (x .and. y?=w322:bool)
        n1628 = And(x=w1463, y=w1462) -> (x .and. y?=w1485:bool)
        n1629 = And(x=w1482, y=w1483) -> (x .and. y?=w1487:bool)
        n1630 = And(x=w342, y=w343) -> (x .and. y?=w320:bool)
        n1631 = And(x=w323, y=w322) -> (x .and. y?=w318:bool)
        n1632 = And(x=w1485, y=w1487) -> (x .and. y?=w1486:bool)
        n1633 = And(x=w320, y=w318) -> (x .and. y?=w319:bool)
        n1634 = case shown="False" w1486 {
          frame False {
          }
          frame True {
            n1635 = local write "String"("MOVIMIENTO INCORRECTO" ("String")) -> ()
          }
        }
        n1636 = case shown="False" w319 {
          frame False {
          }
          frame True {
            n1637 = local write "String"("MOVIMIENTO INCORRECTO" ("String")) -> ()
          }
        }
        n1638 = property on="DISCO 2" class="Bool (strict)"() -> ("Left"=w120:i32, "Top"=w1675:i32)  [unwired: 2 in, 2 out]
        n1639 = property on="DISCO 2" class="Bool (strict)"() -> ("Left"=w132:i32, "Top"=w126:i32)  [unwired: 2 in, 2 out]
        n1640 = property on="DISCO 3" class="Bool (strict)"() -> ("Left"=w1650:i32, "Top"=w1644:i32)  [unwired: 2 in, 2 out]
        n1641 = property on="DISCO 1" class="Bool (strict)"() -> ("Left"=w1661:i32, "Top"=w1656:i32)  [unwired: 2 in, 2 out]
        n1642 = property on="DISCO 4" class="Bool (strict)"() -> ("Left"=w1633:i32, "Top"=w1639:i32)  [unwired: 2 in, 2 out]
        n1643 = property on="DISCO 5" class="Bool (strict)"() -> ("Left"=w1622:i32, "Top"=w1616:i32)  [unwired: 2 in, 2 out]
        n1644 = property on="DISCO 3" class="Bool (strict)"() -> ("Left"=w154:i32, "Top"=w160:i32)  [unwired: 2 in, 2 out]
        n1645 = property on="DISCO 1" class="Bool (strict)"() -> ("Left"=w143:i32, "Top"=w148:i32)  [unwired: 2 in, 2 out]
        n1646 = property on="DISCO 4" class="Bool (strict)"() -> ("Left"=w171:i32, "Top"=w165:i32)  [unwired: 2 in, 2 out]
        n1647 = property on="DISCO 5" class="Bool (strict)"() -> ("Left"=w182:i32, "Top"=w188:i32)  [unwired: 2 in, 2 out]
        n1648 = Less Or Equal?(x=w120, y=160) -> (x <= y?=w1669:bool)
        n1649 = Greater Or Equal?(x=w1675, y=240) -> (x >= y?=w1671:bool)
        n1650 = Less Or Equal?(x=w1675, y=297) -> (x <= y?=w1670:bool)
        n1651 = Greater Or Equal?(x=w1650, y=0) -> (x >= y?=w1652:bool)
        n1652 = Less Or Equal?(x=w1650, y=160) -> (x <= y?=w1651:bool)
        n1653 = Greater Or Equal?(x=w1644, y=240) -> (x >= y?=w1648:bool)
        n1654 = Less Or Equal?(x=w1644, y=297) -> (x <= y?=w1649:bool)
        n1655 = Greater Or Equal?(x=w1661, y=0) -> (x >= y?=w1663:bool)
        n1656 = Less Or Equal?(x=w1661, y=160) -> (x <= y?=w1662:bool)
        n1657 = Greater Or Equal?(x=w1656, y=297) -> (x >= y?=w1659:bool)
        n1658 = Less Or Equal?(x=w1656, y=345) -> (x <= y?=w1660:bool)
        n1659 = Greater Or Equal?(x=w1633, y=0) -> (x >= y?=w1631:bool)
        n1660 = Less Or Equal?(x=w1633, y=160) -> (x <= y?=w1632:bool)
        n1661 = Greater Or Equal?(x=w1639, y=240) -> (x >= y?=w1635:bool)
        n1662 = Less Or Equal?(x=w1639, y=297) -> (x <= y?=w1634:bool)
        n1663 = Greater Or Equal?(x=w1622, y=0) -> (x >= y?=w1624:bool)
        n1664 = Less Or Equal?(x=w1622, y=160) -> (x <= y?=w1623:bool)
        n1665 = Greater Or Equal?(x=w1616, y=240) -> (x >= y?=w1620:bool)
        n1666 = Less Or Equal?(x=w1616, y=297) -> (x <= y?=w1621:bool)
        n1667 = Greater Or Equal?(x=w120, y=0) -> (x >= y?=w121:bool)
        n1668 = Greater Or Equal?(x=w132, y=350) -> (x >= y?=w134:bool)
        n1669 = Less Or Equal?(x=w132, y=500) -> (x <= y?=w133:bool)
        n1670 = Greater Or Equal?(x=w126, y=240) -> (x >= y?=w130:bool)
        n1671 = Less Or Equal?(x=w126, y=297) -> (x <= y?=w131:bool)
        n1672 = Greater Or Equal?(x=w154, y=350) -> (x >= y?=w152:bool)
        n1673 = Less Or Equal?(x=w154, y=500) -> (x <= y?=w153:bool)
        n1674 = Greater Or Equal?(x=w160, y=240) -> (x >= y?=w156:bool)
        n1675 = Less Or Equal?(x=w160, y=297) -> (x <= y?=w155:bool)
        n1676 = Greater Or Equal?(x=w143, y=350) -> (x >= y?=w141:bool)
        n1677 = Less Or Equal?(x=w143, y=500) -> (x <= y?=w142:bool)
        n1678 = Greater Or Equal?(x=w148, y=297) -> (x >= y?=w145:bool)
        n1679 = Less Or Equal?(x=w148, y=345) -> (x <= y?=w144:bool)
        n1680 = Greater Or Equal?(x=w171, y=350) -> (x >= y?=w173:bool)
        n1681 = Less Or Equal?(x=w171, y=500) -> (x <= y?=w172:bool)
        n1682 = Greater Or Equal?(x=w165, y=240) -> (x >= y?=w169:bool)
        n1683 = Less Or Equal?(x=w165, y=297) -> (x <= y?=w170:bool)
        n1684 = Greater Or Equal?(x=w182, y=350) -> (x >= y?=w180:bool)
        n1685 = Less Or Equal?(x=w182, y=500) -> (x <= y?=w181:bool)
        n1686 = Greater Or Equal?(x=w188, y=240) -> (x >= y?=w184:bool)
        n1687 = Less Or Equal?(x=w188, y=297) -> (x <= y?=w183:bool)
        n1688 = And(x=w121, y=w1669) -> (x .and. y?=w1673:bool)
        n1689 = And(x=w1671, y=w1670) -> (x .and. y?=w1674:bool)
        n1690 = And(x=w1652, y=w1651) -> (x .and. y?=w1646:bool)
        n1691 = And(x=w1648, y=w1649) -> (x .and. y?=w1645:bool)
        n1692 = And(x=w1663, y=w1662) -> (x .and. y?=w1676:bool)
        n1693 = And(x=w1659, y=w1660) -> (x .and. y?=w1657:bool)
        n1694 = And(x=w1631, y=w1632) -> (x .and. y?=w1637:bool)
        n1695 = And(x=w1635, y=w1634) -> (x .and. y?=w1638:bool)
        n1696 = And(x=w1624, y=w1623) -> (x .and. y?=w1618:bool)
        n1697 = And(x=w1620, y=w1621) -> (x .and. y?=w1617:bool)
        n1698 = And(x=w134, y=w133) -> (x .and. y?=w128:bool)
        n1699 = And(x=w130, y=w131) -> (x .and. y?=w127:bool)
        n1700 = And(x=w152, y=w153) -> (x .and. y?=w158:bool)
        n1701 = And(x=w156, y=w155) -> (x .and. y?=w159:bool)
        n1702 = And(x=w141, y=w142) -> (x .and. y?=w125:bool)
        n1703 = And(x=w145, y=w144) -> (x .and. y?=w147:bool)
        n1704 = And(x=w173, y=w172) -> (x .and. y?=w167:bool)
        n1705 = And(x=w169, y=w170) -> (x .and. y?=w166:bool)
        n1706 = And(x=w180, y=w181) -> (x .and. y?=w186:bool)
        n1707 = And(x=w184, y=w183) -> (x .and. y?=w187:bool)
        n1708 = And(x=w1673, y=w1674) -> (x .and. y?=w1643:bool)
        n1709 = And(x=w1646, y=w1645) -> (x .and. y?=w1642:bool)
        n1710 = And(x=w1676, y=w1657) -> (x .and. y?=w1678:bool)
        n1711 = And(x=w1637, y=w1638) -> (x .and. y?=w1615:bool)
        n1712 = And(x=w1618, y=w1617) -> (x .and. y?=w1614:bool)
        n1713 = And(x=w128, y=w127) -> (x .and. y?=w161:bool)
        n1714 = And(x=w158, y=w159) -> (x .and. y?=w162:bool)
        n1715 = And(x=w125, y=w147) -> (x .and. y?=w123:bool)
        n1716 = And(x=w167, y=w166) -> (x .and. y?=w189:bool)
        n1717 = And(x=w186, y=w187) -> (x .and. y?=w190:bool)
        n1718 = And(x=w1678, y=w1643) -> (x .and. y?=w1641:bool)
        n1719 = And(x=w1678, y=w1642) -> (x .and. y?=w1640:bool)
        n1720 = And(x=w1678, y=w1615) -> (x .and. y?=w1613:bool)
        n1721 = And(x=w1678, y=w1614) -> (x .and. y?=w1612:bool)
        n1722 = And(x=w123, y=w161) -> (x .and. y?=w163:bool)
        n1723 = And(x=w123, y=w162) -> (x .and. y?=w164:bool)
        n1724 = And(x=w123, y=w189) -> (x .and. y?=w191:bool)
        n1725 = And(x=w123, y=w190) -> (x .and. y?=w192:bool)
        n1726 = Compound Arithmetic op=OR(w1641, w1640, w1613, w1612) -> (w1677:bool)
        n1727 = Compound Arithmetic op=OR(w163, w164, w191, w192) -> (w124:bool)
        n1728 = case shown="False" w1677 {
          frame False {
          }
          frame True {
            n1729 = local write "String"("MOVIMIENTO INCORRECTO" ("String")) -> ()
          }
        }
        n1730 = case shown="False" w124 {
          frame False {
          }
          frame True {
            n1731 = local write "String"("MOVIMIENTO INCORRECTO" ("String")) -> ()
          }
        }
        n1732 = property on="DISCO 2" class="Bool (strict)"() -> ("Left"=w1573:i32, "Top"=w1579:i32)  [unwired: 2 in, 2 out]
        n1733 = property on="DISCO 4" class="Bool (strict)"() -> ("Left"=w1585:i32, "Top"=w1591:i32)  [unwired: 2 in, 2 out]
        n1734 = property on="DISCO 2" class="Bool (strict)"() -> ("Left"=w231:i32, "Top"=w225:i32)  [unwired: 2 in, 2 out]
        n1735 = property on="DISCO 4" class="Bool (strict)"() -> ("Left"=w219:i32, "Top"=w213:i32)  [unwired: 2 in, 2 out]
        n1736 = property on="DISCO 5" class="Bool (strict)"() -> ("Left"=w1603:i32, "Top"=w1597:i32)  [unwired: 2 in, 2 out]
        n1737 = property on="DISCO 3" class="Bool (strict)"() -> ("Left"=w1562:i32, "Top"=w1556:i32)  [unwired: 2 in, 2 out]
        n1738 = property on="DISCO 5" class="Bool (strict)"() -> ("Left"=w201:i32, "Top"=w207:i32)  [unwired: 2 in, 2 out]
        n1739 = property on="DISCO 3" class="Bool (strict)"() -> ("Left"=w242:i32, "Top"=w248:i32)  [unwired: 2 in, 2 out]
        n1740 = Greater Or Equal?(x=w1573, y=0) -> (x >= y?=w1571:bool)
        n1741 = Less Or Equal?(x=w1573, y=160) -> (x <= y?=w1572:bool)
        n1742 = Greater Or Equal?(x=w1579, y=297) -> (x >= y?=w1575:bool)
        n1743 = Greater Or Equal?(x=w1585, y=0) -> (x >= y?=w1583:bool)
        n1744 = Less Or Equal?(x=w1585, y=160) -> (x <= y?=w1584:bool)
        n1745 = Greater Or Equal?(x=w1591, y=240) -> (x >= y?=w1587:bool)
        n1746 = Greater Or Equal?(x=w231, y=350) -> (x >= y?=w233:bool)
        n1747 = Less Or Equal?(x=w231, y=500) -> (x <= y?=w232:bool)
        n1748 = Greater Or Equal?(x=w225, y=297) -> (x >= y?=w229:bool)
        n1749 = Greater Or Equal?(x=w219, y=350) -> (x >= y?=w221:bool)
        n1750 = Less Or Equal?(x=w219, y=500) -> (x <= y?=w220:bool)
        n1751 = Greater Or Equal?(x=w213, y=240) -> (x >= y?=w217:bool)
        n1752 = Greater Or Equal?(x=w1603, y=0) -> (x >= y?=w1605:bool)
        n1753 = Less Or Equal?(x=w1603, y=160) -> (x <= y?=w1604:bool)
        n1754 = Greater Or Equal?(x=w1597, y=240) -> (x >= y?=w1601:bool)
        n1755 = Greater Or Equal?(x=w1562, y=0) -> (x >= y?=w1564:bool)
        n1756 = Less Or Equal?(x=w1562, y=160) -> (x <= y?=w1563:bool)
        n1757 = Greater Or Equal?(x=w1556, y=240) -> (x >= y?=w1560:bool)
        n1758 = Greater Or Equal?(x=w201, y=350) -> (x >= y?=w199:bool)
        n1759 = Less Or Equal?(x=w201, y=500) -> (x <= y?=w200:bool)
        n1760 = Greater Or Equal?(x=w207, y=240) -> (x >= y?=w203:bool)
        n1761 = Greater Or Equal?(x=w242, y=350) -> (x >= y?=w240:bool)
        n1762 = Less Or Equal?(x=w242, y=500) -> (x <= y?=w241:bool)
        n1763 = Greater Or Equal?(x=w248, y=240) -> (x >= y?=w244:bool)
        n1764 = Less Or Equal?(x=w1579, y=345) -> (x <= y?=w1574:bool)
        n1765 = Less Or Equal?(x=w1591, y=297) -> (x <= y?=w1586:bool)
        n1766 = Less Or Equal?(x=w225, y=345) -> (x <= y?=w230:bool)
        n1767 = Less Or Equal?(x=w213, y=297) -> (x <= y?=w218:bool)
        n1768 = Less Or Equal?(x=w1597, y=297) -> (x <= y?=w1602:bool)
        n1769 = And(x=w1571, y=w1572) -> (x .and. y?=w1577:bool)
        n1770 = And(x=w1575, y=w1574) -> (x .and. y?=w1578:bool)
        n1771 = Less Or Equal?(x=w1556, y=297) -> (x <= y?=w1561:bool)
        n1772 = Less Or Equal?(x=w207, y=297) -> (x <= y?=w202:bool)
        n1773 = And(x=w1583, y=w1584) -> (x .and. y?=w1589:bool)
        n1774 = And(x=w1587, y=w1586) -> (x .and. y?=w1590:bool)
        n1775 = And(x=w233, y=w232) -> (x .and. y?=w227:bool)
        n1776 = And(x=w229, y=w230) -> (x .and. y?=w226:bool)
        n1777 = Less Or Equal?(x=w248, y=297) -> (x <= y?=w243:bool)
        n1778 = And(x=w221, y=w220) -> (x .and. y?=w215:bool)
        n1779 = And(x=w217, y=w218) -> (x .and. y?=w214:bool)
        n1780 = And(x=w1605, y=w1604) -> (x .and. y?=w1599:bool)
        n1781 = And(x=w1601, y=w1602) -> (x .and. y?=w1598:bool)
        n1782 = And(x=w1564, y=w1563) -> (x .and. y?=w1558:bool)
        n1783 = And(x=w1560, y=w1561) -> (x .and. y?=w1557:bool)
        n1784 = And(x=w199, y=w200) -> (x .and. y?=w205:bool)
        n1785 = And(x=w203, y=w202) -> (x .and. y?=w206:bool)
        n1786 = And(x=w240, y=w241) -> (x .and. y?=w246:bool)
        n1787 = And(x=w244, y=w243) -> (x .and. y?=w247:bool)
        n1788 = And(x=w1577, y=w1578) -> (x .and. y?=w1609:bool)
        n1789 = And(x=w1589, y=w1590) -> (x .and. y?=w1593:bool)
        n1790 = And(x=w227, y=w226) -> (x .and. y?=w195:bool)
        n1791 = And(x=w215, y=w214) -> (x .and. y?=w211:bool)
        n1792 = And(x=w1599, y=w1598) -> (x .and. y?=w1610:bool)
        n1793 = And(x=w1558, y=w1557) -> (x .and. y?=w1592:bool)
        n1794 = And(x=w205, y=w206) -> (x .and. y?=w194:bool)
        n1795 = And(x=w246, y=w247) -> (x .and. y?=w212:bool)
        n1796 = And(x=w1609, y=w1610) -> (x .and. y?=w1611:bool)
        n1797 = And(x=w195, y=w194) -> (x .and. y?=w193:bool)
        n1798 = And(x=w1609, y=w1593) -> (x .and. y?=w1595:bool)
        n1799 = And(x=w1609, y=w1592) -> (x .and. y?=w1594:bool)
        n1800 = And(x=w195, y=w211) -> (x .and. y?=w209:bool)
        n1801 = And(x=w195, y=w212) -> (x .and. y?=w210:bool)
        n1802 = Compound Arithmetic op=OR(w1594, w1595, w1611) -> (w1596:bool)
        n1803 = Compound Arithmetic op=OR(w210, w209, w193) -> (w208:bool)
        n1804 = case shown="False" w1596 {
          frame False {
          }
          frame True {
            n1805 = local write "String"("MOVIMIENTO INCORRECTO" ("String")) -> ()
          }
        }
        n1806 = case shown="False" w208 {
          frame False {
          }
          frame True {
            n1807 = local write "String"("MOVIMIENTO INCORRECTO" ("String")) -> ()
          }
        }
        n1808 = property on="DISCO 4" class="Bool (strict)"() -> ("Left"=w1549:i32, "Top"=w1555:i32)  [unwired: 2 in, 2 out]
        n1809 = property on="DISCO 3" class="Bool (strict)"() -> ("Left"=w1539:i32, "Top"=w1533:i32)  [unwired: 2 in, 2 out]
        n1810 = property on="DISCO 5" class="Bool (strict)"() -> ("Left"=w1527:i32, "Top"=w1521:i32)  [unwired: 2 in, 2 out]
        n1811 = property on="DISCO 4" class="Bool (strict)"() -> ("Left"=w255:i32, "Top"=w249:i32)  [unwired: 2 in, 2 out]
        n1812 = property on="DISCO 3" class="Bool (strict)"() -> ("Left"=w266:i32, "Top"=w272:i32)  [unwired: 2 in, 2 out]
        n1813 = property on="DISCO 5" class="Bool (strict)"() -> ("Left"=w278:i32, "Top"=w284:i32)  [unwired: 2 in, 2 out]
        n1814 = Greater Or Equal?(x=w1549, y=0) -> (x >= y?=w1547:bool)
        n1815 = Less Or Equal?(x=w1549, y=160) -> (x <= y?=w1548:bool)
        n1816 = Greater Or Equal?(x=w1555, y=240) -> (x >= y?=w1551:bool)
        n1817 = Less Or Equal?(x=w1555, y=297) -> (x <= y?=w1550:bool)
        n1818 = Greater Or Equal?(x=w1539, y=0) -> (x >= y?=w1541:bool)
        n1819 = Less Or Equal?(x=w1539, y=160) -> (x <= y?=w1540:bool)
        n1820 = Greater Or Equal?(x=w1533, y=297) -> (x >= y?=w1537:bool)
        n1821 = Less Or Equal?(x=w1533, y=345) -> (x <= y?=w1538:bool)
        n1822 = Greater Or Equal?(x=w1527, y=0) -> (x >= y?=w1529:bool)
        n1823 = Less Or Equal?(x=w1527, y=160) -> (x <= y?=w1528:bool)
        n1824 = Greater Or Equal?(x=w1521, y=240) -> (x >= y?=w1525:bool)
        n1825 = Less Or Equal?(x=w1521, y=297) -> (x <= y?=w1526:bool)
        n1826 = Greater Or Equal?(x=w255, y=350) -> (x >= y?=w257:bool)
        n1827 = Less Or Equal?(x=w255, y=500) -> (x <= y?=w256:bool)
        n1828 = Greater Or Equal?(x=w249, y=240) -> (x >= y?=w253:bool)
        n1829 = Less Or Equal?(x=w249, y=297) -> (x <= y?=w254:bool)
        n1830 = Greater Or Equal?(x=w266, y=350) -> (x >= y?=w264:bool)
        n1831 = Less Or Equal?(x=w266, y=500) -> (x <= y?=w265:bool)
        n1832 = Greater Or Equal?(x=w272, y=297) -> (x >= y?=w268:bool)
        n1833 = Less Or Equal?(x=w272, y=345) -> (x <= y?=w267:bool)
        n1834 = Greater Or Equal?(x=w278, y=350) -> (x >= y?=w276:bool)
        n1835 = Less Or Equal?(x=w278, y=500) -> (x <= y?=w277:bool)
        n1836 = Greater Or Equal?(x=w284, y=240) -> (x >= y?=w280:bool)
        n1837 = Less Or Equal?(x=w284, y=297) -> (x <= y?=w279:bool)
        n1838 = And(x=w1547, y=w1548) -> (x .and. y?=w1553:bool)
        n1839 = And(x=w1551, y=w1550) -> (x .and. y?=w1554:bool)
        n1840 = And(x=w1541, y=w1540) -> (x .and. y?=w1535:bool)
        n1841 = And(x=w1537, y=w1538) -> (x .and. y?=w1534:bool)
        n1842 = And(x=w1529, y=w1528) -> (x .and. y?=w1523:bool)
        n1843 = And(x=w1525, y=w1526) -> (x .and. y?=w1522:bool)
        n1844 = And(x=w257, y=w256) -> (x .and. y?=w251:bool)
        n1845 = And(x=w253, y=w254) -> (x .and. y?=w250:bool)
        n1846 = And(x=w264, y=w265) -> (x .and. y?=w270:bool)
        n1847 = And(x=w268, y=w267) -> (x .and. y?=w271:bool)
        n1848 = And(x=w276, y=w277) -> (x .and. y?=w282:bool)
        n1849 = And(x=w280, y=w279) -> (x .and. y?=w283:bool)
        n1850 = And(x=w1553, y=w1554) -> (x .and. y?=w1520:bool)
        n1851 = And(x=w1535, y=w1534) -> (x .and. y?=w1515:bool)
        n1852 = And(x=w1523, y=w1522) -> (x .and. y?=w1519:bool)
        n1853 = And(x=w251, y=w250) -> (x .and. y?=w285:bool)
        n1854 = And(x=w270, y=w271) -> (x .and. y?=w290:bool)
        n1855 = And(x=w282, y=w283) -> (x .and. y?=w286:bool)
        n1856 = And(x=w1515, y=w1520) -> (x .and. y?=w1518:bool)
        n1857 = And(x=w1515, y=w1519) -> (x .and. y?=w1517:bool)
        n1858 = And(x=w290, y=w285) -> (x .and. y?=w287:bool)
        n1859 = And(x=w290, y=w286) -> (x .and. y?=w288:bool)
        n1860 = Compound Arithmetic op=OR(w1518, w1517) -> (w1516:bool)
        n1861 = Compound Arithmetic op=OR(w287, w288) -> (w289:bool)
        n1862 = case shown="False" w1516 {
          frame False {
          }
          frame True {
            n1863 = local write "String"("MOVIMIENTO INCORRECTO" ("String")) -> ()
          }
        }
        n1864 = case shown="False" w289 {
          frame False {
          }
          frame True {
            n1865 = local write "String"("MOVIMIENTO INCORRECTO" ("String")) -> ()
          }
        }
        n1866 = property on="DISCO 4" class="Bool (strict)"() -> ("Left"=w1508:i32, "Top"=w1514:i32)  [unwired: 2 in, 2 out]
        n1867 = property on="DISCO 5" class="Bool (strict)"() -> ("Left"=w1497:i32, "Top"=w1491:i32)  [unwired: 2 in, 2 out]
        n1868 = property on="DISCO 4" class="Bool (strict)"() -> ("Left"=w297:i32, "Top"=w291:i32)  [unwired: 2 in, 2 out]
        n1869 = property on="DISCO 5" class="Bool (strict)"() -> ("Left"=w308:i32, "Top"=w314:i32)  [unwired: 2 in, 2 out]
        n1870 = Greater Or Equal?(x=w1508, y=0) -> (x >= y?=w1506:bool)
        n1871 = Less Or Equal?(x=w1508, y=160) -> (x <= y?=w1507:bool)
        n1872 = Greater Or Equal?(x=w1514, y=297) -> (x >= y?=w1510:bool)
        n1873 = Less Or Equal?(x=w1514, y=345) -> (x <= y?=w1509:bool)
        n1874 = Greater Or Equal?(x=w1497, y=0) -> (x >= y?=w1499:bool)
        n1875 = Less Or Equal?(x=w1497, y=160) -> (x <= y?=w1498:bool)
        n1876 = Greater Or Equal?(x=w1491, y=240) -> (x >= y?=w1495:bool)
        n1877 = Less Or Equal?(x=w1491, y=297) -> (x <= y?=w1496:bool)
        n1878 = Greater Or Equal?(x=w297, y=330) -> (x >= y?=w299:bool)
        n1879 = Less Or Equal?(x=w297, y=500) -> (x <= y?=w298:bool)
        n1880 = Greater Or Equal?(x=w291, y=297) -> (x >= y?=w295:bool)
        n1881 = Less Or Equal?(x=w291, y=345) -> (x <= y?=w296:bool)
        n1882 = Greater Or Equal?(x=w308, y=330) -> (x >= y?=w306:bool)
        n1883 = Less Or Equal?(x=w308, y=500) -> (x <= y?=w307:bool)
        n1884 = Greater Or Equal?(x=w314, y=240) -> (x >= y?=w310:bool)
        n1885 = Less Or Equal?(x=w314, y=297) -> (x <= y?=w309:bool)
        n1886 = And(x=w1506, y=w1507) -> (x .and. y?=w1512:bool)
        n1887 = And(x=w1510, y=w1509) -> (x .and. y?=w1513:bool)
        n1888 = And(x=w1499, y=w1498) -> (x .and. y?=w1493:bool)
        n1889 = And(x=w1495, y=w1496) -> (x .and. y?=w1492:bool)
        n1890 = And(x=w299, y=w298) -> (x .and. y?=w293:bool)
        n1891 = And(x=w295, y=w296) -> (x .and. y?=w292:bool)
        n1892 = And(x=w306, y=w307) -> (x .and. y?=w312:bool)
        n1893 = And(x=w310, y=w309) -> (x .and. y?=w313:bool)
        n1894 = And(x=w1512, y=w1513) -> (x .and. y?=w1490:bool)
        n1895 = And(x=w1493, y=w1492) -> (x .and. y?=w1488:bool)
        n1896 = And(x=w293, y=w292) -> (x .and. y?=w315:bool)
        n1897 = And(x=w312, y=w313) -> (x .and. y?=w317:bool)
        n1898 = And(x=w1490, y=w1488) -> (x .and. y?=w1489:bool)
        n1899 = And(x=w315, y=w317) -> (x .and. y?=w316:bool)
        n1900 = case shown="False" w1489 {
          frame False {
          }
          frame True {
            n1901 = local write "String"("MOVIMIENTO INCORRECTO" ("String")) -> ()
          }
        }
        n1902 = case shown="False" w316 {
          frame False {
          }
          frame True {
            n1903 = local write "String"("MOVIMIENTO INCORRECTO" ("String")) -> ()
          }
        }
      }
      event "DISCO 1", "DISCO 2", "DISCO 5", "DISCO 4", "DISCO 3": Mouse Move {
        n1904 = event-data() -> ("CtlRef"=w2712:refnum<vi>, "Coords"=w2710:T4)  [unwired: 1 in, 3 out]
        n1905 = local read "Boolean"() -> (w2711:bool)
        n1906 = case shown="True" w2711 {
          tunnel: w2710 -> [_ w2718]
          tunnel: w2712 -> [_ w2717]
          frame False {
          }
          frame True {
            n1907 = property class="Bool (strict)"(reference=w2717) -> ("Bounds"=w2713:T1)  [unwired: 1 in, 2 out]
            n1908 = Divide(x=w2713, y=T1 {"Width"=2, "Height"=2}) -> (x/y=w2715:cluster{"Width":dbl, "Height":dbl})
            n1909 = Subtract(x=w2718, y=w2715) -> (x-y=w2714:cluster{dbl, dbl})
            n1910 = property class="Bool (strict)"(reference=w2717, "Position"=w2714) -> ()  [unwired: 1 in, 2 out]
          }
        }
      }
      event "DISCO 1", "DISCO 2", "DISCO 5", "DISCO 4", "DISCO 3": Mouse Down {
        n1911 = event-data() -> ("CtlRef"=w2722:refnum<vi>, "Coords"=w2727:T4, "Button"=w2720:u16)  [unwired: 1 in, 5 out]
        n1912 = local write "Boolean"(TRUE ("Boolean")) -> ()
        n1913 = disable-structure shown="Disabled" {
          frame Disabled {
            n1914 = local write "Boolean 2"(FALSE ("Boolean 2")) -> ()
          }
          frame Enabled {
          }
        }
        n1915 = case shown="1" w2720 {
          tunnel: [_ w2731] -> w2721
          frame 0, Default {
          }
          frame 1 {
            n1916 = local read "Numeric 2"() -> (w2730:dbl)
            n1917 = local write "String"("" ("String")) -> ()
            n1918 = Increment(x=w2730) -> (x+1=w2731:dbl)
          }
        }
        "Numeric 2" <- w2721
        n1919 = property class="Bool (strict)"(reference=w2722) -> ("Bounds"=w2723:T1)  [unwired: 1 in, 2 out]
        n1920 = Divide(x=w2723, y=T1 {"Width"=2, "Height"=2}) -> (x/y=w2725:cluster{"Width":dbl, "Height":dbl})
        n1921 = Subtract(x=w2727, y=w2725) -> (x-y=w2724:cluster{dbl, dbl})
        n1922 = property class="Bool (strict)"(reference=w2722, "Position"=w2724) -> ()  [unwired: 1 in, 2 out]
      }
      event Value Change {
        n1923 = event-data() -> ()  [unwired: 1 in, 6 out]
        n1924 = case shown="\"2\", Default" "NUMERO DISCOS" {
          frame "2", Default {
            n1925 = disable-structure shown="Disabled" {
              frame Disabled {
                (unwired) T3 {"Left"=-32, "Top"=489} ("Position")
                (unwired) T3 {"Left"=-22, "Top"=441} ("Position")
                (unwired) T3 {"Left"=-13, "Top"=393} ("Position")
                n1926 = property on="DISCO 3" class="Bool (strict)" props=["Position"]() -> ()  [unwired: 3 in, 2 out]
                n1927 = property on="DISCO 4" class="Bool (strict)" props=["Position"]() -> ()  [unwired: 3 in, 2 out]
                n1928 = property on="DISCO 5" class="Bool (strict)" props=["Position"]() -> ()  [unwired: 3 in, 2 out]
              }
              frame Enabled {
              }
            }
            n1929 = property on="DISCO 1" class="Bool (strict)"("Position"=T3 {"Left"=753, "Top"=441}) -> ()  [unwired: 2 in, 2 out]
            n1930 = property on="DISCO 2" class="Bool (strict)"("Position"=T3 {"Left"=741, "Top"=489}) -> ()  [unwired: 2 in, 2 out]
            n1931 = local write "Numeric 2"(0.0 ("Numeric 2")) -> ()
            n1932 = Scale By Power Of 2(n=i16 2, x=ext 1.0) -> (x*2^n=w2738:ext)
            n1933 = Subtract(x=w2738, y=ext 1.0) -> (x-y=w2740:ext)
            n1934 = local write "x-y"(w2740) -> ()
            n1935 = property on="DISCO 4" class="Bool (strict)"("Visible"=FALSE) -> ()  [unwired: 2 in, 2 out]
            n1936 = property on="DISCO 2" class="Bool (strict)"("Visible"=TRUE) -> ()  [unwired: 2 in, 2 out]
            n1937 = property on="DISCO 3" class="Bool (strict)"("Visible"=FALSE) -> ()  [unwired: 2 in, 2 out]
            n1938 = property on="DISCO 1" class="Bool (strict)"("Visible"=TRUE) -> ()  [unwired: 2 in, 2 out]
            n1939 = property on="DISCO 5" class="Bool (strict)"("Visible"=FALSE) -> ()  [unwired: 2 in, 2 out]
          }
          frame "3" {
            n1940 = disable-structure shown="Disabled" {
              frame Disabled {
                n1941 = property on="DISCO 4" class="Bool (strict)"("Position"=T3 {"Left"=-22, "Top"=441}) -> ()  [unwired: 2 in, 2 out]
                n1942 = property on="DISCO 5" class="Bool (strict)"("Position"=T3 {"Left"=-32, "Top"=489}) -> ()  [unwired: 2 in, 2 out]
              }
              frame Enabled {
              }
            }
            n1943 = property on="DISCO 1" class="Bool (strict)"("Position"=T3 {"Left"=753, "Top"=393}) -> ()  [unwired: 2 in, 2 out]
            n1944 = property on="DISCO 2" class="Bool (strict)"("Position"=T3 {"Left"=741, "Top"=441}) -> ()  [unwired: 2 in, 2 out]
            n1945 = property on="DISCO 3" class="Bool (strict)"("Position"=T3 {"Left"=729, "Top"=489}) -> ()  [unwired: 2 in, 2 out]
            n1946 = local write "Numeric 2"(0.0 ("Numeric 2")) -> ()
            n1947 = Scale By Power Of 2(n=i16 3, x=ext 1.0) -> (x*2^n=w2752:ext)
            n1948 = Subtract(x=w2752, y=ext 1.0) -> (x-y=w2754:ext)
            n1949 = local write "x-y"(w2754) -> ()
            n1950 = property on="DISCO 4" class="Bool (strict)"("Visible"=FALSE) -> ()  [unwired: 2 in, 2 out]
            n1951 = property on="DISCO 2" class="Bool (strict)"("Visible"=TRUE) -> ()  [unwired: 2 in, 2 out]
            n1952 = property on="DISCO 3" class="Bool (strict)"("Visible"=TRUE) -> ()  [unwired: 2 in, 2 out]
            n1953 = property on="DISCO 1" class="Bool (strict)"("Visible"=TRUE) -> ()  [unwired: 2 in, 2 out]
            n1954 = property on="DISCO 5" class="Bool (strict)"("Visible"=FALSE) -> ()  [unwired: 2 in, 2 out]
          }
          frame "4" {
            n1955 = disable-structure shown="Disabled" {
              frame Disabled {
                n1956 = property on="DISCO 5" class="Bool (strict)"("Position"=T3 {"Left"=-32, "Top"=489}) -> ()  [unwired: 2 in, 2 out]
              }
              frame Enabled {
              }
            }
            n1957 = property on="DISCO 1" class="Bool (strict)"("Position"=T3 {"Left"=753, "Top"=345}) -> ()  [unwired: 2 in, 2 out]
            n1958 = property on="DISCO 2" class="Bool (strict)"("Position"=T3 {"Left"=741, "Top"=393}) -> ()  [unwired: 2 in, 2 out]
            n1959 = property on="DISCO 3" class="Bool (strict)"("Position"=T3 {"Left"=729, "Top"=441}) -> ()  [unwired: 2 in, 2 out]
            n1960 = property on="DISCO 4" class="Bool (strict)"("Position"=T3 {"Left"=717, "Top"=489}) -> ()  [unwired: 2 in, 2 out]
            n1961 = local write "Numeric 2"(0.0 ("Numeric 2")) -> ()
            n1962 = Scale By Power Of 2(n=i16 4, x=ext 1.0) -> (x*2^n=w2769:ext)
            n1963 = Subtract(x=w2769, y=ext 1.0) -> (x-y=w2771:ext)
            n1964 = local write "x-y"(w2771) -> ()
            n1965 = property on="DISCO 4" class="Bool (strict)"("Visible"=TRUE) -> ()  [unwired: 2 in, 2 out]
            n1966 = property on="DISCO 2" class="Bool (strict)"("Visible"=TRUE) -> ()  [unwired: 2 in, 2 out]
            n1967 = property on="DISCO 3" class="Bool (strict)"("Visible"=TRUE) -> ()  [unwired: 2 in, 2 out]
            n1968 = property on="DISCO 1" class="Bool (strict)"("Visible"=TRUE) -> ()  [unwired: 2 in, 2 out]
            n1969 = property on="DISCO 5" class="Bool (strict)"("Visible"=FALSE) -> ()  [unwired: 2 in, 2 out]
          }
          frame "5" {
            n1970 = property on="DISCO 1" class="Bool (strict)"("Position"=T3 {"Left"=753, "Top"=295}) -> ()  [unwired: 2 in, 2 out]
            n1971 = property on="DISCO 2" class="Bool (strict)"("Position"=T3 {"Left"=741, "Top"=344}) -> ()  [unwired: 2 in, 2 out]
            n1972 = property on="DISCO 3" class="Bool (strict)"("Position"=T3 {"Left"=729, "Top"=393}) -> ()  [unwired: 2 in, 2 out]
            n1973 = property on="DISCO 4" class="Bool (strict)"("Position"=T3 {"Left"=717, "Top"=442}) -> ()  [unwired: 2 in, 2 out]
            n1974 = property on="DISCO 5" class="Bool (strict)"("Position"=T3 {"Left"=705, "Top"=491}) -> ()  [unwired: 2 in, 2 out]
            n1975 = Scale By Power Of 2(n=i16 5, x=ext 1.0) -> (x*2^n=w2787:ext)
            n1976 = local write "Numeric 2"(0.0 ("Numeric 2")) -> ()
            n1977 = Subtract(x=w2787, y=ext 1.0) -> (x-y=w2784:ext)
            n1978 = local write "x-y"(w2784) -> ()
            n1979 = property on="DISCO 4" class="Bool (strict)"("Visible"=TRUE) -> ()  [unwired: 2 in, 2 out]
            n1980 = property on="DISCO 2" class="Bool (strict)"("Visible"=TRUE) -> ()  [unwired: 2 in, 2 out]
            n1981 = property on="DISCO 3" class="Bool (strict)"("Visible"=TRUE) -> ()  [unwired: 2 in, 2 out]
            n1982 = property on="DISCO 1" class="Bool (strict)"("Visible"=TRUE) -> ()  [unwired: 2 in, 2 out]
            n1983 = property on="DISCO 5" class="Bool (strict)"("Visible"=TRUE) -> ()  [unwired: 2 in, 2 out]
          }
        }
      }
    }
  }
  n1984 = disable-structure shown="Disabled" {
    frame Disabled {
      n1985 = property on="DISCO 4" class="Bool (strict)"() -> ("Position"=w2796:T3)  [unwired: 2 in, 2 out]
      n1986 = property on="DISCO 5" class="Bool (strict)"() -> ("Position"=w2795:T3)  [unwired: 2 in, 2 out]
      n1987 = Select(t=w2795, s="s 2", f=w2796) -> (s? t:f=w2797:T3)
      n1988 = property on="Property Node" class="Pane"("Position"=w2797) -> ()  [unwired: 2 in, 2 out]
    }
    frame Enabled {
    }
  }
  n1989 = local write "Numeric 2"(0.0 ("Numeric 2")) -> ()
  n1990 = disable-structure shown="Disabled" {
    frame Disabled {
      (unwired) T3 {"Left"=705, "Top"=491} ("Position")
      (unwired) T3 {"Left"=717, "Top"=442} ("Position")
      (unwired) T3 {"Left"=729, "Top"=393} ("Position")
      (unwired) T3 {"Left"=741, "Top"=344} ("Position")
      (unwired) T3 {"Left"=753, "Top"=295} ("Position")
      n1991 = property on="DISCO 1" class="Bool (strict)"("Position"=T3 {"Left"=7, "Top"=393}) -> ()  [unwired: 2 in, 2 out]
      n1992 = property on="DISCO 2" class="Bool (strict)"("Position"=T3 {"Left"=-2, "Top"=441}) -> ()  [unwired: 2 in, 2 out]
      n1993 = property on="DISCO 3" class="Bool (strict)"("Position"=T3 {"Left"=-13, "Top"=489}) -> ()  [unwired: 2 in, 2 out]
      n1994 = property on="DISCO 1" class="Bool (strict)"("Position"=T3 {"Left"=7, "Top"=441}) -> ()  [unwired: 2 in, 2 out]
      n1995 = property on="DISCO 2" class="Bool (strict)"("Position"=T3 {"Left"=-2, "Top"=489}) -> ()  [unwired: 2 in, 2 out]
      n1996 = property on="DISCO 1" class="Bool (strict)"("Position"=T3 {"Left"=7, "Top"=297}) -> ()  [unwired: 2 in, 2 out]
      n1997 = property on="DISCO 2" class="Bool (strict)"("Position"=T3 {"Left"=-2, "Top"=345}) -> ()  [unwired: 2 in, 2 out]
      n1998 = property on="DISCO 3" class="Bool (strict)"("Position"=T3 {"Left"=-13, "Top"=393}) -> ()  [unwired: 2 in, 2 out]
      n1999 = property on="DISCO 4" class="Bool (strict)"("Position"=T3 {"Left"=-22, "Top"=441}) -> ()  [unwired: 2 in, 2 out]
      n2000 = property on="DISCO 5" class="Bool (strict)"("Position"=T3 {"Left"=-32, "Top"=489}) -> ()  [unwired: 2 in, 2 out]
      n2001 = property on="DISCO 1" class="Bool (strict)"("Position"=T3 {"Left"=7, "Top"=345}) -> ()  [unwired: 2 in, 2 out]
      n2002 = property on="DISCO 2" class="Bool (strict)"("Position"=T3 {"Left"=-2, "Top"=393}) -> ()  [unwired: 2 in, 2 out]
      n2003 = property on="DISCO 3" class="Bool (strict)"("Position"=T3 {"Left"=-13, "Top"=441}) -> ()  [unwired: 2 in, 2 out]
      n2004 = property on="DISCO 4" class="Bool (strict)"("Position"=T3 {"Left"=-22, "Top"=489}) -> ()  [unwired: 2 in, 2 out]
      n2005 = property on="DISCO 1" class="Bool (strict)" props=["Position"]() -> ()  [unwired: 3 in, 2 out]
      n2006 = property on="DISCO 2" class="Bool (strict)" props=["Position"]() -> ()  [unwired: 3 in, 2 out]
      n2007 = property on="DISCO 3" class="Bool (strict)" props=["Position"]() -> ()  [unwired: 3 in, 2 out]
      n2008 = property on="DISCO 4" class="Bool (strict)" props=["Position"]() -> ()  [unwired: 3 in, 2 out]
      n2009 = property on="DISCO 5" class="Bool (strict)" props=["Position"]() -> ()  [unwired: 3 in, 2 out]
    }
    frame Enabled {
    }
  }
  n2010 = disable-structure shown="Disabled" {
    frame Disabled {
      n2011 = disable-structure shown="Disabled" {
        frame Disabled {
          (unwired) T3 {"Left"=-32, "Top"=489} ("Position")
          (unwired) T3 {"Left"=-22, "Top"=441} ("Position")
          (unwired) T3 {"Left"=-13, "Top"=393} ("Position")
          n2012 = property on="DISCO 3" class="Bool (strict)" props=["Position"]() -> ()  [unwired: 3 in, 2 out]
          n2013 = property on="DISCO 4" class="Bool (strict)" props=["Position"]() -> ()  [unwired: 3 in, 2 out]
          n2014 = property on="DISCO 5" class="Bool (strict)" props=["Position"]() -> ()  [unwired: 3 in, 2 out]
        }
        frame Enabled {
        }
      }
      n2015 = property on="DISCO 1" class="Bool (strict)"("Position"=T3 {"Left"=7, "Top"=441}) -> ()  [unwired: 2 in, 2 out]
      n2016 = property on="DISCO 2" class="Bool (strict)"("Position"=T3 {"Left"=-2, "Top"=489}) -> ()  [unwired: 2 in, 2 out]
      n2017 = property class="Bool (strict)" props=["Position"]() -> ()  [unwired: 3 in, 2 out]
      n2018 = property on="DISCO 4" class="Bool (strict)"("Visible"=FALSE) -> ()  [unwired: 2 in, 2 out]
      n2019 = property on="DISCO 2" class="Bool (strict)"("Visible"=TRUE) -> ()  [unwired: 2 in, 2 out]
      n2020 = property on="DISCO 3" class="Bool (strict)"("Visible"=FALSE) -> ()  [unwired: 2 in, 2 out]
      n2021 = property on="DISCO 1" class="Bool (strict)"("Visible"=TRUE) -> ()  [unwired: 2 in, 2 out]
      n2022 = property on="DISCO 5" class="Bool (strict)"("Visible"=FALSE) -> ()  [unwired: 2 in, 2 out]
    }
    frame Enabled {
    }
  }
